vi "ControlProgram5.6 (DON'T USE ME YET!).vi"() -> ()   [LabVIEW 2016]
uses:
  <vilib>/Utility/error.llb/DialogType.ctl
  <vilib>/Utility/miscctls.llb/LVPoint32TypeDef.ctl
  <vilib>/DAQmx/write.llb/DAQmx Write (Digital Bool 1Line 1Point).vi
  <vilib>/DAQmx/create/channels.llb/DAQmx Create Channel (DO-Digital Output).vi
  <vilib>/platform/TimedLoop/XDataNode/XDataNode.xnode
  <vilib>/Platform/TimedLoop/XDataNode/nitl_modes.ctl
  <vilib>/Platform/TimedLoop/XDataNode/XDNodeRunTimeDep.lvlib
  <vilib>/Platform/TimedLoop/XDataNode/wakeup.ctl
  <vilib>/Platform/TimedLoop/XDataNode/timing_clust.ctl
  <vilib>/DAQmx/create/channels.llb/DAQmx Create Channel (AI-Voltage-Basic).vi
  <vilib>/DAQmx/create/channels.llb/DAQmx Create Channel (AO-Voltage-Basic).vi
  <vilib>/DAQmx/write.llb/DAQmx Write (Analog 1D DBL NChan 1Samp).vi
  <resource>/objmgr/daqmx.rc
  <vilib>/Analysis/NI_AALBase.lvlib
  <vilib>/Analysis/baseanly.llb/Mean (DBL).vi
  <vilib>/Instr/_visa.llb/VISA Configure Serial Port (Instr).vi
  <vilib>/Utility/inputDevices.llb/closeMouse.vi
  <vilib>/Utility/inputDevices.llb/mouseAcquire.vi
  <vilib>/DAQmx/read.llb/DAQmx Read (Analog 2D DBL NChan NSamp).vi
  <vilib>/DAQmx/configure/timing.llb/DAQmx Timing (Sample Clock).vi
  <vilib>/addons/control/pid/NI_PID_pid.lvlib
  <vilib>/addons/control/pid/pid.llb/PID (DBL).vi
panel:
  in  "Save file index":dbl=15.0
  out "Flush Sample Start Time":u32=2285218960
  out "Sample flush time (s)":dbl=48.0
  in  "Inject Sample":bool=TRUE
  out "Chart Freq (Hz)":dbl=500.0
  out "Cal values":T1={"AX alpha"=667.4214819429142, "BX alpha"=606.5152707209702, "AX kappa"=0.3417228871032801, "BX kappa"=0.33057762801553825, "AX offset"=-0.04779405741665418, "BX offset"=-0.14093899580105926, "AY alpha"=584.7548506445179, "BY alpha"=581.5659074854012, "AY kappa"=0.3795559926341009, "BY kappa"=0.3493562572212465, "AY offset"=-0.01291651645056598, "BY offset"=-0.10407020663314887}
  in  "Inject Pump 1":bool
  in  "Inject Pump 2":bool
  in  "Tab Control 2":T2(tab)=enum."Fish"
  in  "Force FB script":bool
  in  "Got ADig bead":bool
  in  "Move Cap. 2 (ADig Top)":bool
  in  "Dump beads":bool
  in  "Got DNA bead":bool
  in  "Flow on\ncap 2?":bool=TRUE
  in  "Flow on\ncap 1?":bool=TRUE
  in  "Flow on\ndump?":bool=TRUE
  in  "Fish After TA?":bool=TRUE
  in  "Delta after tether":dbl=1650.0
  in  "TA Cancel Save?":bool=TRUE
  in  "Min fish\ndelta (nm)":dbl=1200.0 min=0.0 max=5000.0 step=25.0
  in  "Max fish\ndelta (nm)":dbl=1900.0 min=0.0 max=5000.0 step=25.0
  in  "Fish Speed (ms)":i32=5000
  in  "Wait (ms)":i32=1500
  in  "# attempts":dbl=10.0
  in  "Cutoff force (pN)":dbl=4.5
  in  "Raster after\n tether?":bool=TRUE
  out "Tether":bool
  out "Attempt #":i32=9
  in  "Flow on\nwhile fish?":bool=TRUE
  in  "Flow on\nafter raster?":bool=TRUE
  in  "Offset @ Delta (nm)":dbl=1600.0
  in  "Cal @ Delta (nm)":dbl=2500.0
  in  "Cal stage position":i32=3
  out "Cal Final Sampling Rate":dbl=125000.0
  in  "Cal Averaging":i32=1
  in  "Wait before dip (s)":dbl=3.0
  in  "Start dipping after?":bool
  in  "Start trap delta (nm)":dbl=1700.0
  in  "Cancel dwell":bool
  in  "Pause dwell":bool
  in  "Return position":dbl=3.0
  in  "Dip duration":dbl=15.0
  in  "Dip position":dbl=4.0
  in  "Dip":bool
  out "Dip time":i32
  in  "Stop":bool=TRUE
  in  "?":T3(tab)
  in  "Save N sets":bool
  in  "N sets":i32=200
  in  "Cal sets to save":i32=500
  in  "Reset data stream":bool
  out "Buffer Overflow":bool
  out "Stage moving":bool
  in  "Comment":string
  in  "Raster scan":bool
  out "Saving":bool
  in  "Save cal":bool
  in  "Save Data":bool
  in  "Stop saving":bool
  out "Calibrating":bool
  out "Progress":dbl(slide) scale=0.0..100.0
  in  "Read Cal":bool
  in  "Fish":bool
  in  "Averaging Number":i32=1250
  out "Final Sampling Rate":dbl=100.0
  in  "Trap position (V)":cluster{"X":dbl, "Y":dbl}={"X"=3.2129837352776223, "Y"=1.95}
  in  "Trap delta (nm)":dbl=1750.0 min=0.0 max=5000.0 step=50.0
  in  "Fixed X":dbl=1.25
  in  "Fixed Y":dbl=1.95
  in  "Shutter 1 (B)":bool
  in  "Shutter 2 (A)":bool
  in  "Pulling direction":bool
  out "Raster scanning...":bool
  out "Current file name":path=path "D:/data/160307/160307_015.dat"
  in  "AX alpha":dbl=667.4214819429142 format="%#_3p"
  in  "BX alpha":dbl=606.5152707209702 format="%#_3g"
  in  "AX kappa":dbl=0.3417228871032801 format="%#_3g"
  in  "BX kappa":dbl=0.33057762801553825 format="%#_3g"
  in  "AX offset":dbl=-0.04779405741665418 format="%#_3g"
  in  "BX offset":dbl=-0.14093899580105926 format="%#_3g"
  in  "AY alpha":dbl=584.7548506445179 format="%#_3g"
  in  "BY alpha":dbl=581.5659074854012 format="%#_3g"
  in  "AY kappa":dbl=0.3795559926341009 format="%#_3g"
  in  "BY kappa":dbl=0.3493562572212465 format="%#_3g"
  in  "AY offset":dbl=-0.01291651645056598 format="%#_3g"
  in  "BY offset":dbl=-0.10407020663314887 format="%#_3g"
  out "Buffer status":u8(slide) scale=0.0..100.0
  in  "dump spot":string="Dump beads spot"
  in  "up flow spot":string="Upper flow spot"
  in  "low flow spot":string="Lower flow spot"
  in  "up cap":string="Upper capillary (ADig beads)"
  in  "bottom cap":string="Lower capillary (DNA beads)"
  in  "Move to Position 5":bool
  in  "Set Position 5":bool
  in  "Saved stage positions":dbl[][](array[numeric])=[[1.0, 0.0, 0.0, 0.0], [2.0, -0.1188, -3.20907, 0.00068], [3.0, 0.45, -0.73974, 0.0], [4.0, 0.45, -2.1978, 0.0], [5.0, 0.45, -2.63158, -0.02256]]
  in  "Set Position 2":bool
  in  "Move to Position 2":bool
  in  "Set Position 1":bool
  in  "Move to Position 1":bool
  in  "Set Position 4":bool
  in  "Move to Position 4":bool
  in  "Set Position 3":bool
  in  "Move to Position 3":bool
  out "Stage error":errorcluster
  in  "Clear Volume":bool
  out "Sample Flush Meter":u8(slide) scale=0.0..100.0
  out "Flushing Sample":bool
  in  "Flush Sample":bool
  in  "Normal \nRate (ul/hr)  3":dbl=100.0
  in  "Normal \nVolume (ul) 3":dbl=300.0
  in  "Normal \nVolume (ul) 2":dbl
  in  "Normal \nRate (ul/hr)":dbl
  in  "Normal \nVolume (ul)":dbl
  in  "Flush\nRate (ul/min)":dbl
  in  "Flush\nVolume (ul)":dbl
  in  "Flush \nRate (ul/min)  2":dbl
  in  "Flush Pump 2":bool
  in  "Flush\nVolume (ul)  2":dbl
  in  "Flush Pump 1":bool
  in  "Normal \nRate (ul/hr)  2":dbl
  in  "Write Wait":i32=1000
  in  "Flush \nRate (ul/min)  3":dbl=100.0
  in  "Flush\nVolume (ul)  3":dbl=80.0
  out "error out":errorcluster
  in  "Use Mouse to Move Trap?":bool
  in  "Pause Mouse/Mirror Connection":bool
  out "Reference Voltage":cluster{dbl, dbl}={0.0, -0.0}
  out "Saved voltage":cluster{dbl, dbl}={5.766666666666665, 1.45}
  out "Real Coordinates":cluster{"Horizontal":i32, "Vertical":i32}={"Horizontal"=897, "Vertical"=-1271}
  out "CoordinatesMousePressed":T4
  in  "Initial Delta (nm)":dbl=1600.0
  in  "Desired Force (pN)":dbl
  out "Sum error":dbl(knob)=1.0 scale=-10.0..10.0
  out "Trap sep":waveform(dbl)[](graph)=[{"t0"=timestamp(168.60999999999163 s since 1904-01-01), "dt"=0.002, "Y"=[1750.8033268895808, 1750.6596979359072, 1750.70221210613, 1750.6907217899675, 1750.7631107826903], "attributes"=variant("NI_ChannelName"=variant(string "T2 X"))}, {"t0"=timestamp(168.60999999999163 s since 1904-01-01), "dt"=0.002, "Y"=[1.7020764070611287, 1.7327099986985621, 1.667532144120588, 1.7268439918257026, 1.6936032859078953], "attributes"=variant("NI_ChannelName"=variant(string "T2 Y"))}]
  in  "Set Initial Delta":bool
  in  "Offset Y (nm)":dbl format="%0.2f"
  in  "Offset X (nm)":dbl format="%0.2f"
  in  "Remove offsets":bool
  in  "Force Feedback":bool
  in  "Max value X":dbl=10.0 format="%.1f"
  in  "Min value X":dbl format="%0.1f"
  in  "Max value Y":dbl=10.0 format="%.1f"
  in  "Min value Y":dbl format="%.1g"
  in  "PID gains":cluster{"Kprop":dbl, "Kint":dbl}={"Kprop"=1.0, "Kint"=0.5}
  out "Mean Trap Pos X 2 (nm)":dbl=1750.7238139008552 format="%0.2f"
  out "Mean Trp Pos Y 2 (nm)":dbl=1.7045531655227752 format="%0.2f"
  out "T2 X RMS (A)":dbl=0.5203679966642587 format="%0.2f"
  out "T2 Y RMS (A)":dbl=0.2360626363266869 format="%0.2f"
  in  "reinitialize error":bool
  in  "Scan range (nm)":dbl=450.0
  in  "Scan speed (nm/s)":dbl=100.0 min=0.0 max=100.0
  in  "Step size (nm)":dbl=1.0
  in  "Save scans":bool=TRUE
  in  "# scans":i32=1
  in  "Load param":bool
  in  "Scan Parameters":T5(array[cluster])=[{"Label"="Offset", "Max delta 2"=3.8, "Start delta 2"=2.4, "Speed (ms) 2"=10000, "# scans 2"=1}]
  in  "Trap delta\nafter (nm)":dbl=1750.0
  in  "Stop raster":bool
  out "Scan range (V)":dbl=0.5047672462142456
  out "Scan steps (mirror)":u64=450
  out "Scan increment (V)":dbl=0.0011217049915872126
  out "Time per step (ms)":dbl=10.0
  out "Total raster time (s)":dbl=9.0
  out "N sets to be saved":dbl=900.0
  out "Continue to display?":bool
  out "Video Error":errorcluster
  in  "# Samples/channel (in)":i32=40000 format="%.2f"
  out "Buffer size\n(Samples/channel)":u32=511
  out "DAQ rate\n(Samples/s)":dbl=125000.0 format="%#_6p"
  out "# Samples/channel":i32=1250
  out "# Samples/channel/s":dbl=100.0
  out "AvailSampPerChan":u32=9
  out "Data update period (s/set)":dbl=0.01 format="%#_6p"
  out "AvailSampPerChan 2":u32=110
  in  "PC samp per channel":i32=1000
  in  "Sampling Rate":dbl=125000.0 format="%0.0p"
  in  "DAQ Rate2":dbl=1000000.0 format="%#_6p"
  out "Data period (s)":dbl=8e-06 format="%#_6p"
  in  "Tether break\nforce (pN)":dbl=1.0
  in  "Path":path=path "D:/data"
  out "Mirror task":refnum<k21>
  in  "Conv X (nm/V)":dbl=891.5
  in  "Conv Y (nm/V)":dbl=505.7
  in  "HWP1":string="Half waveplate 1: differential trap power"
  in  "HWP0":string="Half waveplate 0: total trap power"
  in  "Move 1":bool
  in  "\"Degrees\" 1":dbl
  in  "Move 0":bool
  in  "\"Degrees\" 0":dbl
  out "Chamber":T6(plugin-control)
  out "Deflection":T4
  in  "Sampling Rate":dbl=125000.0 format="%0.2f"
  in  "Averaging Number":i32=12500
  in  "DAQ Rate":dbl=1000000.0
  out "Final Sampling Rate":dbl
  in  "Tab Control":T7(tab)
  in  "Downsamp\nfact":dbl=250.0
  out "Bead sep":waveform(dbl)[](graph)=[{"t0"=timestamp(168.60999999999163 s since 1904-01-01), "dt"=0.002, "Y"=[4727.160732188745, 4710.814328126384, 4662.047898916555, 4830.411717025629, 4760.584350916598], "attributes"=variant("NI_ChannelName"=variant(string "T2"))}, {"t0"=timestamp(168.60999999999163 s since 1904-01-01), "dt"=0.002, "Y"=[1461.5383672767387, 1524.4661096393045, 1544.3945198290342, 1457.2660645927294, 1236.1675333616608], "attributes"=variant("NI_ChannelName"=variant(string "T1"))}]
  out "Force (pN)":waveform(dbl)[](graph)=[{"t0"=timestamp(168.60999999999163 s since 1904-01-01), "dt"=0.002, "Y"=[1615.882480725656, 1610.392258295866, 1593.6702564391426, 1651.2708223052214, 1627.3736257823707], "attributes"=variant("NI_ChannelName"=variant(string "T2"))}, {"t0"=timestamp(168.60999999999163 s since 1904-01-01), "dt"=0.002, "Y"=[510.5070285449429, 532.3366054605332, 539.4905656260677, 508.8600257300396, 431.67642791906815], "attributes"=variant("NI_ChannelName"=variant(string "T1"))}]
  out "Mean force (pN)":dbl=1062.1460096828907 format="%0.2f"
  out "Force noise (pN)":dbl=17.268335299694712 format="%0.2f"
  out "Mean Bead Sep\n(nm)":dbl=3091.4851621873377 format="%0.2f"
  out "Bead Sep Noise\n(A)":dbl=494.77805668581857 format="%0.2f"
  out "PSD 2":cluster{dbl[], dbl[]}(graph)
  out "PSD 1":cluster{dbl[], dbl[]}(graph)
  out "PSD 1 Sum":dbl(slide) scale=0.0..10.0
  out "PSD 2 Sum":dbl(slide) scale=0.0..10.0
  in  "Start":bool
  out "All signals":waveform(dbl)[](graph)=[{"t0"=timestamp(168.60999999999163 s since 1904-01-01), "dt"=0.002, "Y"=[0.0011821860798437312, 0.001312633777410628, 0.001242511697769595, 0.0012914940322799955, 0.0012690652725783874], "attributes"=variant("NI_ChannelName"=variant(string "A y"))}, {"t0"=timestamp(168.60999999999163 s since 1904-01-01), "dt"=0.002, "Y"=[0.019556422473767078, 0.01991399362970228, 0.019693830876328172, 0.01969460427040848, 0.019782772493313613], "attributes"=variant("NI_ChannelName"=variant(string "A x"))}, {"t0"=timestamp(168.60999999999163 s since 1904-01-01), "dt"=0.002, "Y"=[-0.0013630908745525172, -0.0015559266057216816, -0.001497405596047725, -0.0014656959822427578, -0.0013483961720842275], "attributes"=variant("NI_ChannelName"=variant(string "B y"))}, {"t0"=timestamp(168.60999999999163 s since 1904-01-01), "dt"=0.002, "Y"=[0.00015941436024671937, 0.0002339190787486881, 0.00014781328468225978, 0.00022773183412498586, 0.000218450970001253], "attributes"=variant("NI_ChannelName"=variant(string "B x"))}, {"t0"=timestamp(168.60999999999163 s since 1904-01-01), "dt"=0.002, "Y"=[-0.002746279049062249, -0.002806855193752219, -0.0028042774852306703, -0.002707613423611985, -0.0027591675907931747], "attributes"=variant("NI_ChannelName"=variant(string "A sum"))}, {"t0"=timestamp(168.60999999999163 s since 1904-01-01), "dt"=0.002, "Y"=[-0.0005668266999084266, -0.000620958572545292, -0.0005874483653747573, -0.000613225446732485, -0.0006699350304745015], "attributes"=variant("NI_ChannelName"=variant(string "B sum"))}, {"t0"=timestamp(168.60999999999163 s since 1904-01-01), "dt"=0.002, "Y"=[3.213884831059541, 3.2137237217452688, 3.213771410102221, 3.2137585213572266, 3.2138397204516997], "attributes"=variant("NI_ChannelName"=variant(string "Trap x"))}, {"t0"=timestamp(168.60999999999163 s since 1904-01-01), "dt"=0.002, "Y"=[1.9533657828891855, 1.9534263594991073, 1.9532974730949586, 1.9534147597228113, 1.9533490276565313], "attributes"=variant("NI_ChannelName"=variant(string "Trap y"))}]
  # "Bead Calibration"
  # "Y"
  # "X"
  # "Pump #1 Controls"
  # "Pump #2 Controls"
  # "Sample Pump Controls"
  # "Retract the pumps manually. Change it back to INFUSE when you're done. Suck it up, don't whine."
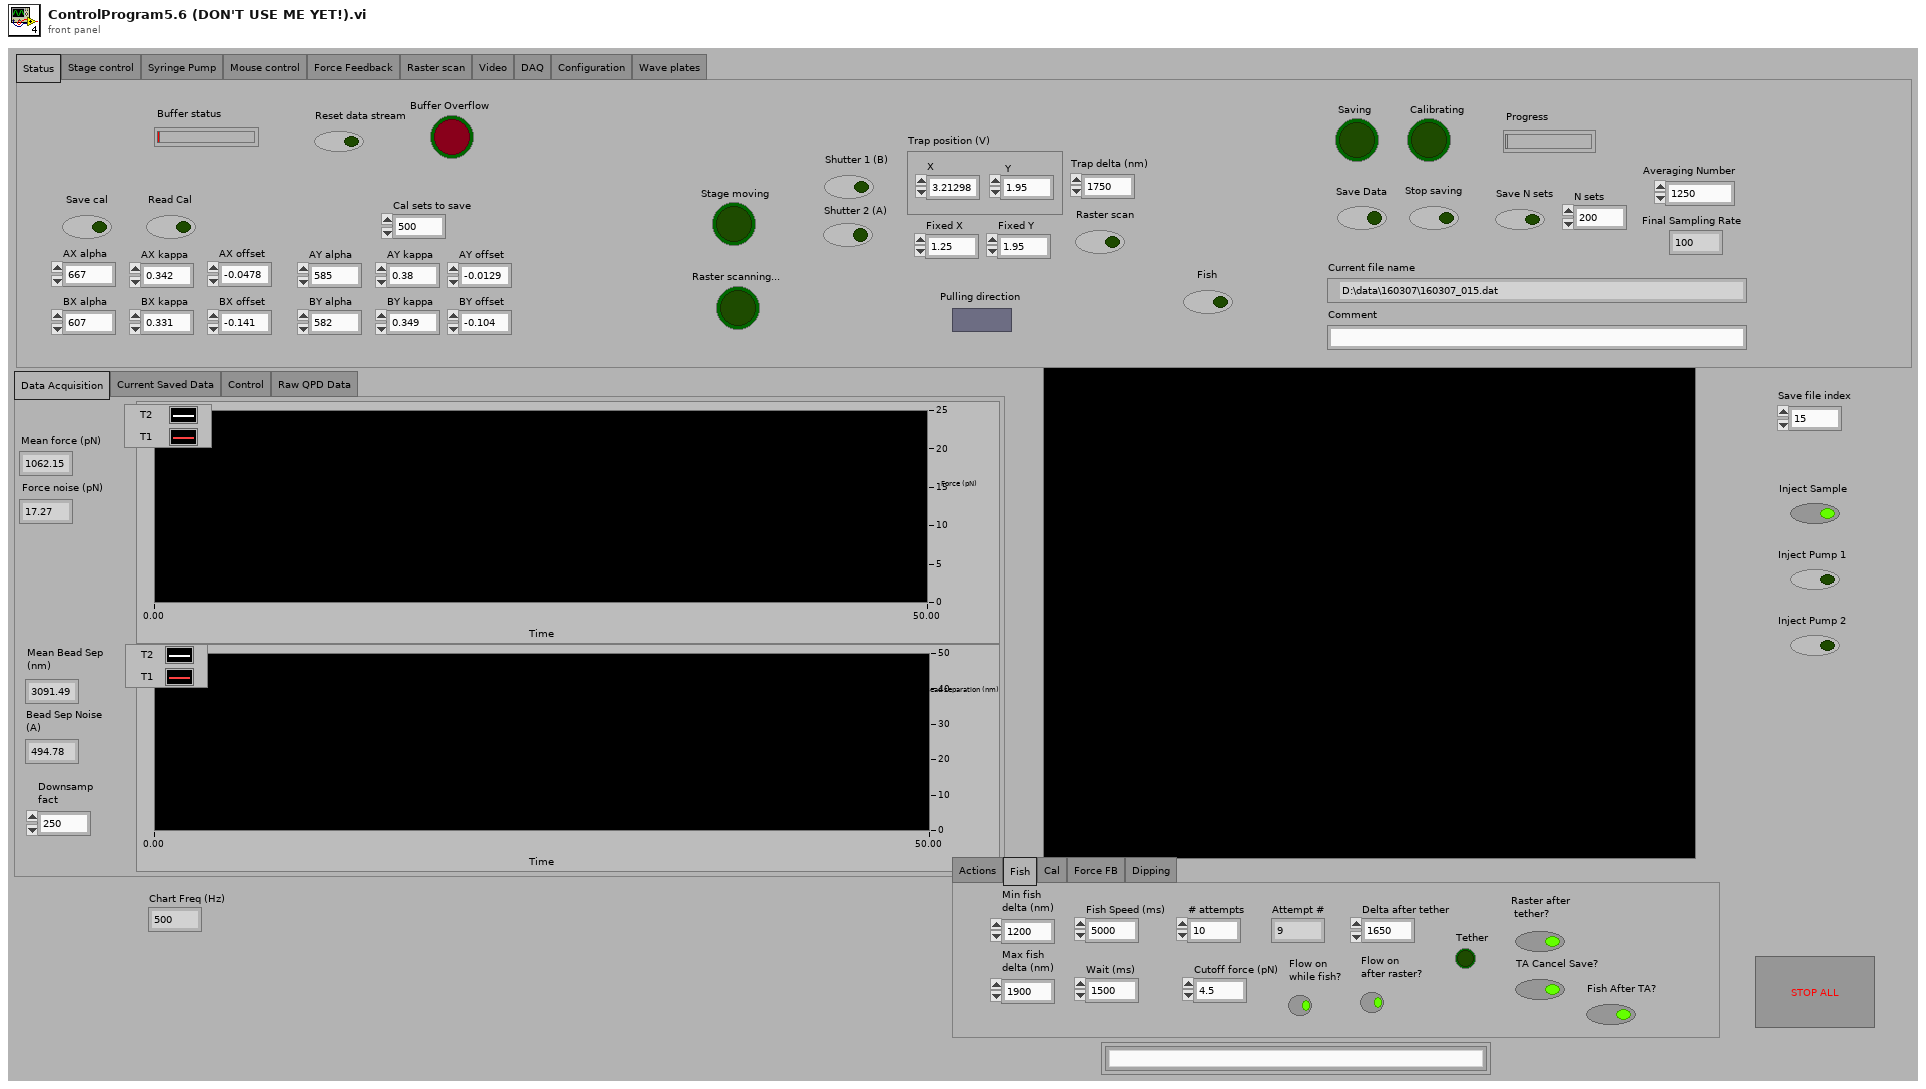
[diagram p1: front panel]
types:
  T1 = cluster{"AX alpha":dbl, "BX alpha":dbl, "AX kappa":dbl, "BX kappa":dbl, "AX offset":dbl, "BX offset":dbl, "AY alpha":dbl, "BY alpha":dbl, "AY kappa":dbl, "BY kappa":dbl, "AY offset":dbl, "BY offset":dbl}
  T2 = enum32{"Actions", "Fish", "Cal", "Force FB", "Dipping"}
  T3 = enum32{"Status", "Stage control", "Syringe Pump", "Mouse control", "Force Feedback", "Raster scan", "Video", "DAQ", "Configuration", "Wave plates"}
  T4 = typedef "LVPoint32TypeDef.ctl" = cluster{"Horizontal":i32, "Vertical":i32}
  T5 = cluster{"Label":string, "Max delta 2":dbl, "Start delta 2":dbl, "Speed (ms) 2":i32, "# scans 2":i32}[]
  T6 = typedef "IMAQ Image.ctl" = refnum<image>
  T7 = enum32{"Data Acquisition", "Current Saved Data", "Control", "Raw QPD Data"}
  T8 = enum16{"open", "replace", "create", "open or create", "replace or create", "replace or create with confirmation"}
  T9 = enum16{"big-endian, network order", "native, host order", "little-endian"}
  T10 = cluster{string, string, string, string, string, string, string, string}
  T11 = typedef "XDNodeRunTimeDep.lvlib/timing_clust.ctl" = cluster{"Expected End [f-1]":u64, "Actual End [f-1]":u64, "Finished Late? [f-1]":bool, "Expected End [i-1]":u64, "Actual End [i-1]":u64, "Finished Late? [i-1]":bool, "Expected Start [i]":u64, "Actual Start [i]":u64, "Expected Start [f]":u64, "Actual Start [f]":u64, "Source Name":string, "Structure Name":string, "Period":i64, "Deadline":i64, "Offset":i64, "Start":i64, "Priority":i32, "Timeout":i32, "Mode":T12, "Wakeup Reason":T13, "Error":errorcluster, "Source Type":string, "Secondary Source Type":string, "Global End Time":u64, "Global Start Time":u64, "Frame Duration":u64, "Iteration Duration":u64, "Assigned CPU":i32, "I/O Scan Engine Mode":u32}
  T12 = typedef "XDNodeRunTimeDep.lvlib/nitl_modes.ctl" = enum32{"No Change", "Process missed periods, maintain original phase", "Discard missed periods, maintain original phase", "Process missed periods, ignore original phase", "Discard missed periods, ignore original phase"}
  T13 = typedef "XDNodeRunTimeDep.lvlib/wakeup.ctl" = enum32{"Normal", "Aborted", "Asynchronous wakeup", "Timing source error", "Timed loop error", "Timeout"}
  T14 = typedef "DialogType.ctl" = u16
  T15 = cluster{"button 1":bool, "button 2":bool, "button 3":bool, "button 4":bool}
  T16 = cluster{"[0]":dbl, "[1]":dbl, "[2]":dbl, "[3]":dbl, "[4]":dbl, "[5]":dbl, "[6]":dbl, "[7]":dbl, "[8]":dbl, "[9]":dbl, "[10]":dbl, "[11]":dbl}
  T17 = cluster{"Label":string, "Max delta 2":dbl, "Start delta 2":dbl, "Speed (ms) 2":i32, "# scans 2":i32}
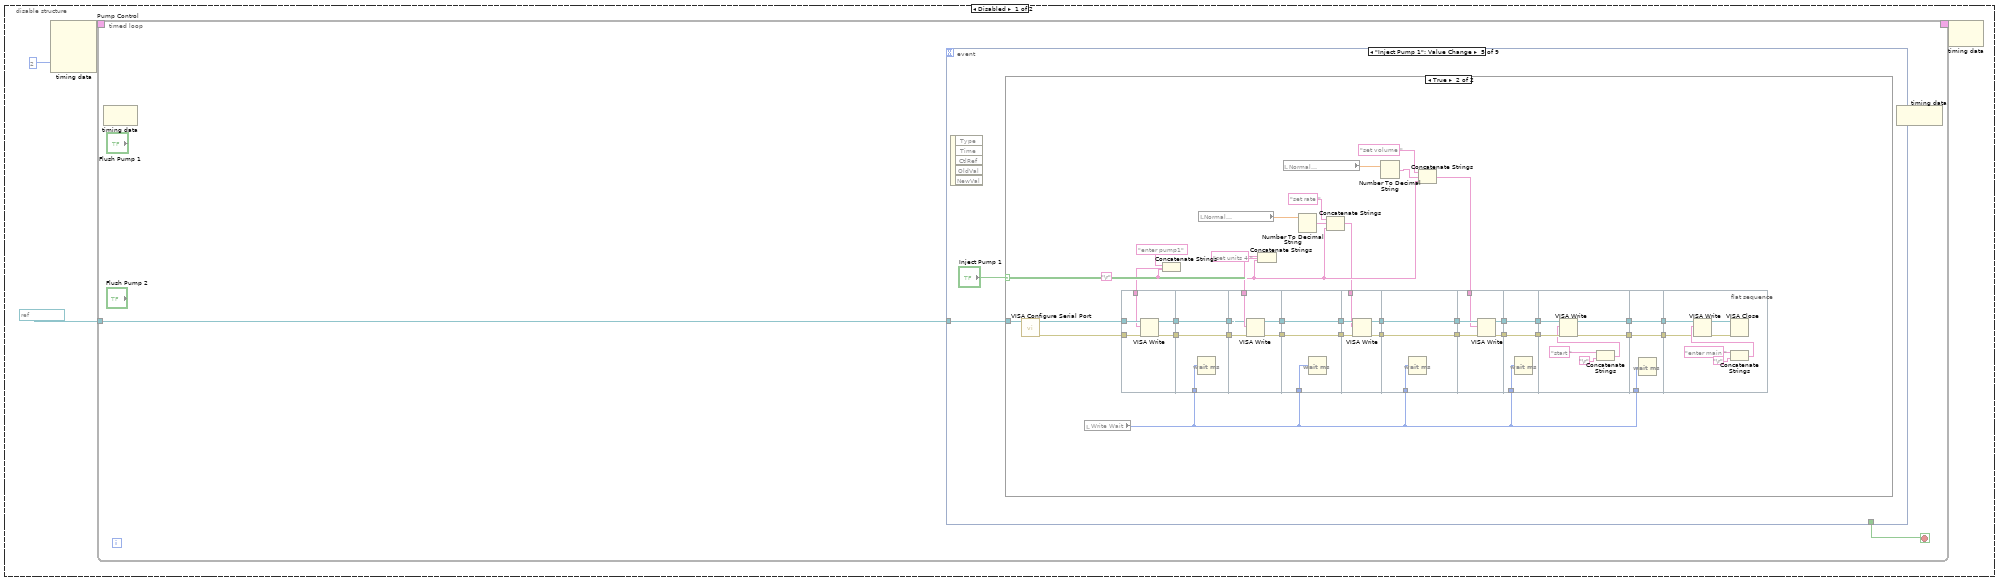
[diagram p2: hidden frame]
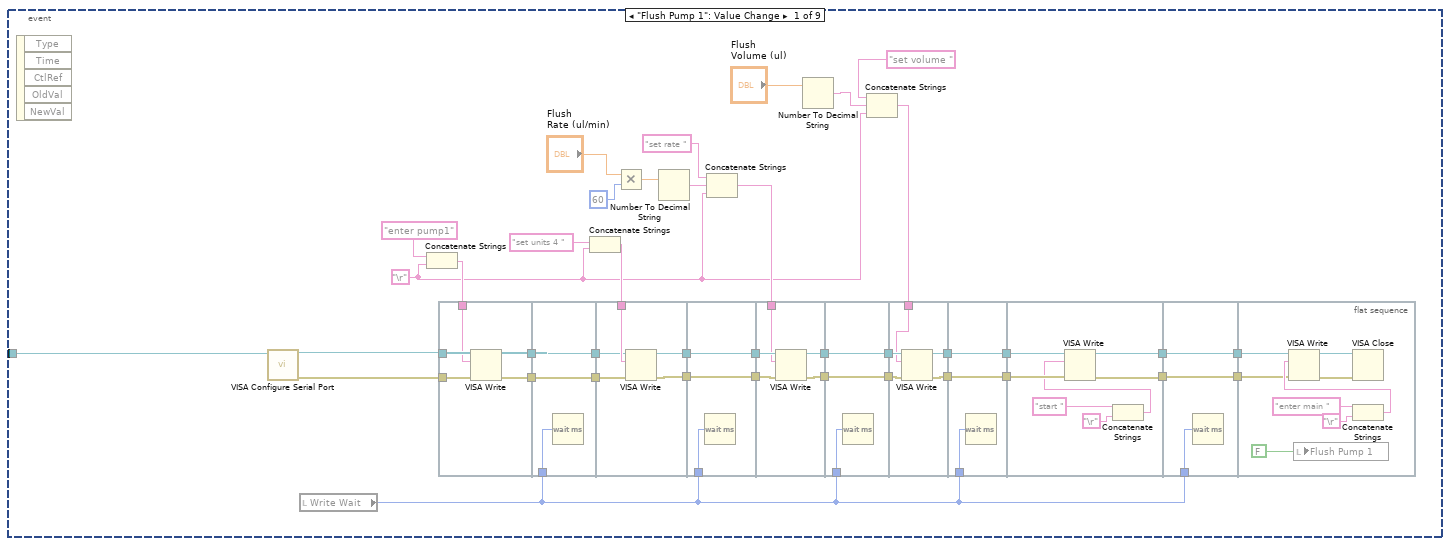
[diagram p3: hidden frame]
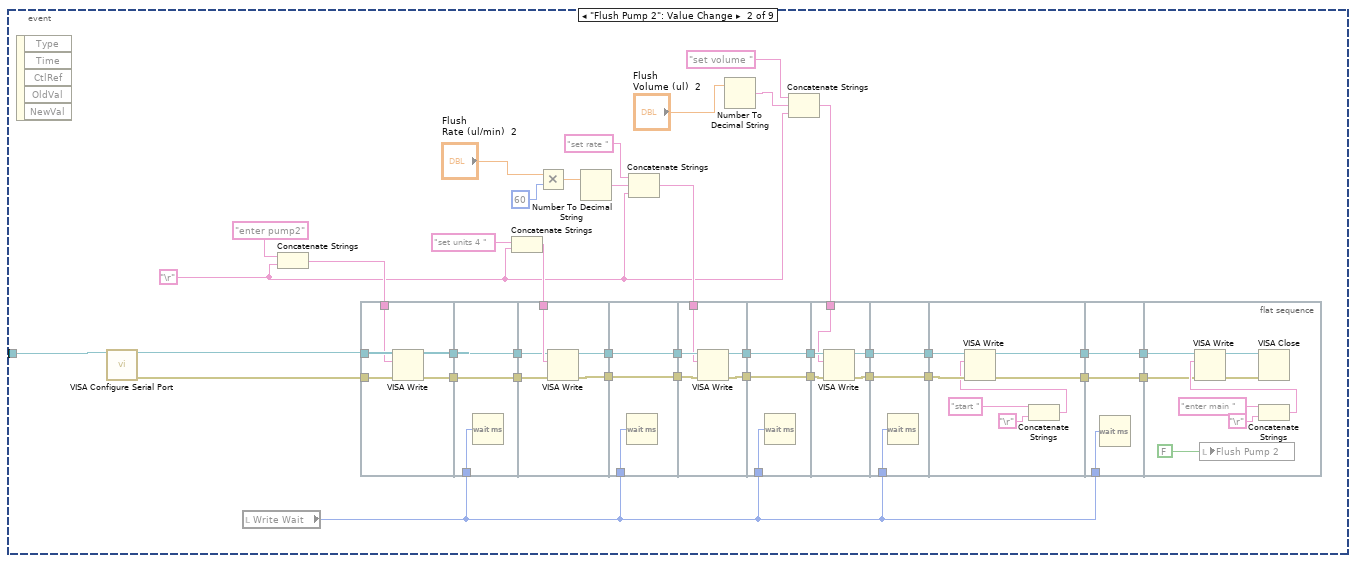
[diagram p4: hidden frame]
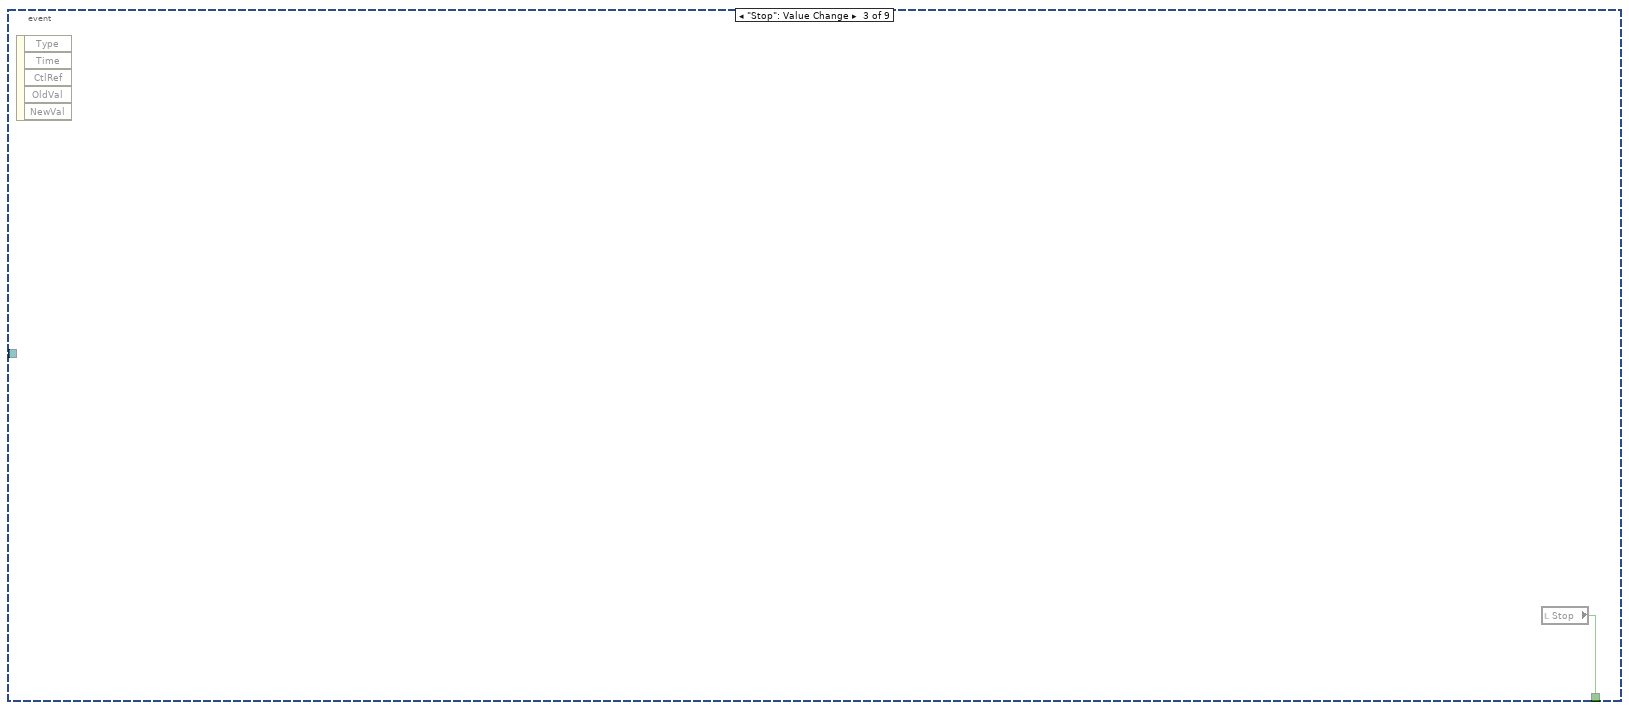
[diagram p5: hidden frame]
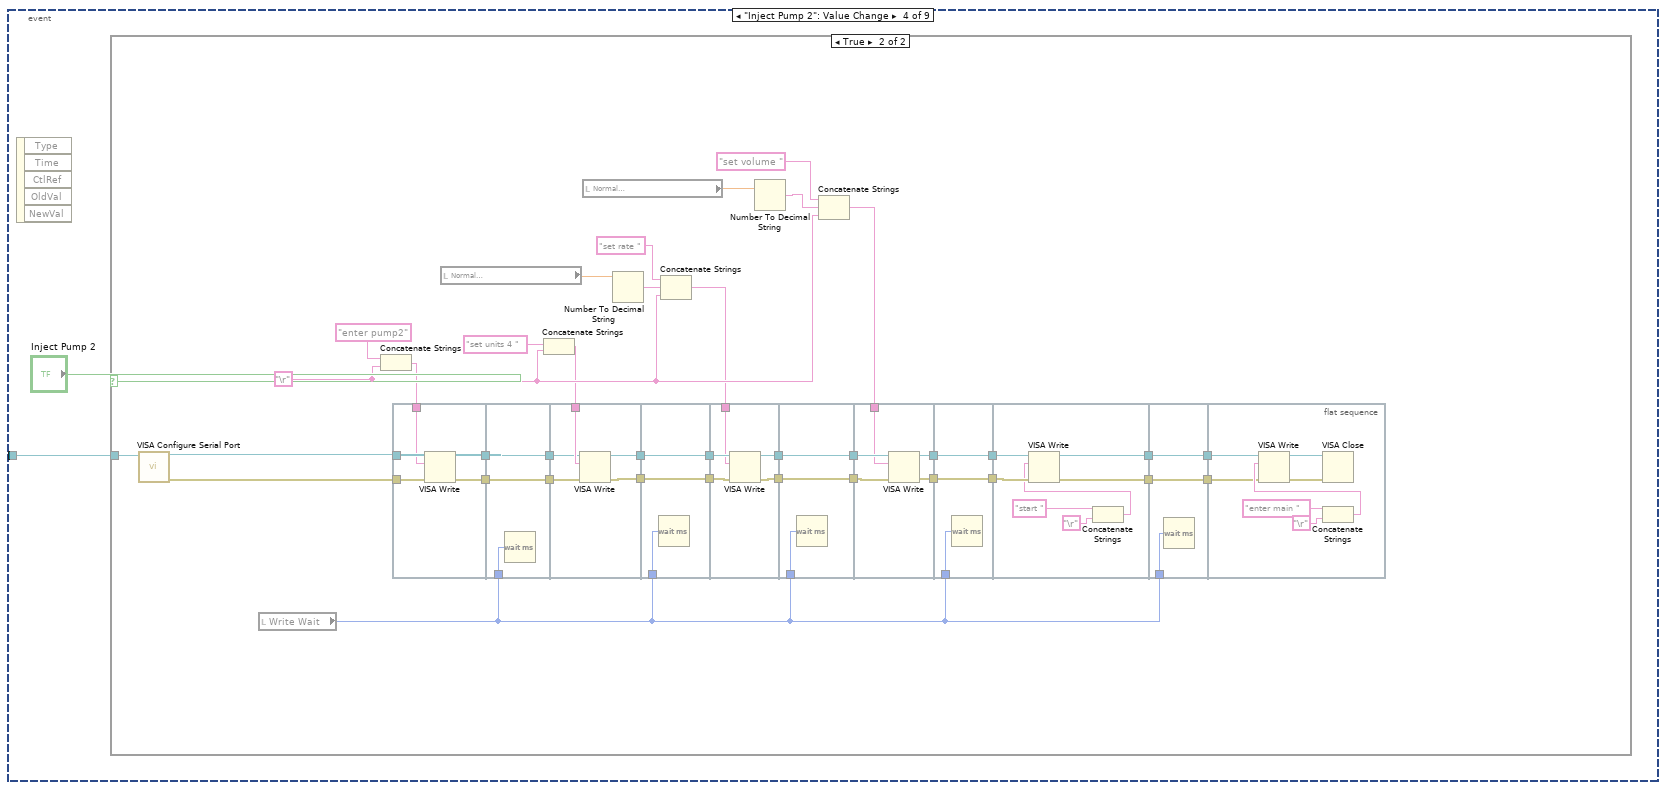
[diagram p6: hidden frame]
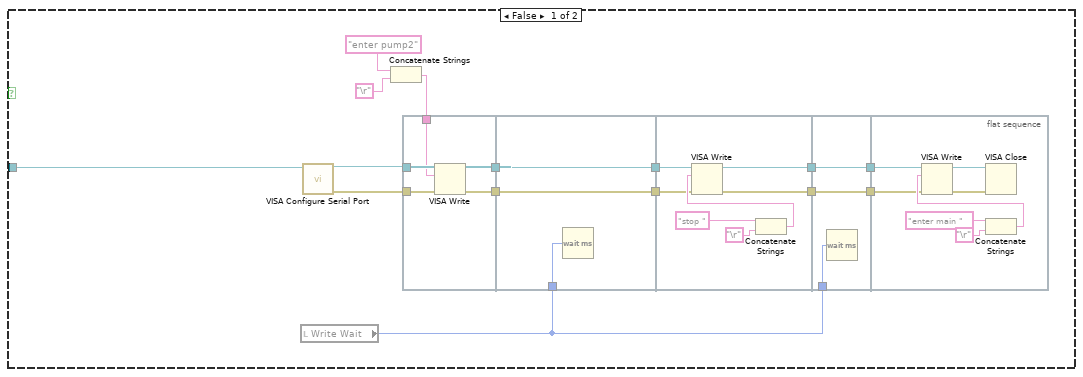
[diagram p7: hidden frame]
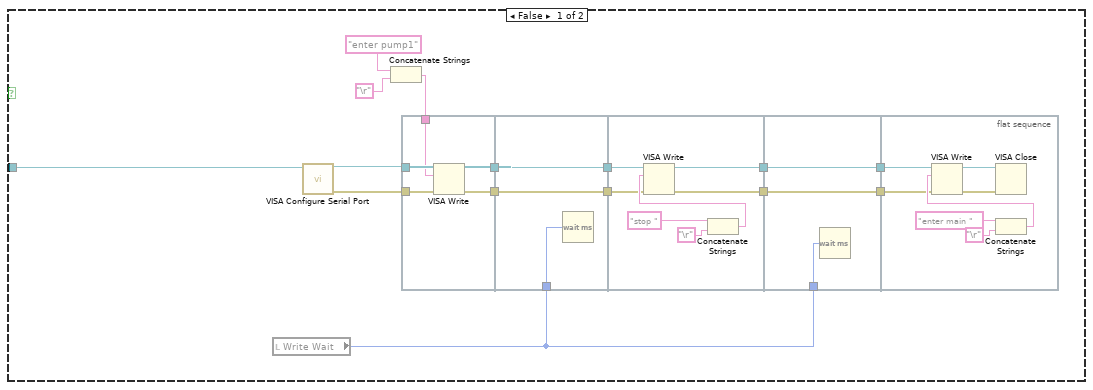
[diagram p8: hidden frame]
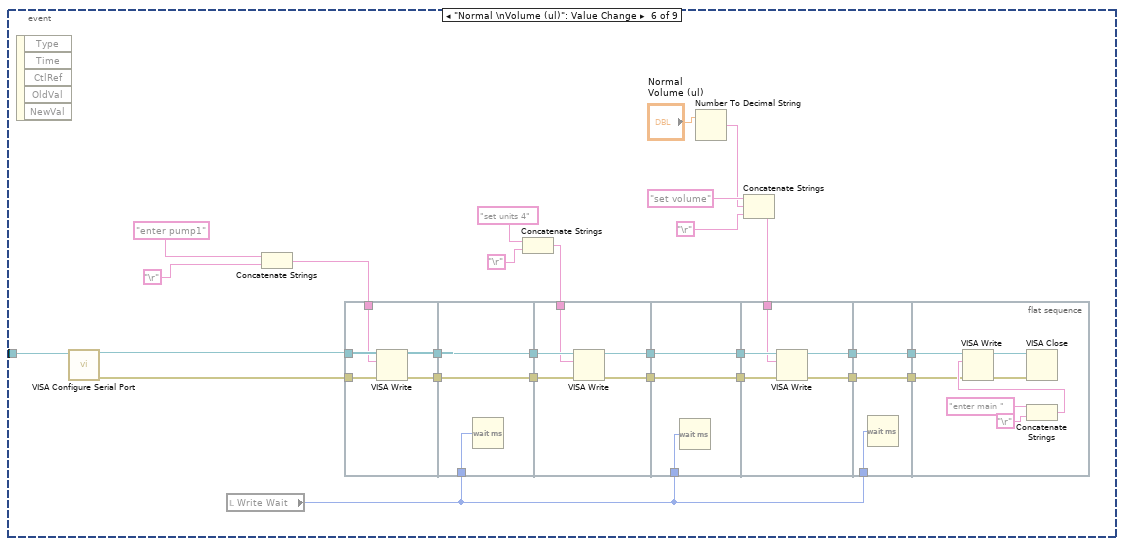
[diagram p9: hidden frame]
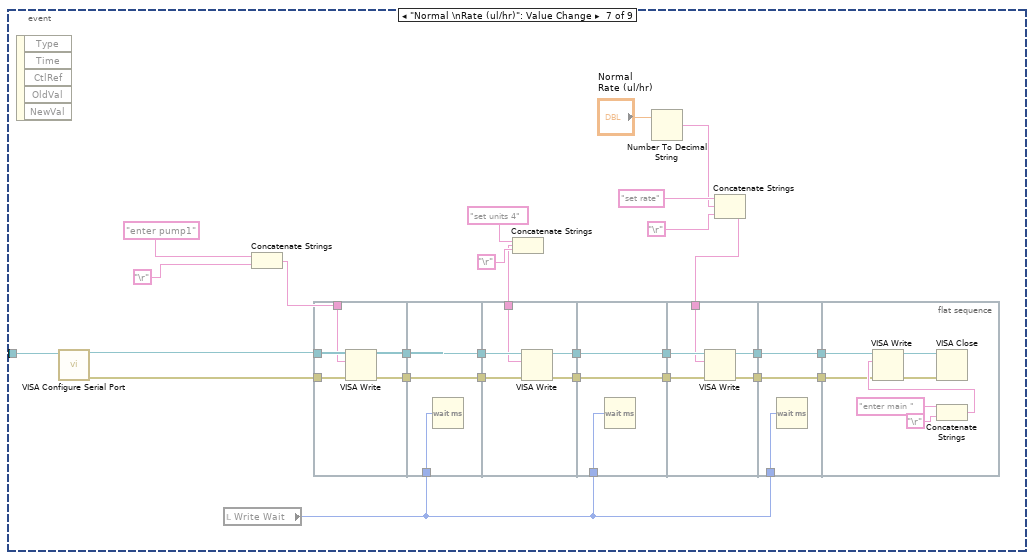
[diagram p10: hidden frame]
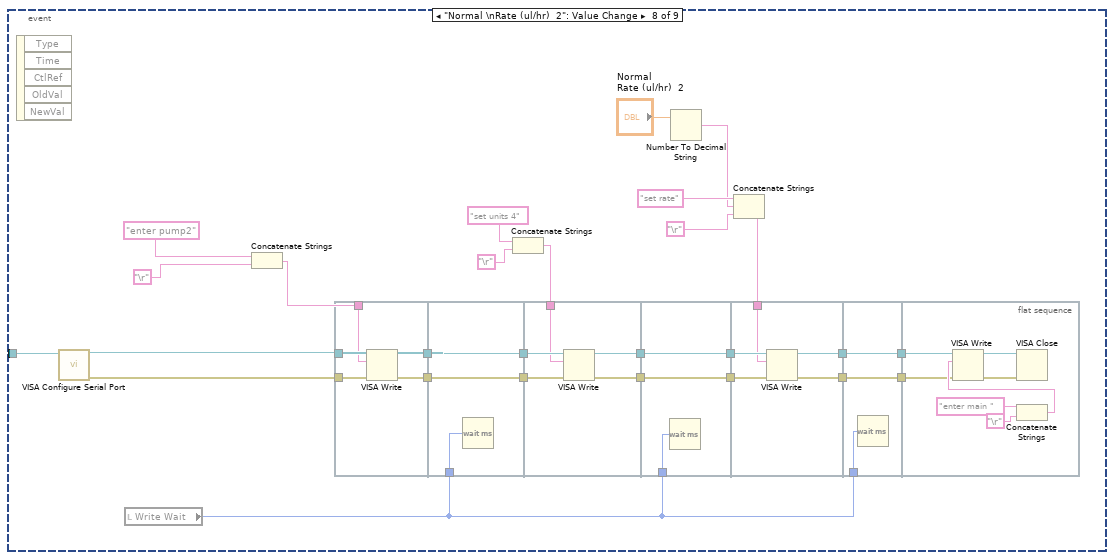
[diagram p11: hidden frame]
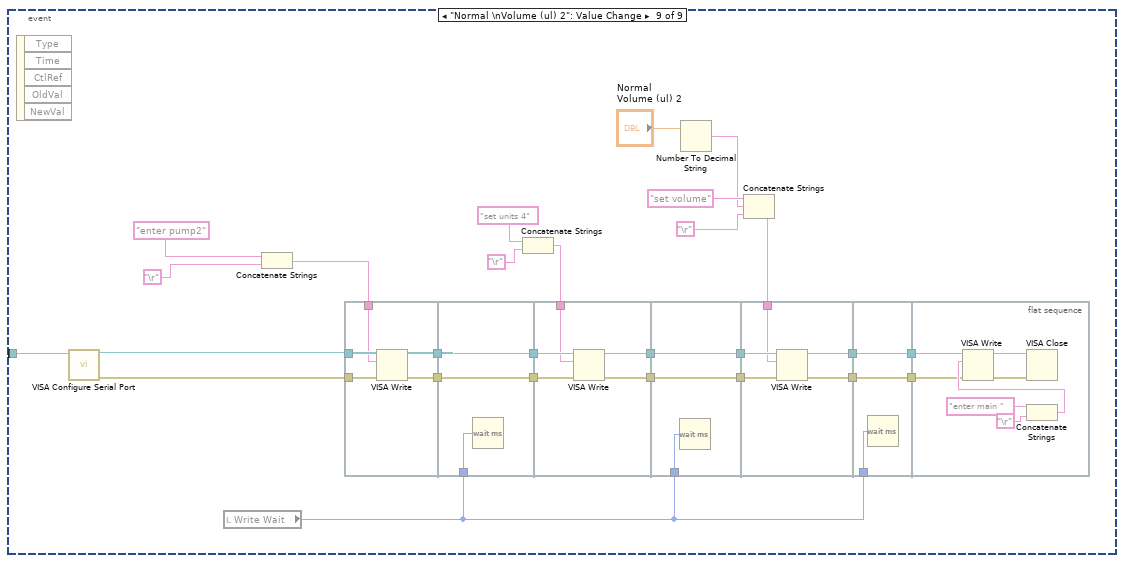
[diagram p12: hidden frame]
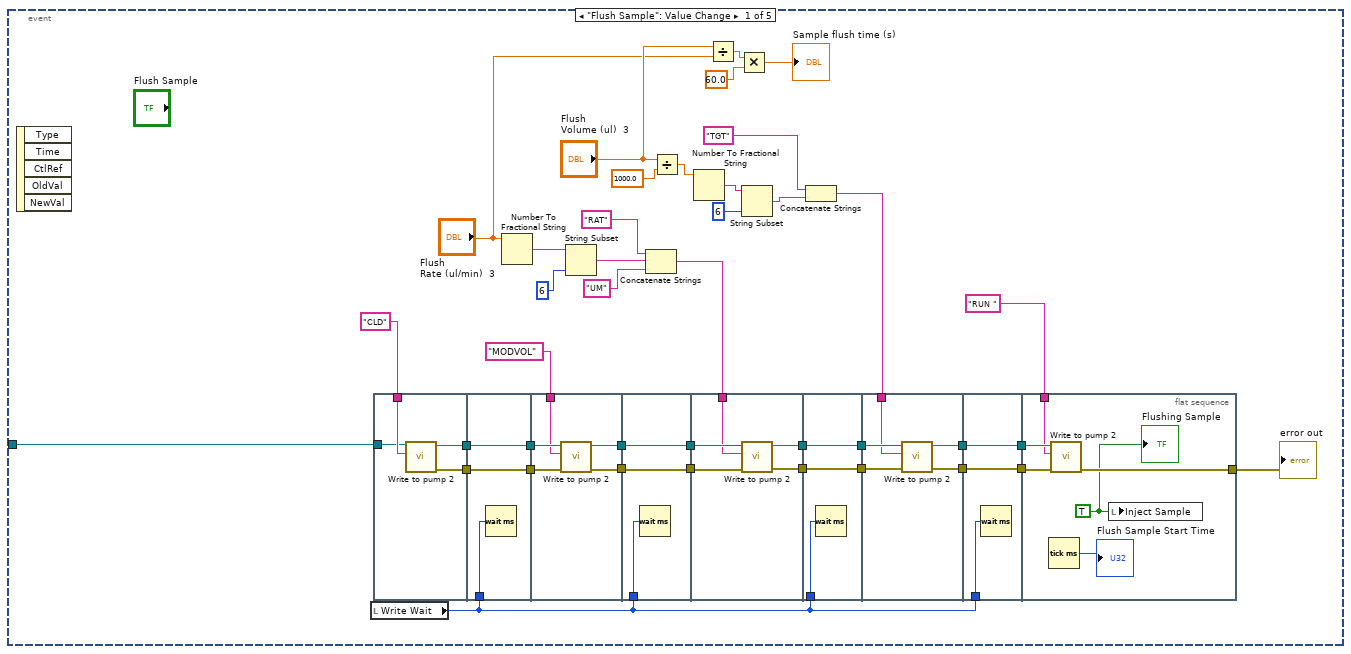
[diagram p13: hidden frame]
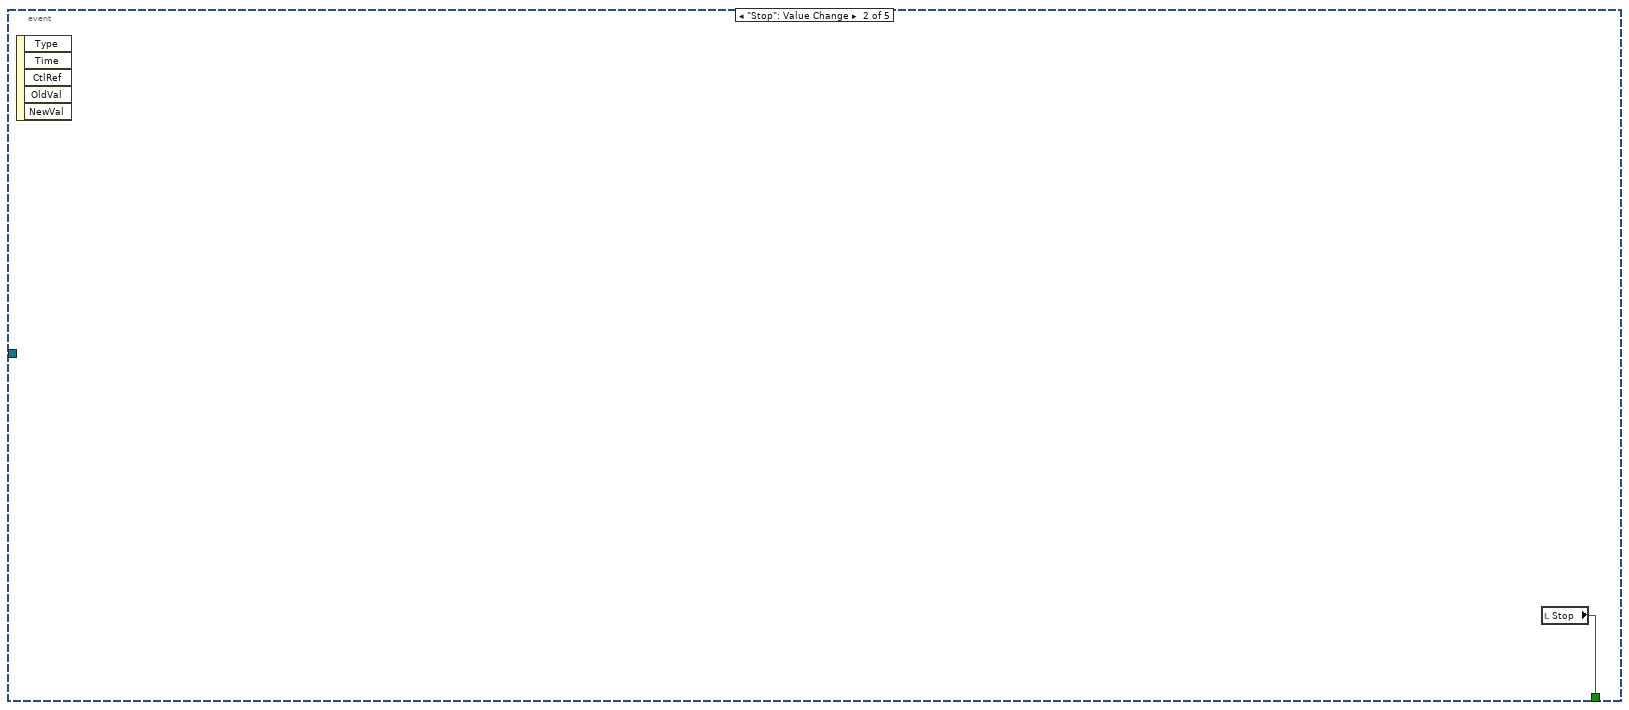
[diagram p14: hidden frame]
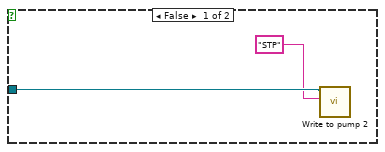
[diagram p15: hidden frame]
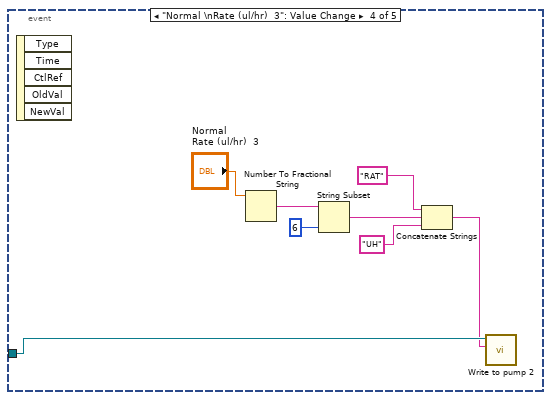
[diagram p16: hidden frame]
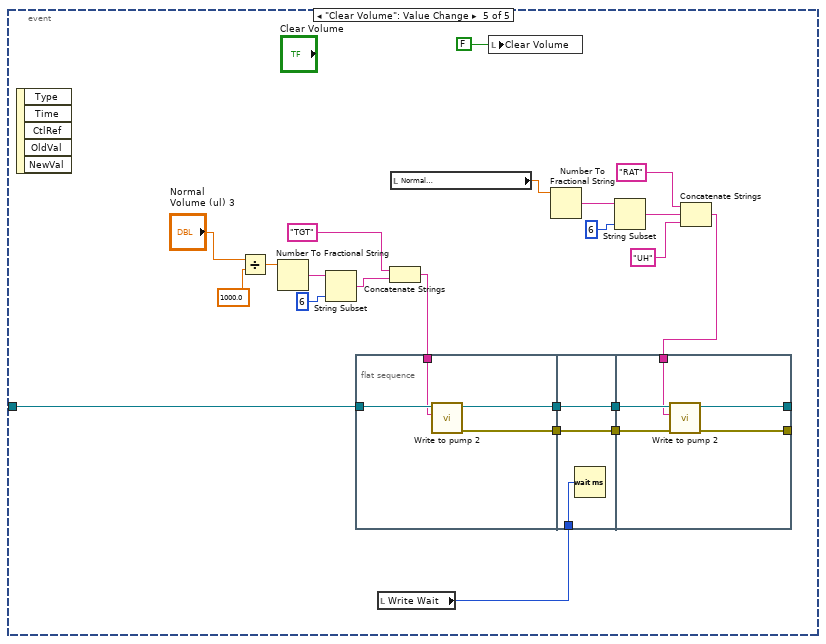
[diagram p17: hidden frame]
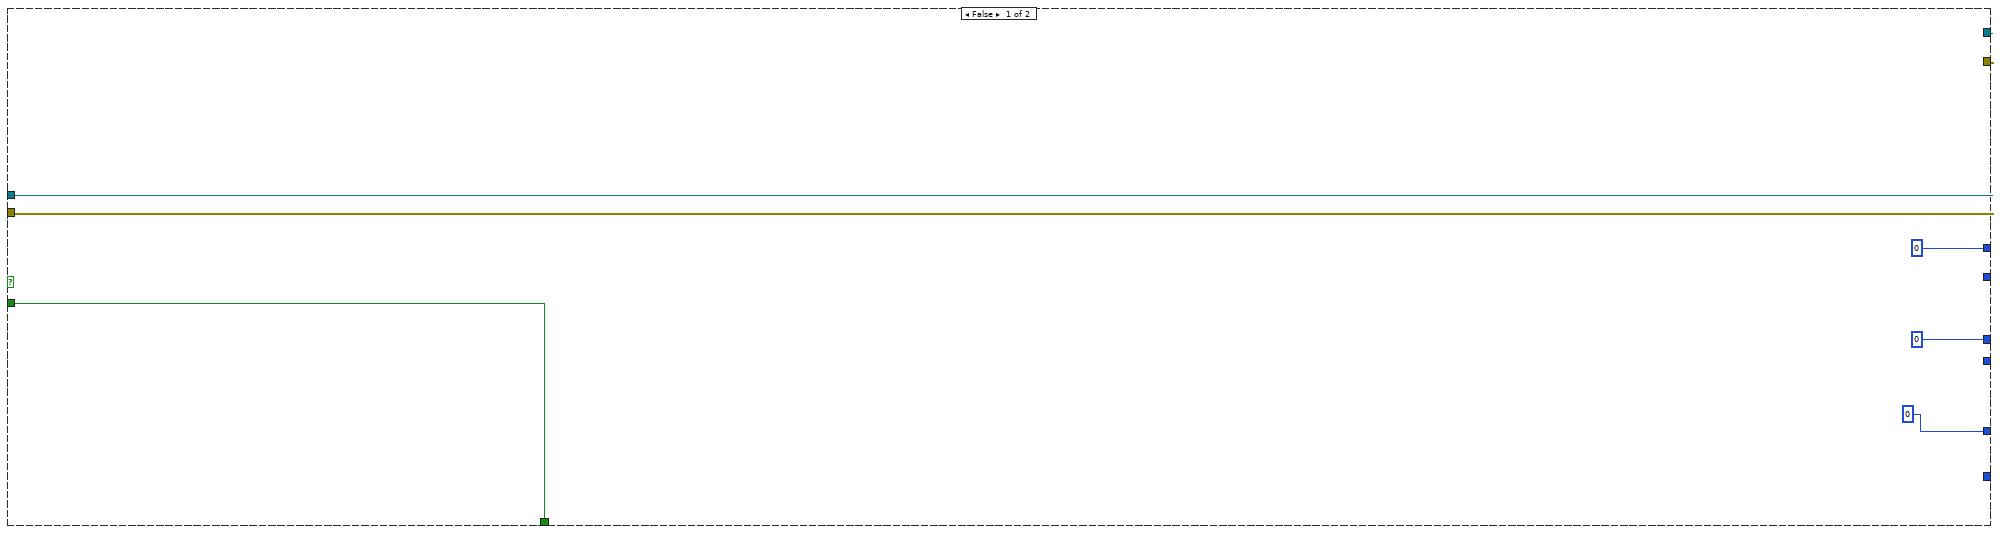
[diagram p20: hidden frame]
diagram:
  w42 = 10.0 ("Minimum Value")
  w43 = -10.0 ("Minimum Value")
  w45 = -2.0 ("Minimum Value")
  w46 = 2.0 ("Maximum Value")
  w71 = 10123 items=["Finite Samples"=10178, "Continuous Samples"=10123] ("sample mode")
  w92 = tag "Dev1/port2/line1"  # Shutter 2
  w95 = tag "Dev1/port1/line4"  # Shutter 1
  # "Create channels for movable mirror"
  # "Create channels for detectors"
  n1 = call-poly <vilib>:"DAQmx Create Virtual Channel.vi"("maximum value"=w46, "minimum value"=w45, "physical channels"=tag "Dev1/ai0" ("Physical Channel")) -> ("task out"=w47:refnum<k21>, "error out"=w70:errorcluster)  [unwired: 11 in]
  n2 = call-poly <vilib>:"DAQmx Create Virtual Channel.vi"("task in"=w47, "maximum value"=w46, "minimum value"=w45, "physical channels"=tag "Dev1/ai1", "error in"=w70) -> ("task out"=w68:refnum<k21>, "error out"=w67:errorcluster)  [unwired: 9 in]
  n3 = call-poly <vilib>:"DAQmx Create Virtual Channel.vi"("task in"=w68, "maximum value"=w46, "minimum value"=w45, "physical channels"=tag "Dev1/ai2", "error in"=w67) -> ("task out"=w59:refnum<k21>, "error out"=w58:errorcluster)  [unwired: 9 in]
  n4 = call-poly <vilib>:"DAQmx Create Virtual Channel.vi"("task in"=w59, "maximum value"=w46, "minimum value"=w45, "physical channels"=tag "Dev1/ai3" ("Physical Channel"), "error in"=w58) -> ("task out"=w44:refnum<k21>, "error out"=w64:errorcluster)  [unwired: 9 in]
  n5 = call-poly <vilib>:"DAQmx Create Virtual Channel.vi"("task in"=w44, "maximum value"=w42, "minimum value"=w43, "physical channels"=tag "Dev1/ai4", "error in"=w64) -> ("task out"=w62:refnum<k21>, "error out"=w61:errorcluster)  [unwired: 9 in]
  n6 = call-poly <vilib>:"DAQmx Create Virtual Channel.vi"("task in"=w62, "maximum value"=w42, "minimum value"=w43, "physical channels"=tag "Dev1/ai5", "error in"=w61) -> ("task out"=w57:refnum<k21>, "error out"=w56:errorcluster)  [unwired: 9 in]
  n7 = call-poly <vilib>:"DAQmx Create Virtual Channel.vi"("task in"=w57, "maximum value"=w42, "minimum value"=w43, "physical channels"=tag "Dev1/ai6", "error in"=w56) -> ("task out"=w51:refnum<k21>, "error out"=w49:errorcluster)  [unwired: 9 in]
  n8 = call-poly <vilib>:"DAQmx Create Virtual Channel.vi"("task in"=w51, "maximum value"=w42, "minimum value"=w43, "physical channels"=tag "Dev1/ai7", "error in"=w49) -> ("task out"=w50:refnum<k21>, "error out"=w48:errorcluster)  [unwired: 9 in]
  n9 = call-poly <vilib>:"DAQmx Timing.vi"("task/channels in"=w50, "sample mode"=w71, "samples per channel"="PC samp per channel", "rate"="Sampling Rate", "error in"=w48) -> ("task out"=w54:refnum<k21>, "error out"=w53:errorcluster)  [unwired: 9 in]
  n10 = call-poly <vilib>:"DAQmx Create Virtual Channel.vi"("maximum value"="Max value Y", "minimum value"="Min value Y", "physical channels"=tag "Dev1/ao1" ("Trap X Axis")) -> ("task out"=w39:refnum<k21>, "error out"=w41:errorcluster)  [unwired: 11 in]
  n11 = property class="DAQmx Timing"(reference=w54, error in=w53, "More:AI Convert:Rate"="DAQ Rate2") -> (reference out=w6:refnum<k21>, error out=w5:errorcluster, "SampClk.Rate"=→"DAQ rate\n(Samples/s)":dbl)
  n12 = call-poly <vilib>:"DAQmx Create Virtual Channel.vi"("task in"=w39, "maximum value"="Max value X", "minimum value"="Min value X", "physical channels"=tag "Dev1/ao0" ("Trap Y Axis"), "error in"=w41) -> ("task out"=w30:refnum<k21>, "error out"=w29:errorcluster)  [unwired: 9 in]
  "Mirror task" <- w30
  n13 = property class="DAQmx Buffer"(reference=w6, error in=w5) -> (reference out=w3:refnum<k21>, error out=w2:errorcluster, "Input.OnbrdBufSize"=→"Buffer size\n(Samples/channel)":u32)
  n14 = call <vilib>:"DAQmx Start Task.vi"("task/channels in"=w3, "error in"=w2) -> ("task out"=w31:refnum<k21>)  [unwired: 12 in, 1 out]
  n15 = while {
    tunnel: [w129] -> w77
    tunnel: [w320] -> w78
    tunnel: [w128] -> w76
    tunnel: [w429] -> w73
    tunnel: w31 -> [w114]
    tunnel: w30 -> [w112]
    tunnel: w29 -> [w111]
    stop <- w429 stop-if-true
    w169 = "NI_ChannelName" ("name")
    w245 = -1
    # "Scan # counter"
    # "DAQ loop iteration\ncounter (for timing)"
    # "Step counter"
    # "Force feedback"
    # "Raster scan"
    # "Rewire everything"
    # "Invert these because changed\nfrom PSD to QPD"
    # "Trap Y"
    # "Trap X"
    # "Convert to\npN"
    # "Convert to\nnm"
    # "Subtract\noffset"
    # "Normalize by\nsum"
    # "B sum"
    # "BX"
    # "BY"
    # "AX"
    # "AY"
    # "A sum"
    # "Close files when done saving"
    n16 = disable-structure shown="Disabled" {
      frame Disabled {
        n17 = property class="DAQmx Read"() -> ("AvailSampPerChan"=→"AvailSampPerChan 2":u32)  [unwired: 2 in, 2 out]
      }
      frame Enabled {
      }
    }
    n18 = local read "Averaging Number"() -> (w136:i32)
    n19 = local read "Averaging Number"() -> (w139:i32)
    "# Samples/channel" <- w139
    n20 = local read "Sampling Rate"() -> (w428:dbl)
    n21 = call-poly <vilib>:"DAQmx Read.vi"("task/channels in"=w114, "number of samples per channel"=w136, "timeout"=10.0) -> ("task out"=w113:refnum<k21>, "data"=w137:dbl[][], "error out"=w248:errorcluster)  [unwired: 10 in]
    n22 = Unbundle By Name(w248) -> ("status"=w368:bool)
    n23 = Divide(x=w428, y="Cal Averaging") -> (x/y=→"Cal Final Sampling Rate":dbl)
    n24 = Divide(x=w428, y=w139) -> (x/y=→"Final Sampling Rate" →"# Samples/channel/s":dbl)
    n25 = disable-structure shown="Disabled" {
      frame Disabled {
        n26 = local read "Buffer size\n(Samples/channel)"() -> (w431:u32)
        n27 = property class="DAQmx Read"() -> ("AvailSampPerChan"=w432:u32)  [unwired: 2 in, 2 out]
        "AvailSampPerChan" <- w432
        n28 = Divide(x=w432, y=w431) -> (x/y=→"Buffer status":dbl)
      }
      frame Enabled {
      }
    }
    n29 = case shown="True" w368 {
      frame False {
      }
      frame True {
        n30 = call <vilib>:"Beep.vi"() -> ()  [unwired: 12 in]
        "Buffer Overflow" <- TRUE
      }
    }
    n31 = local read "Cal values"() -> (w360:T1)
    n32 = Index Array(array=w137, index (row)=4) -> (element=w237:dbl[])  [unwired: 1 in]
    n33 = Index Array(array=w137, index (row)=0) -> (element=w247:dbl[])  [unwired: 1 in]
    n34 = Index Array(array=w137, index (row)=2) -> (element=w242:dbl[])  [unwired: 1 in]
    n35 = Index Array(array=w137, index (row)=1) -> (element=w246:dbl[])  [unwired: 1 in]
    n36 = Index Array(array=w137, index (row)=3) -> (element=w240:dbl[])  [unwired: 1 in]
    n37 = Index Array(array=w137, index (row)=6) -> (element=w239:dbl[])  [unwired: 1 in]
    n38 = Index Array(array=w137, index (row)=7) -> (element=w238:dbl[])  [unwired: 1 in]
    n39 = Index Array(array=w137, index (row)=5) -> (element=w236:dbl[])  [unwired: 1 in]
    n40 = Unbundle(w360) -> ("AX alpha"=w348:dbl, "BX alpha"=w344:dbl, "AX kappa"=w340:dbl, "BX kappa"=w336:dbl, "AX offset"=w354:dbl, "BX offset"=w352:dbl, "AY alpha"=w351:dbl, "BY alpha"=w346:dbl, "AY kappa"=w342:dbl, "BY kappa"=w338:dbl, "AY offset"=w358:dbl, "BY offset"=w356:dbl)
    n41 = Multiply(x=w246, y=w245) -> (x*y=w241:dbl[])
    n42 = Multiply(x=w247, y=w245) -> (x*y=w243:dbl[])
    n43 = local write "AX alpha"(w348) -> ()
    n44 = local write "BY offset"(w356) -> ()
    n45 = Build Array(w243, w242, w241, w240, w239, w238, w237, w236) -> (w166:dbl[][])
    n46 = local write "BX alpha"(w344) -> ()
    n47 = case shown="True" "Reset data stream" {
      selector: "Reset data stream" -> [_ w567]
      tunnel: w113 -> [w559 w565]
      tunnel: [w559 w563] -> w320
      tunnel: w248 -> [w558 w562]
      tunnel: [w558 w560] -> _
      frame False {
      }
      frame True {
        n48 = Not(x=w567) -> (.not. x?=w566:bool)
        n49 = call <vilib>:"DAQmx Stop Task.vi"("task/channels in"=w565, "error in"=w562) -> ("task out"=w564:refnum<k21>, "error out"=w561:errorcluster)  [unwired: 12 in]
        n50 = local write "Reset data stream"(w566) -> ()
        n51 = local write "Buffer Overflow"(w566) -> ()
        n52 = call <vilib>:"DAQmx Start Task.vi"("task/channels in"=w564, "error in"=w561) -> ("task out"=w563:refnum<k21>, "error out"=w560:errorcluster)  [unwired: 12 in]
      }
    }
    n53 = call-poly <vilib>:"Mean.vi"("X"=w236) -> ("mean"=w372:dbl)  [unwired: 1 out]
    n54 = local write "AY offset"(w358) -> ()
    n55 = call-poly <vilib>:"Mean.vi"("X"=w237) -> ("mean"=w373:dbl)  [unwired: 1 out]
    n56 = call-poly <vilib>:"Mean.vi"("X"=w242) -> ("mean"=w379:dbl)  [unwired: 1 out]
    n57 = call-poly <vilib>:"Mean.vi"("X"=w240) -> ("mean"=w377:dbl)  [unwired: 1 out]
    n58 = call-poly <vilib>:"Mean.vi"("X"=w239) -> ("mean"=w376:dbl)  [unwired: 1 out]
    n59 = call-poly <vilib>:"Mean.vi"("X"=w238) -> ("mean"=w375:dbl)  [unwired: 1 out]
    n60 = local read "Averaging Number"() -> (w135:i32)
    n61 = local write "BY kappa"(w338) -> ()
    n62 = local write "AX kappa"(w340) -> ()
    n63 = call-poly <vilib>:"Mean.vi"("X"=w241) -> ("mean"=w378:dbl)  [unwired: 1 out]
    n64 = local write "AY kappa"(w342) -> ()
    n65 = call-poly <vilib>:"Mean.vi"("X"=w243) -> ("mean"=w380:dbl)  [unwired: 1 out]
    n66 = local read "DAQ rate\n(Samples/s)"() -> (w144:dbl)
    n67 = Build Array(w373, w372) -> (w371:dbl[])
    n68 = local write "BX kappa"(w336) -> ()
    n69 = local write "BY alpha"(w346) -> ()
    n70 = local write "AX offset"(w354) -> ()
    n71 = local write "BX offset"(w352) -> ()
    n72 = local write "AY alpha"(w351) -> ()
    n73 = Build Array(w380, w379, w378, w377, w376, w375) -> (w369:dbl[])
    n74 = Divide(x=w135, y=w144) -> (x/y=w141:dbl)
    "Data update period (s/set)" <- w141
    n75 = Reciprocal(x=w144) -> (1/x=w145:dbl)
    "Data period (s)" <- w145
    n76 = Divide(x=w380, y=w376) -> (x/y=w410:dbl)
    n77 = Divide(x=w379, y=w376) -> (x/y=w411:dbl)
    n78 = Divide(x=w378, y=w375) -> (x/y=w418:dbl)
    n79 = Divide(x=w377, y=w375) -> (x/y=w419:dbl)
    n80 = Subtract(x=w410, y="AY offset") -> (x-y=w392:dbl)
    n81 = Subtract(x=w411, y="AX offset") -> (x-y=w393:dbl)
    n82 = Subtract(x=w418, y="BY offset") -> (x-y=w391:dbl)
    n83 = Subtract(x=w419, y="BX offset") -> (x-y=w394:dbl)
    n84 = Subtract(x=w418, y=w410) -> (x-y=w408:dbl)
    n85 = Subtract(x=w419, y=w411) -> (x-y=w409:dbl)
    n86 = feedback #1(0.0) -> (w319:dbl)
    n87 = Multiply(x="Downsamp\nfact", y=w145) -> (x*y=w146:dbl)
    n88 = Multiply(x=w392, y="AY alpha") -> (x*y=w328:dbl)
    n89 = Multiply(x=w393, y="AX alpha") -> (x*y=w326:dbl)
    n90 = Multiply(x=w394, y="BX alpha") -> (x*y=w327:dbl)
    n91 = Multiply(x=w391, y="BY alpha") -> (x*y=w329:dbl)
    n92 = Add(x=w141, y=w319) -> (x+y=w317:dbl)
    n93 = feedback-in #1(w317) -> ()
    n94 = Square(x=w328) -> (x^2=w402:dbl)
    n95 = Square(x=w326) -> (x^2=w403:dbl)
    n96 = Square(x=w329) -> (x^2=w404:dbl)
    n97 = Square(x=w327) -> (x^2=w405:dbl)
    n98 = Bundle(w408, w409) -> (w138:cluster{dbl, dbl})  [unwired: 1 in]
    n99 = case shown="True" "Set Initial Delta" {
      tunnel: w138 -> [_ _]
      frame False {
      }
      frame True {
        n100 = local read "Trap delta (nm)"() -> (w556:dbl)
        n101 = local write "Set Initial Delta"(FALSE ("Set reading to\nsetpoint")) -> ()
        n102 = local write "Initial Delta (nm)"(w556) -> ()
      }
    }
    n103 = Reciprocal(x=w146) -> (1/x=→"Chart Freq (Hz)":dbl)
    n104 = To Time Stamp(1:w317) -> (0:w316:timestamp)
    n105 = Add(x=w402, y=w403) -> (x+y=w406:dbl)
    n106 = Add(x=w404, y=w405) -> (x+y=w417:dbl)
    n107 = Multiply(x=w326, y="AX kappa") -> (x*y=w322:dbl)
    n108 = Bundle("A y", "A x", "B y", "B x", "A sum", "B sum", "Trap x", "Trap y") -> (w307:T10)  [unwired: 1 in]
    n109 = Multiply(x=w327, y="BX kappa") -> (x*y=w323:dbl)
    n110 = Square Root(x=w406) -> (sqrt(x)=w422:dbl)
    n111 = Square Root(x=w417) -> (sqrt(x)=w421:dbl)
    n112 = Multiply(x=w328, y="AY kappa") -> (x*y=w324:dbl)
    n113 = Multiply(x=w329, y="BY kappa") -> (x*y=w325:dbl)
    n114 = Subtract(x=w372, y="Fixed Y") -> (x-y=w407:dbl)
    n115 = Subtract(x=w373, y="Fixed X") -> (x-y=w412:dbl)
    n116 = Cluster To Array(cluster=w307) -> (array=w306:string[])
    n117 = for {
      tunnel: w166 -> [w548] mode=indexing
      tunnel: w146 -> [w547]
      tunnel: "Downsamp\nfact" -> [w553]
      tunnel: [w551] -> w222 mode=indexing
      tunnel: w316 -> [w555]
      tunnel: w306 -> [w550] mode=indexing
      tunnel: "NI_ChannelName" ("name") -> [w549]
      n118 = call "Downsample 1D array.vi"("Ave N"=w553, "Arrray In"=w548) -> ("Array Out"=w554:dbl[])  [unwired: 9 in]
      n119 = Bundle By Name("Y"=w554, "dt"=w547, "t0"=w555) -> (w552:waveform(dbl))  [unwired: 1 in]
      n120 = Set Waveform Attribute(5:w550, 6:w549, 7:w552) -> (3:w551:waveform(dbl))  [unwired: 1 in, 2 out]
    }
    "All signals" <- w222
    n121 = Square(x=w324) -> (x^2=w395:dbl)
    n122 = Square(x=w322) -> (x^2=w396:dbl)
    n123 = Square(x=w325) -> (x^2=w397:dbl)
    n124 = Square(x=w323) -> (x^2=w398:dbl)
    n125 = Add(x=w395, y=w396) -> (x+y=w399:dbl)
    n126 = Add(x=w397, y=w398) -> (x+y=w400:dbl)
    n127 = Multiply(x=w407, y="Conv Y (nm/V)") -> (x*y=w331:dbl)
    n128 = Multiply(x=w412, y="Conv X (nm/V)") -> (x*y=w332:dbl)
    n129 = Square Root(x=w399) -> (sqrt(x)=w330:dbl)
    n130 = Square Root(x=w400) -> (sqrt(x)=w423:dbl)
    n131 = Add(x=w330, y=w423) -> (x+y=w401:dbl)
    n132 = Build Array(w410, w411, w418, w419, w376, w375, w330, w423, w422, w421, w332, w331) -> ()  [unwired: 1 out]
    n133 = Divide(x=w401, y=2.0) -> (x/y=w367:dbl)
    n134 = Index Array(array=w222, index=6) -> (element=w171:waveform(dbl))
    n135 = Index Array(array=w222, index=7) -> (element=w173:waveform(dbl))
    n136 = feedback #2(0.0) -> (w109:dbl)
    n137 = case shown="True" "Force Feedback" {
      tunnel: [0.0 w846] -> w110
      tunnel: w109 -> [_ w844]
      frame False {
        # "Force feedback"
      }
      frame True {
        w852 = 0.0  # Kdiff
        n138 = Unbundle("PID gains") -> ("Kprop"=w854:dbl, "Kint"=w853:dbl)
        n139 = local read "Mean force (pN)"() -> (w847:dbl)
        n140 = Bundle("Kprop"=w854, "Kint"=w853, "Kdiff"=w852) -> (w851:cluster{"Kprop":dbl, "Kint":dbl, "Kdiff":dbl})  [unwired: 1 in]
        n141 = local read "Pulling direction"() -> (w841:bool)
        n142 = local read "AY kappa"() -> (w850:dbl)
        n143 = local read "AX kappa"() -> (w849:dbl)
        n144 = Select(t=w850, s=w841, f=w849) -> (s? t:f=w843:dbl)
        n145 = Subtract(x="Desired Force (pN)", y=w847) -> (x-y=w845:dbl)
        n146 = call-poly <vilib>:"PID.vi"("reinitialize? (F)"="reinitialize error", "PID gains"=w851, "process variable"=w847, "setpoint"="Desired Force (pN)") -> ("output"=w842:dbl)  [unwired: 6 in, 1 out]
        n147 = Add(x=w845, y=w844) -> (x+y=w846:dbl)
        "Sum error" <- w846
        n148 = Multiply(x=w843, y=w842) -> (x*y=w840:dbl)
        n149 = Add(x="Initial Delta (nm)", y=w840) -> (x+y=w839:dbl)
        n150 = property on="Trap delta (nm)" class="DigNum (strict)"("Val(Sgnl)"=w839) -> ()  [unwired: 2 in, 2 out]
      }
    }
    n151 = feedback-in #2(w110) -> ()
    n152 = local read "Fixed X"() -> (w226:dbl)
    n153 = local read "Fixed Y"() -> (w228:dbl)
    n154 = Unbundle By Name(w171) -> ("Y"=w230:dbl[])
    n155 = Unbundle By Name(w173) -> ("Y"=w229:dbl[])
    n156 = Index Array(array=w222, index=0) -> (element=w179:waveform(dbl))
    n157 = Index Array(array=w222, index=1) -> (element=w303:waveform(dbl))
    n158 = Index Array(array=w222, index=4) -> (element=w297:waveform(dbl))
    n159 = Subtract(x=w230, y=w226) -> (x-y=w227:dbl[])
    n160 = Subtract(x=w229, y=w228) -> (x-y=w224:dbl[])
    n161 = Unbundle By Name(w179) -> ("Y"=w295:dbl[])
    n162 = Unbundle By Name(w303) -> ("Y"=w294:dbl[])
    n163 = Unbundle By Name(w297) -> ("Y"=w293:dbl[])
    n164 = Index Array(array=w222, index=5) -> (element=w296:waveform(dbl))
    n165 = local read "Conv X (nm/V)"() -> (w225:dbl)
    n166 = local read "Conv Y (nm/V)"() -> (w223:dbl)
    n167 = Index Array(array=w222, index=2) -> (element=w176:waveform(dbl))
    n168 = Index Array(array=w222, index=3) -> (element=w300:waveform(dbl))
    n169 = Set Waveform Attribute(5:"T2 X", 6:w169, 7:w171) -> (3:w170:waveform(dbl))  [unwired: 1 in, 2 out]
    n170 = Set Waveform Attribute(5:"T2 Y", 6:w169, 7:w173) -> (3:w172:waveform(dbl))  [unwired: 1 in, 2 out]
    n171 = Unbundle By Name(w296) -> ("Y"=w290:dbl[])
    n172 = Unbundle By Name(w176) -> ("Y"=w292:dbl[])
    n173 = Unbundle By Name(w300) -> ("Y"=w291:dbl[])
    n174 = local read "Saving"() -> (w333:bool)
    n175 = local read "Tether"() -> (w334:bool)
    n176 = Divide(x=w295, y=w293) -> (x/y=w194:dbl[])
    n177 = Divide(x=w294, y=w293) -> (x/y=w192:dbl[])
    n178 = local read "AY offset"() -> (w281:dbl)
    n179 = local read "AX offset"() -> (w279:dbl)
    n180 = Multiply(x=w227, y=w225) -> (x*y=w163:dbl[])
    n181 = Multiply(x=w224, y=w223) -> (x*y=w165:dbl[])
    n182 = Less?(x=w367, y="Tether break\nforce (pN)") -> (x < y?=w365:bool)
    n183 = Divide(x=w291, y=w290) -> (x/y=w193:dbl[])
    n184 = Subtract(x=w192, y=w279) -> (x-y=w282:dbl[])
    n185 = local read "BY offset"() -> (w286:dbl)
    n186 = local read "BX offset"() -> (w289:dbl)
    n187 = Subtract(x=w194, y=w281) -> (x-y=w283:dbl[])
    n188 = Divide(x=w292, y=w290) -> (x/y=w195:dbl[])
    n189 = local read "AY alpha"() -> (w280:dbl)
    n190 = local read "AX alpha"() -> (w278:dbl)
    n191 = Compound Arithmetic op=AND(w333, w334, w365) -> (w364:bool)
    n192 = call-poly <vilib>:"Mean.vi"("X"=w165) -> ("mean"=w205:dbl)  [unwired: 1 out]
    "Mean Trp Pos Y 2 (nm)" <- w205
    n193 = Subtract(x=w195, y=w194) -> (x-y=w191:dbl[])
    n194 = Subtract(x=w193, y=w192) -> (x-y=w190:dbl[])
    n195 = Subtract(x=w163, y="Offset X (nm)") -> (x-y=w162:dbl[])
    n196 = Subtract(x=w165, y="Offset Y (nm)") -> (x-y=w164:dbl[])
    n197 = Subtract(x=w195, y=w286) -> (x-y=w288:dbl[])
    n198 = Subtract(x=w193, y=w289) -> (x-y=w287:dbl[])
    n199 = Subtract(x=w205, y=w165) -> (x-y=w204:dbl[])
    n200 = call-poly <vilib>:"Mean.vi"("X"=w163) -> ("mean"=w209:dbl)  [unwired: 1 out]
    "Mean Trap Pos X 2 (nm)" <- w209
    n201 = Build Array(w191, w190) -> (w188:dbl[][])
    n202 = Index Array(array=w188, index (row)=0) -> (element=w186:dbl[])  [unwired: 1 in]
    n203 = Index Array(array=w188, index (row)=1) -> (element=w185:dbl[])  [unwired: 1 in]
    n204 = call-poly <vilib>:"Mean.vi"("X"=w186) -> ("mean"=w184:dbl)  [unwired: 1 out]
    n205 = call-poly <vilib>:"Mean.vi"("X"=w185) -> ("mean"=w183:dbl)  [unwired: 1 out]
    n206 = Bundle("mean"=w184, "mean"=w183) -> ()  [unwired: 1 in, 1 out]
    n207 = local read "BY alpha"() -> (w285:dbl)
    n208 = local read "BX alpha"() -> (w284:dbl)
    n209 = Multiply(x=w283, y=w280) -> (x*y=w271:dbl[])
    n210 = Multiply(x=w282, y=w278) -> (x*y=w270:dbl[])
    n211 = Square(x=w204) -> (x^2=w203:dbl[])
    n212 = Subtract(x=w209, y=w163) -> (x-y=w208:dbl[])
    n213 = Bundle By Name(cluster=w172, "Y"=w164) -> (w220:waveform(dbl))
    n214 = Bundle By Name(cluster=w170, "Y"=w162) -> (w221:waveform(dbl))
    n215 = case shown="True" w364 {
      selector: w364 -> [_ w571]
      frame False {
      }
      frame True {
        n216 = call <vilib>:"Beep.vi"() -> ()  [unwired: 12 in]
        n217 = Not(x=w571) -> (.not. x?=w569:bool)
        n218 = local write "Tether"(w569) -> ()
        n219 = local write "Force Feedback"(w569) -> ()
        n220 = property on="Stop saving" class="Bool (strict)"("Val(Sgnl)"="TA Cancel Save?") -> ()  [unwired: 2 in, 2 out]
        n221 = property on="Fish" class="Bool (strict)"("Val(Sgnl)"="Fish After TA?") -> ()  [unwired: 2 in, 2 out]
      }
    }
    n222 = Square(x=w208) -> (x^2=w207:dbl[])
    n223 = call-poly <vilib>:"Mean.vi"("X"=w203) -> ("mean"=w202:dbl)  [unwired: 1 out]
    n224 = Square(x=w271) -> (x^2=w277:dbl[])
    n225 = Multiply(x=w288, y=w285) -> (x*y=w269:dbl[])
    n226 = Square(x=w270) -> (x^2=w276:dbl[])
    n227 = Multiply(x=w287, y=w284) -> (x*y=w268:dbl[])
    n228 = call-poly <vilib>:"Mean.vi"("X"=w207) -> ("mean"=w206:dbl)  [unwired: 1 out]
    n229 = Build Array(w221, w220) -> (w130:waveform(dbl)[])
    "Trap sep" <- w130
    n230 = Square Root(x=w202) -> (sqrt(x)=w201:dbl)
    n231 = Square(x=w269) -> (x^2=w275:dbl[])
    n232 = Square(x=w268) -> (x^2=w274:dbl[])
    n233 = Add(x=w277, y=w276) -> (x+y=w273:dbl[])
    n234 = Square Root(x=w206) -> (sqrt(x)=w199:dbl)
    n235 = Multiply(x=w201, y=10) -> (x*y=→"T2 Y RMS (A)":dbl)
    n236 = Square Root(x=w273) -> (sqrt(x)=w158:dbl[])
    n237 = Add(x=w275, y=w274) -> (x+y=w272:dbl[])
    n238 = Set Waveform Attribute(5:"T2", 6:"NI_ChannelName" ("name"), 7:w179) -> (3:w178:waveform(dbl))  [unwired: 1 in, 2 out]
    n239 = Set Waveform Attribute(5:"T1", 6:"NI_ChannelName" ("name"), 7:w176) -> (3:w175:waveform(dbl))  [unwired: 1 in, 2 out]
    n240 = Square Root(x=w272) -> (sqrt(x)=w157:dbl[])
    n241 = Multiply(x=w199, y=10) -> (x*y=→"T2 X RMS (A)":dbl)
    n242 = Bundle By Name(cluster=w178, "Y"=w158) -> (w182:waveform(dbl))
    n243 = Bundle By Name(cluster=w175, "Y"=w157) -> (w250:waveform(dbl))
    n244 = Add(x=w158, y=w157) -> (x+y=w156:dbl[])
    n245 = case shown="True" "Remove offsets" {
      selector: "Remove offsets" -> [_ w545]
      frame False {
      }
      frame True {
        n246 = local read "Mean Trp Pos Y 2 (nm)"() -> (w543:dbl)
        n247 = Not(x=w545) -> (.not. x?=w546:bool)
        n248 = local read "Mean Trap Pos X 2 (nm)"() -> (w544:dbl)
        n249 = local write "Remove offsets"(w546) -> ()
        n250 = local write "Offset Y (nm)"(w543) -> ()
        n251 = local write "Offset X (nm)"(w544) -> ()
      }
    }
    n252 = Build Array(w182, w250) -> (→"Bead sep":waveform(dbl)[])
    n253 = local read "AY kappa"() -> (w267:dbl)
    n254 = local read "AX kappa"() -> (w266:dbl)
    n255 = Divide(x=w156, y=2) -> (x/y=w154:dbl[])
    n256 = local read "Raster scanning..."() -> (w127:bool)
    n257 = local read "BX kappa"() -> (w264:dbl)
    n258 = local read "BY kappa"() -> (w265:dbl)
    n259 = call-poly <vilib>:"Mean.vi"("X"=w154) -> ("mean"=w153:dbl)  [unwired: 1 out]
    "Mean Bead Sep\n(nm)" <- w153
    n260 = local read "Calibrating"() -> (w424:bool)
    n261 = Multiply(x=w271, y=w267) -> (x*y=w260:dbl[])
    n262 = Multiply(x=w270, y=w266) -> (x*y=w261:dbl[])
    n263 = Square(x=w260) -> (x^2=w259:dbl[])
    n264 = Square(x=w261) -> (x^2=w258:dbl[])
    n265 = Subtract(x=w154, y=w153) -> (x-y=w152:dbl[])
    n266 = Multiply(x=w269, y=w265) -> (x*y=w262:dbl[])
    n267 = Multiply(x=w268, y=w264) -> (x*y=w263:dbl[])
    n268 = Add(x=w259, y=w258) -> (x+y=w255:dbl[])
    n269 = Square(x=w152) -> (x^2=w151:dbl[])
    n270 = Or(x=w127, y="Raster scan") -> (x .or. y?=w126:bool)
    n271 = Square Root(x=w255) -> (sqrt(x)=w219:dbl[])
    n272 = Square(x=w262) -> (x^2=w257:dbl[])
    n273 = Square(x=w263) -> (x^2=w256:dbl[])
    n274 = call-poly <vilib>:"Mean.vi"("X"=w151) -> ("mean"=w150:dbl)  [unwired: 1 out]
    n275 = Add(x=w257, y=w256) -> (x+y=w254:dbl[])
    n276 = Bundle By Name(cluster=w178, "Y"=w219) -> (w253:waveform(dbl))
    n277 = local read "Saving"() -> (w363:bool)
    n278 = Or(x=w424, y=w363) -> ()  [unwired: 1 out]
    n279 = Square Root(x=w150) -> (sqrt(x)=w149:dbl)
    n280 = Square Root(x=w254) -> (sqrt(x)=w218:dbl[])
    n281 = Multiply(x=10, y=w149) -> (x*y=→"Bead Sep Noise\n(A)":dbl)
    n282 = Bundle By Name(cluster=w175, "Y"=w218) -> (w252:waveform(dbl))
    n283 = Add(x=w219, y=w218) -> (x+y=w217:dbl[])
    n284 = Build Array(w253, w252) -> (→"Force (pN)":waveform(dbl)[])
    n285 = Divide(x=w217, y=2) -> (x/y=w214:dbl[])
    n286 = call-poly <vilib>:"Mean.vi"("X"=w214) -> ("mean"=w215:dbl)  [unwired: 1 out]
    "Mean force (pN)" <- w215
    n287 = Subtract(x=w215, y=w214) -> (x-y=w213:dbl[])
    n288 = Square(x=w213) -> (x^2=w212:dbl[])
    n289 = call-poly <vilib>:"Mean.vi"("X"=w212) -> ("mean"=w211:dbl)  [unwired: 1 out]
    n290 = Square Root(x=w211) -> (sqrt(x)=→"Force noise (pN)":dbl)
    n291 = flat-sequence {
      tunnel: w424 -> [w611]
      tunnel: w363 -> [_]
      tunnel: w424 -> [_]
      tunnel: w363 -> [_]
      tunnel: w166 -> [w598]
      tunnel: [w598] -> w382
      tunnel: w248 -> [w597]
      tunnel: [w597] -> w381
      tunnel: w369 -> [w596]
      tunnel: [w596] -> w374
      tunnel: w371 -> [w595]
      tunnel: [w595] -> w370
      tunnel: [w592] -> w362
      tunnel: [w589] -> w361
      tunnel: [w586] -> w235
      tunnel: [w585] -> w234
      tunnel: [w582] -> w233
      tunnel: w132 -> [w579]
      tunnel: ["Save Data"] -> w131
      tunnel: w382 -> [w759]
      tunnel: w381 -> [w758]
      tunnel: w374 -> [_]
      tunnel: w370 -> [_]
      tunnel: w362 -> [w757]
      tunnel: w361 -> [w756]
      tunnel: w235 -> [w755]
      tunnel: w234 -> [w754]
      tunnel: w233 -> [w753]
      tunnel: w131 -> [w751]
      tunnel: w130 -> [w750]
      frame #0 {
        w577 = 0.0
        # "1: old trap\n0: fleezers"
        # "Create files if saving data"
        n292 = local read "Save N sets"() -> (w581:bool)
        n293 = local read "Sampling Rate"() -> (w609:dbl)
        n294 = Or(x=w581, y="Save Data") -> (x .or. y?=w580:bool)
        n295 = Build Array(w580, "Save cal", w579) -> (w600:bool[])
        n296 = Compound Arithmetic op=OR("Save Data", "Save cal", w579) -> (w602:bool)
        n297 = Boolean Array To Number(Boolean array=w600) -> (number=w599:u32)
        n298 = local read "Trap position (V)"() -> (w606:cluster{"X":dbl, "Y":dbl})
        n299 = local read "Fixed X"() -> (w576:dbl)
        n300 = local read "Fixed Y"() -> (w575:dbl)
        n301 = Unbundle(w606) -> ("X"=w574:dbl, "Y"=w573:dbl)
        n302 = Build Array(w574, w573, w576, w575, w577, w577) -> (w605:dbl[])
        n303 = feedback #3(refnum<k0> refnum) -> (w590:refnum<file>)
        n304 = feedback #4() -> (w587:dbl)  [unwired: 1 in]
        n305 = feedback #5(FALSE) -> (w583:bool)
        n306 = feedback #6(0) -> (w603:i32)
        n307 = feedback #7(refnum<k0> refnum) -> (w593:refnum<file>)
        n308 = case shown="True" w602 {
          tunnel: w611 -> [_ _]
          tunnel: 9 -> [_ w654]
          tunnel: w609 -> [_ w653]
          tunnel: 6 -> [_ w652]
          tunnel: 5 -> [_ w651]
          tunnel: w605 -> [_ w650]
          tunnel: [w616 1] -> w586
          tunnel: w603 -> [w617 _]
          tunnel: w599 -> [_ w625]
          tunnel: [w615 w623] -> w592
          tunnel: w593 -> [w615 _]
          tunnel: [w614 w622] -> w589
          tunnel: w590 -> [w614 _]
          tunnel: 1.0 -> [_ w621]
          tunnel: [w613 w620] -> w585
          tunnel: w587 -> [w613 _]
          tunnel: [w612 w619] -> w582
          tunnel: w583 -> [w612 _]
          frame False {
            n309 = Increment(x=w617) -> (x+1=w616:i32)
          }
          frame True {
            w626 = FALSE ("Save Data")
            w632 = FALSE
            w633 = T9."big-endian, network order" ("byte order (0:big-endian, network order)")
            n310 = local write "Save cal"(w626) -> ()
            n311 = local write "Save Data"(w626) -> ()
            n312 = case shown="4" w625 {
              tunnel: w654 -> [w701 w719 w749]
              tunnel: w653 -> [w679 w718 w724]
              tunnel: w652 -> [w700 w716 w745]
              tunnel: w651 -> [w699 w715 w744]
              tunnel: w650 -> [w697 w712 w741]
              tunnel: [w696 w711 w730] -> w647
              tunnel: [w698 w708 w729] -> w619
              tunnel: ["Averaging Number" 200 w727] -> _
              tunnel: w621 -> [w684 w703 w726]
              tunnel: [w680 "Cal sets to save" w720] -> w620
              frame 1, Default {
                w698 = TRUE
                w685 = 0.0
                # "Time trace"
                n313 = local read "Averaging Number"() -> (w695:i32)
                n314 = Boolean To (0,1)(Boolean=w698) -> (0, 1=w690:i16)
                n315 = Increment(x=w690) -> (x+1=w689:i16)
                n316 = Divide(x=w679, y=w695) -> (x/y=w694:dbl)
                n317 = To Double Precision Float(number=w689) -> (double precision float=w688:dbl)
                n318 = Reciprocal(x=w694) -> (1/x=w693:dbl)
                n319 = Reciprocal(x=w679) -> (1/x=w678:dbl)
                n320 = Build Array(w701, w678, w693, w700, w699, 0 ("f")) -> (w692:dbl[])
                n321 = Build Array(w688, w684, w685, w685, w685) -> (w691:dbl[])
                n322 = Build Array (concatenate)(w692, w697, w691) -> (w696:dbl[])
                n323 = Select(t="N sets", s="Save N sets", f=2147483647) -> (s? t:f=w680:i32)
              }
              frame 2 {
                w708 = FALSE
                w706 = 0.0
                # "Calibration file"
                n324 = Reciprocal(x=w718) -> (1/x=w717:dbl)
                n325 = Boolean To (0,1)(Boolean=w708) -> (0, 1=w710:i16)
                n326 = To Double Precision Float(number=w710) -> (double precision float=w709:dbl)
                n327 = Build Array(w719, w717, w717, w716, w715, 1) -> (w713:dbl[])
                n328 = Build Array(w709, w703, w706, w706, w706) -> (w707:dbl[])
                n329 = Build Array (concatenate)(w713, w712, w707) -> (w711:dbl[])
                "Calibrating" <- TRUE ("Calibrating")
              }
              frame 4 {
                w737 = 0.0
                w729 = TRUE
                # "Not using ncycles"
                # "FX curve"
                n330 = local read "Averaging Number"() -> (w748:i32)
                n331 = Boolean To (0,1)(Boolean=w729) -> (0, 1=w740:i16)
                n332 = Increment(x=w740) -> (x+1=w739:i16)
                n333 = local write "Raster scan"(FALSE ("Raster scan")) -> ()
                n334 = To Double Precision Float(number=w739) -> (double precision float=w738:dbl)
                n335 = Divide(x=w724, y=w748) -> (x/y=w747:dbl)
                n336 = Reciprocal(x=w747) -> (1/x=w746:dbl)
                n337 = Build Array(w738, w726, w737, w737, w737) -> (w736:dbl[])
                n338 = Reciprocal(x=w724) -> (1/x=w723:dbl)
                n339 = Build Array(w749, w723, w746, w745, w744, 2) -> (w742:dbl[])
                n340 = local read "Pulling direction"() -> (w734:bool)
                n341 = local read "Scan range (V)"() -> (w721:dbl)
                n342 = local read "N sets to be saved"() -> (w720:dbl)
                n343 = local read "Scan steps (mirror)"() -> (w722:u64)
                n344 = local read "# scans"() -> (w732:i32)
                n345 = Not(x=w734) -> (.not. x?=w733:bool)
                n346 = local read "Averaging Number"() -> (w727:i32)
                n347 = Boolean To (0,1)(Boolean=w733) -> (0, 1=w735:i16)
                n348 = Build Array(w735, w721, w722, 0, w732) -> (w731:dbl[])
                n349 = Build Array (concatenate)(w742, w741, w736, w731) -> (w730:dbl[])
              }
            }
            n350 = call "CreateSaveFile.vi"("Index In"="Save file index", "Ext"=".dat", "Insert"="", "Directory"="Path") -> ("Index Out"=w618:i32, "Path Out"=w631:path)  [unwired: 6 in]
            "Current file name" <- w631
            n351 = Open/Create/Replace File(file path (use dialog)=w631, operation (0:open)=T8."create", access (0:read/write)=enum16{"read/write", "read-only", "write-only"}."write-only") -> (refnum out=w640:refnum<file>, error out=w641:errorcluster)  [unwired: 3 in, 1 out]
            n352 = local write "Save file index"(w618) -> ()
            n353 = Array Size(array=w647) -> (size(s)=w649:i32)
            n354 = case shown="True" w619 {
              tunnel: w631 -> [_ w677]
              tunnel: [refnum<k0> refnum w656] -> w622
              frame False {
              }
              frame True {
                w663 = 0.0
                n355 = Path To String(path=w677) -> (string=w673:string)
                n356 = Build Array(w663, w663, w663, w663, w663, w663, w663, w663) -> (w660:dbl[])
                n357 = String Length(string=w673) -> (length=w676:i32)
                n358 = Array Size(array=w660) -> (size(s)=w662:i32)
                n359 = Subtract(x=w676, y=4) -> (x-y=w674:i32)
                n360 = To Double Precision Float(number=w662) -> (double precision float=w661:dbl)
                n361 = String Subset(string=w673, length (rest)=w674) -> (substring=w672:string)  [unwired: 1 in]
                n362 = Build Array (concatenate)(w661, w660) -> (w659:dbl[])
                n363 = Concatenate Strings(w672, "_pos.dat" ("string")) -> (w670:string)
                n364 = String To Path(string=w670) -> (path=w669:path)
                n365 = Open/Create/Replace File(file path (use dialog)=w669, operation (0:open)=T8."create", access (0:read/write)=enum16{"read/write", "read-only", "write-only"}."write-only") -> (refnum out=w665:refnum<file>, error out=w666:errorcluster)  [unwired: 3 in, 1 out]
                n366 = Deny Access(4:w666, 7:w665) -> (3:w664:refnum<file>)  [unwired: 1 in, 1 out]
                n367 = Write to Binary File(file (use dialog)=w664, data=w659, 5:FALSE ("prepend array or string size? (T)"), 9:T9."big-endian, network order" ("byte order (0:big-endian, network order)")) -> (refnum out=w656:refnum<file>)  [unwired: 2 in, 2 out]
              }
            }
            n368 = Deny Access(4:w641, 7:w640) -> (0:w630:errorcluster, 3:w639:refnum<file>)  [unwired: 1 in]
            n369 = String Length(string="Comment") -> (length=w646:i32)
            n370 = To Double Precision Float(number=w649) -> (double precision float=w648:dbl)
            n371 = To Double Precision Float(number=w646) -> (double precision float=w645:dbl)
            n372 = Build Array (concatenate)(w648, w647, w645) -> (w636:dbl[])
            n373 = Write to Binary File(file (use dialog)=w639, data=w636, error in=w630, 5:w632, 9:w633) -> (refnum out=w635:refnum<file>, error out=w629:errorcluster)  [unwired: 1 in, 1 out]
            n374 = Write to Binary File(file (use dialog)=w635, data="Comment", error in=w629, 5:w632, 9:w633) -> (refnum out=w623:refnum<file>)  [unwired: 1 in, 2 out]
            "Saving" <- TRUE
          }
        }
        n375 = feedback-in #3(w589) -> ()
        n376 = feedback-in #4(w585) -> ()
        n377 = feedback-in #5(w582) -> ()
        n378 = feedback-in #6(w586) -> ()
        n379 = feedback-in #7(w592) -> ()
      }
      frame #1 {
        n380 = local read "Saving"() -> (w752:bool)
        n381 = case shown="True" w752 {
          tunnel: w759 -> [_ w778]
          tunnel: w758 -> [_ w777]
          tunnel: w757 -> [_ w776]
          tunnel: w756 -> [_ w775]
          tunnel: w755 -> [_ w765]
          tunnel: w754 -> [_ w766]
          tunnel: w753 -> [_ w769]
          tunnel: w751 -> [_ w761]
          tunnel: w750 -> [_ w760]
          frame False {
            (unwired) FALSE ("Calibrating")
          }
          frame True {
            n382 = local read "Stop"() -> (w773:bool)
            n383 = Less Or Equal?(x=w765, y=w766) -> (x <= y?=w774:bool)
            n384 = Divide(x=w765, y=w766) -> (x/y=w764:dbl)
            n385 = Or(x=w773, y="Stop saving") -> (x .or. y?=w772:bool)
            n386 = Not(x=w772) -> (.not. x?=w771:bool)
            n387 = Multiply(x=100.0, y=w764) -> (x*y=w763:dbl)
            n388 = And(x=w774, y=w771) -> (x .and. y?=w770:bool)
            n389 = case shown="True" w770 {
              tunnel: w776 -> [w783 w792]
              tunnel: w777 -> [_ w791]
              tunnel: w778 -> [_ w790]
              tunnel: w775 -> [w782 w789]
              tunnel: w769 -> [w780 _]
              tunnel: [0.0 ("Progress") w788] -> w768
              tunnel: w763 -> [_ w788]
              tunnel: w761 -> [_ w785]
              tunnel: w760 -> [_ w786]
              frame False {
                w781 = FALSE
                n390 = Close File(refnum=w783) -> ()  [unwired: 1 in, 2 out]
                n391 = case shown="True" w780 {
                  tunnel: w782 -> [_ w784]
                  frame False {
                  }
                  frame True {
                    n392 = Close File(refnum=w784) -> ()  [unwired: 1 in, 2 out]
                  }
                }
                n393 = call <vilib>:"Beep.vi"() -> ()  [unwired: 12 in]
                n394 = local write "Saving"(w781) -> ()
                n395 = local write "Stop saving"(w781) -> ()
                n396 = local write "Calibrating"(w781) -> ()
              }
              frame True {
                n397 = local read "Calibrating"() -> (w787:bool)
                n398 = case shown="True" w787 {
                  tunnel: w792 -> [w819 w835]
                  tunnel: w791 -> [_ w834]
                  tunnel: w790 -> [w806 w828]
                  tunnel: w789 -> [w805 _]
                  tunnel: w786 -> [w797 _]
                  tunnel: w785 -> [_ _]
                  frame False {
                    n399 = local read "Averaging Number"() -> (w813:i32)
                    n400 = Array Subset(array=w806, index (row)=0 ("index"), length (row)=6 ("length")) -> (w802:dbl[][])  [unwired: 2 in]
                    n401 = Array Subset(array=w806, index (row)=6 ("index"), length (row)=2 ("length")) -> (w801:dbl[][])  [unwired: 2 in]
                    n402 = Array Size(array=w801) -> (size(s)=w812:i32[])
                    n403 = Array Size(array=w802) -> (size(s)=w809:i32[])
                    n404 = Index Array(array=w797, index=0) -> (element=w794:waveform(dbl))
                    n405 = Index Array(array=w797, index=1) -> (element=w793:waveform(dbl))
                    n406 = for {
                      tunnel: w802 -> [w823] mode=indexing
                      tunnel: w813 -> [w825]
                      tunnel: [w824] -> w800 mode=indexing
                      n407 = call "Downsample 1D array.vi"("Ave N"=w825, "Arrray In"=w823) -> ("Array Out"=w824:dbl[])  [unwired: 9 in]
                    }
                    n408 = Unbundle By Name(w794) -> ()  [unwired: 1 out]
                    n409 = Unbundle By Name(w793) -> ()  [unwired: 1 out]
                    n410 = Multiply Array Elements(1:w809) -> (0:w808:i32)
                    n411 = for {
                      tunnel: w801 -> [w822] mode=indexing
                      tunnel: w813 -> [w821]
                      tunnel: [w820] -> w804 mode=indexing
                      n412 = call "Downsample 1D array.vi"("Ave N"=w821, "Arrray In"=w822) -> ("Array Out"=w820:dbl[])  [unwired: 9 in]
                    }
                    n413 = Multiply Array Elements(1:w812) -> (0:w811:i32)
                    n414 = Divide(x=w808, y=w813) -> (x/y=w814:dbl)
                    n415 = Divide(x=w811, y=w813) -> (x/y=w810:dbl)
                    n416 = Transpose 2D Array(2D array=w800) -> (transposed array=w799:dbl[][])
                    n417 = Transpose 2D Array(2D array=w804) -> (transposed array=w798:dbl[][])
                    n418 = Reshape Array(w799, w814) -> (w803:dbl[])
                    n419 = Reshape Array(w798, w810) -> (w807:dbl[])
                    n420 = call <vilib>:"Write File+ [SGL].vi"("1D array"=w807, "refnum"=w805) -> ()  [unwired: 7 in, 3 out]
                    n421 = call <vilib>:"Write File+ [SGL].vi"("1D array"=w803, "refnum"=w819) -> ()  [unwired: 7 in, 3 out]
                  }
                  frame True {
                    n422 = Array Subset(array=w828, index (row)=0 ("index"), length (row)=6 ("length")) -> (w826:dbl[][])  [unwired: 2 in]
                    n423 = Transpose 2D Array(2D array=w826) -> (transposed array=w832:dbl[][])
                    n424 = Array Size(array=w826) -> (size(s)=w827:i32[])
                    n425 = Multiply Array Elements(1:w827) -> (0:w833:i32)
                    n426 = Reshape Array(w832, w833) -> (w831:dbl[])
                    n427 = call <vilib>:"Write File+ [SGL].vi"("1D array"=w831, "error in (no error)"=w834, "refnum"=w835) -> ()  [unwired: 6 in, 3 out]
                  }
                }
              }
            }
            "Progress" <- w768
          }
        }
      }
    }
    n428 = local read "Flushing Sample"() -> (w134:bool)
    n429 = case shown="True" w134 {
      frame False {
      }
      frame True {
        n430 = local read "Flush Sample Start Time"() -> (w539:u32)
        n431 = local read "Sample flush time (s)"() -> (w532:dbl)
        n432 = Tick Count (ms)() -> (millisecond timer value=w540:u32)
        n433 = Subtract(x=w540, y=w539) -> (x-y=w530:u32)
        n434 = Multiply(x=u32 1000, y=w532) -> (x*y=w531:dbl)
        n435 = Divide(x=w530, y=w531) -> (x/y=w535:dbl)
        n436 = Greater?(x=w530, y=w531) -> (0:w538:bool)
        n437 = Not(x=w538) -> (.not. x?=w537:bool)
        n438 = Boolean To (0,1)(Boolean=w537) -> (0, 1=w536:i16)
        n439 = Compound Arithmetic op=MULTIPLY(w536, w535, 100.0 ("value")) -> (→"Sample Flush Meter":dbl)
        n440 = case shown="True" w538 {
          frame False {
          }
          frame True {
            w542 = FALSE ("Inject Sample")
            n441 = property on="Clear Volume" class="Bool (strict)"("Val(Sgnl)"=TRUE ("Value (Signaling)")) -> ()  [unwired: 2 in, 2 out]
            n442 = local write "Inject Sample"(w542) -> ()
            n443 = local write "Flushing Sample"(w542) -> ()
          }
        }
      }
    }
    n444 = feedback #8(0) -> (w119:i32)
    n445 = feedback #9(0) -> (w116:i32)
    n446 = feedback #10(0) -> (w121:i32)
    n447 = case shown="True" w126 {
      tunnel: w112 -> [w440 w488]
      tunnel: [w440 w472] -> w129
      tunnel: w111 -> [w439 w487]
      tunnel: [w439 w471] -> w128
      tunnel: "Raster scan" -> [w438 w464]
      tunnel: [w438 w463] -> w124
      tunnel: [0 w462] -> w122
      tunnel: w121 -> [_ w456]
      tunnel: w119 -> [_ w444]
      tunnel: [0 w447] -> w118
      tunnel: w116 -> [_ w453]
      tunnel: [0 w452] -> w115
      frame False {
      }
      frame True {
        # "Reset step counter"
        # "Current position"
        # "Initial values"
        n448 = disable-structure shown="Disabled" {
          frame Disabled {
            n449 = local write "Raster scan"(FALSE ("Raster scan")) -> ()
            n450 = property on="Reset data stream" class="Bool (strict)"("Val(Sgnl)"=TRUE) -> ()  [unwired: 2 in, 2 out]
          }
          frame Enabled {
          }
        }
        n451 = local read "Data update period (s/set)"() -> (w461:dbl)
        n452 = local read "Time per step (ms)"() -> (w458:dbl)
        n453 = local read "Trap position (V)"() -> (w443:cluster{"X":dbl, "Y":dbl})
        n454 = local read "Fixed X"() -> (w481:dbl)
        n455 = local read "Fixed Y"() -> (w482:dbl)
        n456 = Unbundle(w443) -> ("X"=w441:dbl, "Y"=w442:dbl)
        n457 = local read "Scan steps (mirror)"() -> (w470:u64)
        n458 = Multiply(x=w461, y=1000.0) -> (x*y=w459:dbl)
        n459 = local read "Stop raster"() -> (w477:bool)
        n460 = local read "Stop saving"() -> (w478:bool)
        n461 = Select(t=w481, s="Pulling direction", f=w482) -> (s? t:f=w489:dbl)
        n462 = Divide(x=w458, y=w459) -> (x/y=w457:dbl)
        n463 = Quotient & Remainder(x=w456, y=w457) -> (x-y*floor(x/y)=w455:dbl)  [unwired: 1 out]
        n464 = Not(x=w477) -> (.not. x?=w476:bool)
        n465 = Not(x=w478) -> (.not. x?=w475:bool)
        n466 = Multiply(x=u64 2, y=w470) -> (x*y=w466:u64)
        n467 = Select(t=w442, s="Pulling direction", f=w441) -> (s? t:f=w465:dbl)
        n468 = Equal To 0?(x=w455) -> (x = 0?=w454:bool)
        n469 = Less?(x=w444, y=w466) -> (x < y?=w467:bool)
        n470 = Compound Arithmetic op=AND(w467, w476, w475, w454) -> (w468:bool)
        n471 = Not(x=w467) -> (.not. x?=w450:bool)
        n472 = feedback #11() -> (w473:dbl)  [unwired: 1 in]
        n473 = case shown="True" w468 {
          tunnel: w489 -> [_ w525]
          tunnel: w465 -> [_ w507]
          tunnel: w488 -> [w502 w524]
          tunnel: w487 -> [w501 w523]
          tunnel: [w502 w522] -> w472
          tunnel: [w501 w521] -> w471
          tunnel: [w498 w510] -> w474
          tunnel: w444 -> [w499 w505]
          tunnel: w473 -> [w498 w504]
          tunnel: w464 -> [w500 w509]
          tunnel: [w500 w509] -> w463
          tunnel: [w499 w508] -> w448
          frame False {
          }
          frame True {
            # "Go forward or backward?"
            n474 = local read "Scan increment (V)"() -> (w503:dbl)
            n475 = local read "Scan steps (mirror)"() -> (w514:u64)
            n476 = Multiply(x=w503, y=w505) -> (x*y=w506:dbl)
            n477 = Less?(x=w505, y=w514) -> (x < y?=w513:bool)
            n478 = Add(x=w507, y=w506) -> (x+y=w516:dbl)
            n479 = Subtract(x=w504, y=w503) -> (x-y=w515:dbl)
            n480 = Select(t=w516, s=w513, f=w515) -> (s? t:f=w510:dbl)
            n481 = local read "Pulling direction"() -> (w512:bool)
            n482 = Build Array(w510, w525) -> (w519:dbl[])
            n483 = Build Array(w525, w510) -> (w518:dbl[])
            n484 = Select(t=w519, s=w512, f=w518) -> (s? t:f=w517:dbl[])
            n485 = call-poly <vilib>:"DAQmx Write.vi"("task/channels in"=w524, "auto start"=TRUE, "data"=w517, "error in"=w523) -> ("task out"=w522:refnum<k21>, "error out"=w521:errorcluster)  [unwired: 9 in, 1 out]
            n486 = Increment(x=w505) -> (x+1=w508:i32)
            "Raster scanning..." <- TRUE ("Raster scanning...")
          }
        }
        n487 = feedback-in #11(w474) -> ()
        n488 = case shown="True" w450 {
          tunnel: w453 -> [w495 w497]
          tunnel: [w495 w496] -> w452
          frame False {
          }
          frame True {
            n489 = Increment(x=w497) -> (x+1=w496:i32)
          }
        }
        n490 = local read "# scans"() -> (w451:i32)
        n491 = local read "Stop saving"() -> (w480:bool)
        n492 = Greater Or Equal?(x=w452, y=w451) -> (x >= y?=w445:bool)
        n493 = Not(x=w445) -> (.not. x?=w446:bool)
        n494 = And(x=w450, y=w446) -> (x .and. y?=w449:bool)
        n495 = Compound Arithmetic op=OR(w445, "Stop raster", w480) -> (w483:bool)
        n496 = case shown="True" w483 {
          frame False {
          }
          frame True {
            n497 = flat-sequence {
              frame #0 {
                n498 = Wait (ms)(milliseconds to wait=u32 300) -> ()  [unwired: 1 out]
              }
              frame #1 {
                n499 = property on="Trap delta (nm)" class="DigNum (strict)"("Val(Sgnl)"="Trap delta\nafter (nm)") -> ()  [unwired: 2 in, 2 out]
              }
            }
          }
        }
        n500 = And(x="Flow on\nafter raster?", y=w483) -> (x .and. y?=w484:bool)
        n501 = case shown="True" w484 {
          frame False {
          }
          frame True {
            n502 = property on="Inject Sample" class="Bool (strict)"("Val(Sgnl)"=TRUE ("Value (Signaling)")) -> ()  [unwired: 2 in, 2 out]
          }
        }
        n503 = case shown="True" w449 {
          tunnel: w448 -> [w493 _]
          tunnel: [w493 0] -> w447
          frame False {
          }
          frame True {
          }
        }
        n504 = Not(x=w483) -> (.not. x?=w486:bool)
        n505 = local write "Raster scanning..."(w486) -> ()
        n506 = Increment(x=w456) -> (x+1=w462:i32)
      }
    }
    n507 = And(x="Save scans", y=w124) -> (x .and. y?=w132:bool)
    n508 = feedback-in #8(w118) -> ()
    n509 = feedback-in #9(w115) -> ()
    n510 = feedback-in #10(w122) -> ()
    n511 = local read "Stop"() -> (w429:bool)
  }
  n512 = local write "Progress"(u8 0 ("Progress")) -> ()
  n513 = local write "Calibrating"(FALSE ("Calibrating")) -> ()
  n514 = call "InitializeChamberImage.vi"() -> ("error out"=w101:errorcluster, "IMAQ Session Out"=w102:refnum<k11>, "Display Out"=w103:T6, "Acquired Image"=w9:T6)  [unwired: 8 in]
  n515 = node-c288(i64 10 ("Period"), 2 ("Processor")) -> (w15:T11)  [unwired: 2 in]
  n516 = timed-loop {
    tunnel: w103 -> [w865]
    tunnel: w102 -> [w864]
    tunnel: w101 -> [w863]
    tunnel: [w861] -> w100
    tunnel: [w860] -> w99
    timing: w15 -> [_]
    timing-out: [_] -> w14
    i -> [w862]
    stop <- w856 continue-if-true
    n517 = node-c288() -> ()  [unwired: 1 in, 1 out]
    n518 = call <vilib>:"IMAQ Copy Acquired Buffer.vi"("IMAQ Session In"=w864, "Image In"=w865, "Buffer Number"=w862, "error in (no error)"=w863) -> ("IMAQ Session Out"=w861:refnum<k11>, "Image Out"=→"Chamber":T6, "error out"=w860:errorcluster)  [unwired: 7 in, 2 out]
    "Video Error" <- w860
    n519 = local read "Stop"() -> (w858:bool)
    n520 = Unbundle By Name(w860) -> ("status"=w859:bool)
    n521 = Not Or(1:w858, 2:w859) -> (0:w856:bool)
    "Continue to display?" <- w856
    n522 = node-c288() -> ()  [unwired: 1 in, 1 out]
  }
  n523 = node-c288(w14) -> ()  [unwired: 1 out]
  n524 = call <vilib>:"IMAQ Close.vi"("error in (no error)"=w99, "IMAQ Session In"=w100) -> ("error out"=w107:errorcluster)  [unwired: 9 in]
  n525 = call "IMAQ Dispose"("error in (no error)"=w107) -> ("error out"=w106:errorcluster)  [unwired: 5 in]
  n526 = call-poly "VISA Configure Serial Port"("VISA resource name"=refnum<visa-resource-name> "COM3") -> ("VISA resource name out"=w21:refnum<visa-resource-name>, "error out"=w20:errorcluster)  [unwired: 13 in]
  n527 = call "IMAQ Dispose"("Image"=w9, "error in (no error)"=w106) -> ("error out"=w105:errorcluster)  [unwired: 4 in]
  n528 = node-c288(i64 100 ("Period"), 2 ("Processor")) -> (w23:T11)  [unwired: 2 in]
  n529 = call <vilib>:"Simple Error Handler.vi"("error in (no error)"=w105) -> ()  [unwired: 4 in, 5 out]
  n530 = timed-loop {
    timing: w23 -> [_]
    timing-out: [_] -> w22
    tunnel: w21 -> [w868]
    tunnel: w20 -> [w870]
    tunnel: [w868] -> w19
    stop <- w869 stop-if-true
    n531 = node-c288() -> ()  [unwired: 1 in, 1 out]
    n532 = event shown="[0] \"Got DNA bead\": Value Change" {
      selector: _ -> [_ _ _ _ _ _ _ _ _ _ _]
      dyn-events: _ -> [_ _ _ _ _ _ _ _ _ _ _]
      timeout: _ -> [_ _ _ _ _ _ _ _ _ _ _]
      tunnel: w868 -> [w877 w916 w936 w953 w970 w989 w1009 _ _ _ _]
      tunnel: w870 -> [w876 w915 w935 w952 w969 w988 w1008 _ _ _ _]
      tunnel: [_ _ _ _ _ _ _ _ _ _ w1062] -> w869
      event "Got DNA bead": Value Change {
        n533 = event-data() -> ()  [unwired: 1 in, 5 out]
        n534 = flat-sequence {
          tunnel: w877 -> [w881]
          tunnel: w876 -> [w879]
          tunnel: [w896] -> w875
          tunnel: w875 -> [w899]
          tunnel: [w899] -> w874
          tunnel: w874 -> [w901]
          tunnel: [w901] -> w873
          tunnel: w873 -> [w905]
          tunnel: [w905] -> w872
          tunnel: w872 -> [w907]
          tunnel: [w907] -> w871
          tunnel: w871 -> [w909]
          frame #0 {
            n535 = local read "Saved stage positions"() -> (w882:dbl[][])
            n536 = disable-structure shown="Disabled" {
              frame Disabled {
                n537 = property on="Inject Pump 2" class="Bool (strict)"("Val(Sgnl)"=FALSE ("Inject Pump 2")) -> ()  [unwired: 2 in, 2 out]
              }
              frame Enabled {
              }
            }
            n538 = property on="Inject Sample" class="Bool (strict)"("Val(Sgnl)"=TRUE ("Value (Signaling)")) -> ()  [unwired: 2 in, 2 out]
            n539 = local write "Stage moving"(TRUE ("Stage moving")) -> ()
            n540 = property on="Trap delta (nm)" class="DigNum (strict)"("Val(Sgnl)"="Cal @ Delta (nm)") -> ()  [unwired: 2 in, 2 out]
            n541 = call "move to saved stage position.vi"("error in"=w879, "Stage VISA resource name in"=w881, "Position"="Cal stage position", "Saved Stage Positions"=w882) -> ()  [unwired: 2 out]
          }
          frame #1 {
            n542 = local write "Stage moving"(FALSE ("Stage moving")) -> ()
            n543 = property on="Inject Sample" class="Bool (strict)"("Val(Sgnl)"=FALSE ("Value (Signaling)")) -> ()  [unwired: 2 in, 2 out]
            n544 = call <vilib>:"Beep.vi"() -> ()  [unwired: 12 in]
          }
          frame #2 {
            n545 = Wait (ms)(milliseconds to wait=u32 1000) -> ()  [unwired: 1 out]
          }
          frame #3 {
            n546 = property on="Save cal" class="Bool (strict)"("Val(Sgnl)"=TRUE ("Value (Signaling)")) -> ()  [unwired: 2 in, 2 out]
          }
          frame #4 {
            n547 = Wait (ms)(milliseconds to wait=u32 2000) -> ()  [unwired: 1 out]
          }
          frame #5 {
            n548 = while {
              stop <- w892 stop-if-true
              n549 = local read "Saving"() -> (w893:bool)
              n550 = Not(x=w893) -> (.not. x?=w892:bool)
              n551 = Wait (ms)(milliseconds to wait=u32 100) -> ()  [unwired: 1 out]
            }
          }
          frame #6 {
            n552 = Wait (ms)(milliseconds to wait=u32 2000) -> ()  [unwired: 1 out]
            n553 = property on="Trap delta (nm)" class="DigNum (strict)"("Val(Sgnl)"="Offset @ Delta (nm)") -> ()  [unwired: 2 in, 2 out]
          }
          frame #7 {
            # "Only continue if there is no buffer\noverflow error"
            n554 = local read "Buffer Overflow"() -> (w897:bool)
            n555 = Not(x=w897) -> (.not. x?=w896:bool)
            n556 = case shown="True" w896 {
              frame False {
              }
              frame True {
                n557 = property on="Raster scan" class="Bool (strict)"("Val(Sgnl)"=TRUE ("Value (Signaling)")) -> ()  [unwired: 2 in, 2 out]
              }
            }
          }
          frame #8 {
            n558 = case shown="True" w899 {
              frame False {
              }
              frame True {
                n559 = Wait (ms)(milliseconds to wait=u32 2000) -> ()  [unwired: 1 out]
              }
            }
          }
          frame #9 {
            n560 = case shown="True" w901 {
              frame False {
              }
              frame True {
                n561 = while {
                  stop <- w903 stop-if-true
                  n562 = local read "Saving"() -> (w904:bool)
                  n563 = Not(x=w904) -> (.not. x?=w903:bool)
                  n564 = Wait (ms)(milliseconds to wait=u32 100) -> ()  [unwired: 1 out]
                }
              }
            }
          }
          frame #10 {
            n565 = case shown="True" w905 {
              frame False {
              }
              frame True {
                n566 = property on="Read Cal" class="Bool (strict)"("Val(Sgnl)"=TRUE ("Value (Signaling)")) -> ()  [unwired: 2 in, 2 out]
              }
            }
          }
          frame #11 {
            n567 = case shown="True" w907 {
              frame False {
              }
              frame True {
                n568 = Wait (ms)(milliseconds to wait=u32 1000) -> ()  [unwired: 1 out]
              }
            }
          }
          frame #12 {
            n569 = case shown="True" w909 {
              frame False {
              }
              frame True {
                n570 = property on="Fish" class="Bool (strict)"("Val(Sgnl)"=TRUE ("Value (Signaling)")) -> ()  [unwired: 2 in, 2 out]
                n571 = case shown="True" "Flow on\nwhile fish?" {
                  frame False {
                  }
                  frame True {
                    n572 = property on="Inject Sample" class="Bool (strict)"("Val(Sgnl)"=TRUE ("Value (Signaling)")) -> ()  [unwired: 2 in, 2 out]
                  }
                }
              }
            }
          }
        }
      }
      event "Dump beads": Value Change {
        n573 = event-data() -> ()  [unwired: 1 in, 5 out]
        n574 = flat-sequence {
          tunnel: w915 -> [w919]
          tunnel: w916 -> [w920]
          tunnel: [w920] -> w914
          tunnel: [w919] -> w913
          tunnel: w914 -> [w923]
          tunnel: w913 -> [w922]
          frame #0 {
            w917 = FALSE ("Fish")
            n575 = local read "Saving"() -> (w918:bool)
            n576 = local write "Pause dwell"(w917) -> ()
            n577 = local write "Force Feedback"(w917) -> ()
            n578 = local write "Dump beads"(w917) -> ()
            n579 = property on="Stop saving" class="Bool (strict)"("Val(Sgnl)"=w918) -> ()  [unwired: 2 in, 2 out]
            n580 = local write "Fish"(w917) -> ()
          }
          frame #1 {
            n581 = local read "Saved stage positions"() -> (w925:dbl[][])
            n582 = case shown="True" "Flow on\ndump?" {
              frame False {
              }
              frame True {
                n583 = property on="Inject Sample" class="Bool (strict)"("Val(Sgnl)"=TRUE ("Value (Signaling)")) -> ()  [unwired: 2 in, 2 out]
              }
            }
            n584 = local write "Stage moving"(TRUE ("Stage moving")) -> ()
            n585 = call "move to saved stage position.vi"("error in"=w922, "Stage VISA resource name in"=w923, "Position"=5, "Saved Stage Positions"=w925) -> ()  [unwired: 2 out]
          }
          frame #2 {
            n586 = local read "Shutter 1 (B)"() -> (w930:bool)
            n587 = local read "Shutter 2 (A)"() -> (w929:bool)
            n588 = call <vilib>:"Beep.vi"() -> ()  [unwired: 12 in]
            n589 = case shown="True" w930 {
              frame False {
              }
              frame True {
                n590 = property on="Shutter 1 (B)" class="Bool (strict)"("Val(Sgnl)"=FALSE ("Value (Signaling)")) -> ()  [unwired: 2 in, 2 out]
              }
            }
            n591 = case shown="True" w929 {
              frame False {
              }
              frame True {
                n592 = property on="Shutter 2 (A)" class="Bool (strict)"("Val(Sgnl)"=FALSE) -> ()  [unwired: 2 in, 2 out]
              }
            }
            n593 = local write "Stage moving"(FALSE ("Stage moving")) -> ()
            n594 = local write "Tether"(FALSE ("Tether")) -> ()
          }
          frame #3 {
            n595 = property on="Move Cap. 2 (ADig Top)" class="Bool (strict)"("Val(Sgnl)"=TRUE ("Value (Signaling)")) -> ()  [unwired: 2 in, 2 out]
          }
        }
      }
      event "Move Cap. 2 (ADig Top)": Value Change {
        n596 = event-data() -> ()  [unwired: 1 in, 5 out]
        n597 = flat-sequence {
          tunnel: w936 -> [w940]
          tunnel: w935 -> [w939]
          frame #0 {
            n598 = local read "Saved stage positions"() -> (w938:dbl[][])
            n599 = case shown="True" "Flow on\ncap 2?" {
              frame False {
              }
              frame True {
                n600 = property on="Inject Sample" class="Bool (strict)"("Val(Sgnl)"=TRUE ("Value (Signaling)")) -> ()  [unwired: 2 in, 2 out]
              }
            }
            n601 = local write "Move Cap. 2 (ADig Top)"(FALSE ("Move Cap. 2 (ADig Top)")) -> ()
            n602 = local write "Stage moving"(TRUE ("Stage moving")) -> ()
            n603 = call "move to saved stage position.vi"("error in"=w939, "Stage VISA resource name in"=w940, "Position"=2, "Saved Stage Positions"=w938) -> ()  [unwired: 2 out]
          }
          frame #1 {
            # "Make sure you don't reverse\nwhich is ON and OFF"
            n604 = local read "Cal @ Delta (nm)"() -> (w947:dbl)
            n605 = local write "Stage moving"(FALSE ("Stage moving")) -> ()
            n606 = call <vilib>:"Beep.vi"() -> ()  [unwired: 12 in]
            n607 = property on="Trap delta (nm)" class="DigNum (strict)"("Val(Sgnl)"=w947) -> ()  [unwired: 2 in, 2 out]
            n608 = disable-structure shown="Disabled" {
              frame Disabled {
                n609 = property on="Inject Pump 1" class="Bool (strict)"("Val(Sgnl)"=TRUE ("Inject Pump 2")) -> ()  [unwired: 2 in, 2 out]
              }
              frame Enabled {
              }
            }
            n610 = local read "Shutter 2 (A)"() -> (w946:bool)
            n611 = case shown="False" w946 {
              frame False {
                n612 = property on="Shutter 2 (A)" class="Bool (strict)"("Val(Sgnl)"=TRUE ("Value (Signaling)")) -> ()  [unwired: 2 in, 2 out]
              }
              frame True {
              }
            }
            n613 = property on="Inject Sample" class="Bool (strict)"("Val(Sgnl)"=FALSE ("Value (Signaling)")) -> ()  [unwired: 2 in, 2 out]
          }
        }
      }
      event "Got ADig bead": Value Change {
        n614 = event-data() -> ()  [unwired: 1 in, 5 out]
        n615 = flat-sequence {
          tunnel: w953 -> [w957]
          tunnel: w952 -> [w956]
          frame #0 {
            n616 = local read "Saved stage positions"() -> (w959:dbl[][])
            n617 = property on="Inject Pump 1" class="Bool (strict)"("Val(Sgnl)"=FALSE ("Inject Pump 2")) -> ()  [unwired: 2 in, 2 out]
            n618 = case shown="True" "Flow on\ncap 1?" {
              frame False {
              }
              frame True {
                n619 = property on="Inject Sample" class="Bool (strict)"("Val(Sgnl)"=TRUE ("Value (Signaling)")) -> ()  [unwired: 2 in, 2 out]
              }
            }
            n620 = local write "Stage moving"(TRUE ("Stage moving")) -> ()
            n621 = call "move to saved stage position.vi"("error in"=w956, "Stage VISA resource name in"=w957, "Position"=1, "Saved Stage Positions"=w959) -> ()  [unwired: 2 out]
          }
          frame #1 {
            n622 = local read "Shutter 1 (B)"() -> (w963:bool)
            n623 = disable-structure shown="Disabled" {
              frame Disabled {
                n624 = property on="Inject Pump 2" class="Bool (strict)"("Val(Sgnl)"=TRUE ("Inject Pump 2")) -> ()  [unwired: 2 in, 2 out]
              }
              frame Enabled {
              }
            }
            n625 = local write "Stage moving"(FALSE ("Stage moving")) -> ()
            n626 = case shown="False" w963 {
              frame False {
                n627 = property on="Shutter 1 (B)" class="Bool (strict)"("Val(Sgnl)"=TRUE ("Value (Signaling)")) -> ()  [unwired: 2 in, 2 out]
              }
              frame True {
              }
            }
            n628 = property on="Inject Sample" class="Bool (strict)"("Val(Sgnl)"=FALSE ("Value (Signaling)")) -> ()  [unwired: 2 in, 2 out]
            n629 = call <vilib>:"Beep.vi"() -> ()  [unwired: 12 in]
          }
        }
        n630 = local write "Got ADig bead"(FALSE ("Got ADig bead")) -> ()
      }
      event "Set Position 1", "Set Position 2", "Set Position 3", "Set Position 4", "Set Position 5": Value Change {
        n631 = event-data() -> ()  [unwired: 1 in, 5 out]
        n632 = Build Array("Set Position 1", "Set Position 2", "Set Position 3", "Set Position 4", "Set Position 5") -> (w982:bool[])
        n633 = Boolean Array To Number(Boolean array=w982) -> (number=w981:u32)
        n634 = call "Read Stage Position.vi"("error in"=w969, "VISA resource name in"=w970) -> ("Current Position"=w967:cluster{dbl, dbl, dbl}, "error out"=→"Stage error":errorcluster)  [unwired: 1 in, 1 out]
        n635 = Logarithm Base 2(1:w981) -> (0:w975:dbl)
        n636 = Cluster To Array(cluster=w967) -> (array=w977:dbl[])
        n637 = Increment(x=w975) -> (x+1=w978:dbl)
        n638 = Build Array (concatenate)(w978, w977) -> (w976:dbl[])
        n639 = Replace Array Subset(array="Saved stage positions", new element=w976, index (row)=w975) -> (w979:dbl[][])  [unwired: 1 in]
        n640 = local write "Saved stage positions"(w979) -> ()
      }
      event "Move to Position 2", "Move to Position 4", "Move to Position 3", "Move to Position 5", "Move to Position 1": Value Change {
        n641 = event-data() -> ()  [unwired: 1 in, 5 out]
        n642 = Build Array("Move to Position 1", "Move to Position 2", "Move to Position 3", "Move to Position 4", "Move to Position 5") -> (w992:bool[])
        n643 = Boolean Array To Number(Boolean array=w992) -> (number=w991:u32)
        n644 = Logarithm Base 2(1:w991) -> (0:w990:dbl)
        n645 = flat-sequence {
          tunnel: w990 -> [w997]
          tunnel: w989 -> [w996]
          tunnel: w988 -> [w995]
          frame #0 {
            n646 = local read "Saved stage positions"() -> (w998:dbl[][])
            n647 = Increment(x=w997) -> (x+1=w994:dbl)
            n648 = call "move to saved stage position.vi"("error in"=w995, "Stage VISA resource name in"=w996, "Position"=w994, "Saved Stage Positions"=w998) -> ()  [unwired: 2 out]
            "Stage moving" <- TRUE ("Stage moving")
          }
          frame #1 {
            n649 = call <vilib>:"Beep.vi"() -> ()  [unwired: 12 in]
            n650 = local write "Stage moving"(FALSE ("Stage moving")) -> ()
          }
        }
      }
      event "Dip": Value Change {
        n651 = event-data() -> ()  [unwired: 1 in, 5 out]
        n652 = local write "Dip"(FALSE ("Dip")) -> ()
        n653 = flat-sequence {
          tunnel: w1009 -> [w1011]
          tunnel: w1008 -> [w1010]
          tunnel: [w1012] -> w1006
          tunnel: [w1011] -> w1004
          tunnel: [w1010] -> w1002
          tunnel: [w1020] -> w1007
          tunnel: w1006 -> [w1020]
          tunnel: [w1019] -> w1005
          tunnel: w1004 -> [w1019]
          tunnel: [w1018] -> w1003
          tunnel: w1002 -> [w1018]
          tunnel: w1007 -> [w1039]
          tunnel: w1005 -> [w1038]
          tunnel: w1003 -> [w1037]
          frame #0 {
            n654 = local read "Saved stage positions"() -> (w1012:dbl[][])
            n655 = local write "Stage moving"(TRUE) -> ()
            n656 = call "move to saved stage position.vi"("error in"=w1010, "Stage VISA resource name in"=w1011, "Position"="Dip position", "Saved Stage Positions"=w1012) -> ()  [unwired: 2 out]
          }
          frame #1 {
            n657 = node-c288() -> (w1017:T11)  [unwired: 4 in]
            n658 = timed-loop {
              timing: w1017 -> [_]
              timing-out: [_] -> w1016
              i -> [w1030]
              stop <- w1021 stop-if-true
              n659 = node-c288() -> ()  [unwired: 1 in, 1 out]
              n660 = Greater Or Equal?(x=w1030, y="Dip duration") -> (x >= y?=w1026:bool)
              n661 = local read "Dump beads"() -> (w1023:bool)
              n662 = Or(x=w1026, y="Cancel dwell") -> (x .or. y?=w1024:bool)
              n663 = Not(x="Pause dwell") -> (.not. x?=w1027:bool)
              n664 = node-c288() -> ()  [unwired: 1 in, 1 out]
              n665 = And(x=w1027, y=w1024) -> (x .and. y?=w1022:bool)
              n666 = Or(x=w1022, y=w1023) -> (x .or. y?=w1021:bool)
              "Dip time" <- w1030
            }
            n667 = local write "Stage moving"(FALSE ("Stage moving")) -> ()
            n668 = node-c288(w1016) -> ()  [unwired: 1 out]
          }
          frame #2 {
            n669 = local write "Cancel dwell"(FALSE ("Cancel dwell")) -> ()
            n670 = call "move to saved stage position.vi"("error in"=w1037, "Stage VISA resource name in"=w1038, "Position"="Return position", "Saved Stage Positions"=w1039) -> ()  [unwired: 2 out]
          }
          frame #3 {
            n671 = local write "Stage moving"(FALSE ("Stage moving")) -> ()
          }
        }
      }
      event "Force FB script": Value Change {
        n672 = event-data() -> ()  [unwired: 1 in, 5 out]
        n673 = flat-sequence {
          frame #0 {
            n674 = disable-structure shown="Disabled" {
              frame Disabled {
                n675 = local read "# Samples/channel"() -> (w1043:i32)
                n676 = local write "# Samples/channel (in)"(w1043) -> ()
              }
              frame Enabled {
              }
            }
            n677 = local write "Force FB script"(FALSE ("Force FB script")) -> ()
            n678 = property on="Trap delta (nm)" class="DigNum (strict)"("Val(Sgnl)"="Start trap delta (nm)") -> ()  [unwired: 2 in, 2 out]
          }
          frame #1 {
            n679 = Wait (ms)(milliseconds to wait=u32 500) -> ()  [unwired: 1 out]
          }
          frame #2 {
            n680 = property on="Set Initial Delta" class="Bool (strict)"("Val(Sgnl)"=TRUE ("Value (Signaling)")) -> ()  [unwired: 2 in, 2 out]
          }
          frame #3 {
            n681 = Wait (ms)(milliseconds to wait=u32 300) -> ()  [unwired: 1 out]
          }
          frame #4 {
            n682 = local write "Force Feedback"(TRUE ("Force Feedback")) -> ()
            n683 = property on="Tabs" class="TabCtl (strict)"("Val(Sgnl)"=T3."Force Feedback" ("Value (Signaling)")) -> ()  [unwired: 2 in, 2 out]
          }
          frame #5 {
            n684 = property on="Save Data" class="Bool (strict)"("Val(Sgnl)"=TRUE ("Value (Signaling)")) -> ()  [unwired: 2 in, 2 out]
          }
          frame #6 {
            n685 = Multiply(x="Wait before dip (s)", y=1000) -> (x*y=w1050:dbl)
            n686 = Wait (ms)(milliseconds to wait=w1050) -> ()  [unwired: 1 out]
          }
          frame #7 {
            n687 = case shown="True" "Start dipping after?" {
              selector: "Start dipping after?" -> [_ w1055]
              frame False {
              }
              frame True {
                n688 = property on="Dip" class="Bool (strict)"("Val(Sgnl)"=w1055) -> ()  [unwired: 2 in, 2 out]
              }
            }
            n689 = property on="Remove offsets" class="Bool (strict)"("Val(Sgnl)"=TRUE ("Value (Signaling)")) -> ()  [unwired: 2 in, 2 out]
          }
        }
      }
      event "Move 0": Value Change {
        n690 = event-data() -> ()  [unwired: 1 in, 5 out]
        n691 = local write "Move 0"(FALSE) -> ()
        n692 = call "HalfWavePlate.vi"("Degrees"="\"Degrees\" 0", "Motor"=0) -> ()  [unwired: 1 in]
      }
      event "Move 1": Value Change {
        n693 = event-data() -> ()  [unwired: 1 in, 5 out]
        n694 = local write "Move 1"(FALSE) -> ()
        n695 = call "HalfWavePlate.vi"("Degrees"="\"Degrees\" 1", "Motor"=1) -> ()  [unwired: 1 in]
      }
      event "Stop": Value Change {
        n696 = event-data() -> ()  [unwired: 1 in, 5 out]
        n697 = local read "Stop"() -> (w1062:bool)
      }
    }
    n698 = node-c288() -> ()  [unwired: 1 in, 1 out]
  }
  n699 = node-c288(2 ("Processor")) -> (w75:T11)  [unwired: 3 in]
  n700 = node-c288(2 ("Processor")) -> (w27:T11)  [unwired: 3 in]
  n701 = timed-loop {
    timing: w75 -> [_]
    timing-out: [_] -> w74
    stop <- w1065 stop-if-true
    n702 = node-c288() -> ()  [unwired: 1 in, 1 out]
    n703 = case shown="\"Current Saved Data\"" "Tab Control" {
      frame "Control" {
        n704 = case shown="True" "Start" {
          frame False {
          }
          frame True {
            w1078 = T14 3 items=["no dialog", "OK message", "continue or stop message", "OK message + warnings", "continue/stop + warnings"] ("type of dialog (OK msg:1)")
            n705 = call "InitializeAcquireFF.vi"("DAQ Rate"="DAQ Rate", "Averaging Number"="Averaging Number", "Sampling Rate"="Sampling Rate") -> ("error out"=w1072:errorcluster, "task out"=w1071:refnum<k21>, "Final Sampling Rate"=→"Final Sampling Rate":dbl)  [unwired: 4 in, 2 out]
            n706 = while {
              tunnel: [w1090] -> w1077
              tunnel: [w1089] -> w1070
              tunnel: "Averaging Number" -> [w1088]
              tunnel: w1072 -> [w1087]
              tunnel: w1071 -> [w1085]
              stop <- w1086 continue-if-true
              n707 = call "Acquire2_QPD.vi"("task/channels in"=w1085, "Save Data?"=FALSE ("Take Data?"), "Averaging Number"=w1088, "error in"=w1087) -> ("PSD 1"=→"PSD 1":cluster{dbl[], dbl[]}, "PSD 1 Sum"=→"PSD 1 Sum":dbl, "PSD 2"=→"PSD 2":cluster{dbl[], dbl[]}, "PSD 2 Sum"=→"PSD 2 Sum":dbl, "task out"=w1090:refnum<k21>, "error out"=w1089:errorcluster)  [unwired: 14 in, 4 out]
              n708 = local read "Start"() -> (w1086:bool)
            }
            n709 = call <vilib>:"DAQmx Clear Task.vi"("task in"=w1077, "error in"=w1070) -> ("error out"=w1079:errorcluster)  [unwired: 13 in]
            n710 = call <vilib>:"Simple Error Handler.vi"("type of dialog (OK msg:1)"=w1078, "error in (no error)"=w1079) -> ()  [unwired: 3 in, 5 out]
          }
        }
      }
      frame "Current Saved Data" {
      }
      frame "Data Acquisition" {
      }
      frame "Raw QPD Data" {
      }
    }
    n711 = local read "Stop"() -> (w1065:bool)
    n712 = node-c288() -> ()  [unwired: 1 in, 1 out]
  }
  n713 = call-poly <vilib>:"DAQmx Create Virtual Channel.vi"("lines"=w92) -> ("task out"=w91:refnum<k21>)  [unwired: 13 in, 1 out]
  n714 = call-poly <vilib>:"DAQmx Create Virtual Channel.vi"("lines"=w95) -> ("task out"=w94:refnum<k21>)  [unwired: 13 in, 1 out]
  n715 = timed-loop {
    timing: w27 -> [_]
    timing-out: [_] -> w26
    stop <- w1091 stop-if-true
    n716 = node-c288() -> ()  [unwired: 1 in, 1 out]
    n717 = event shown="[0] \"Pause Mouse/Mirror Connection\": Value Change" {
      selector: _ -> [_ _]
      dyn-events: _ -> [_ _]
      timeout: _ -> [_ _]
      tunnel: [w1184 _] -> w1092
      tunnel: [_ w1185] -> w1091
      event "Pause Mouse/Mirror Connection": Value Change {
        n718 = event-data() -> ("NewVal"=w1184:bool)  [unwired: 1 in]
      }
      event "Stop": Value Change {
        n719 = event-data() -> ("NewVal"=w1185:bool)  [unwired: 1 in]
      }
    }
    n720 = case shown="True" w1092 {
      frame False {
      }
      frame True {
        n721 = call "InitializeMouseControl.vi"() -> ("error out 2"=w1101:errorcluster, "task out"=w1102:refnum<k21>, "error out"=w1104:errorcluster, "device ID"=w1103:refnum<k1>)  [unwired: 8 in]
        n722 = while {
          tunnel: w1104 -> [w1116]
          tunnel: w1103 -> [w1115]
          tunnel: w1102 -> [w1114]
          tunnel: w1101 -> [w1113]
          tunnel: [w1112] -> w1099
          tunnel: [w1111] -> w1098
          tunnel: [w1110] -> w1095
          tunnel: [w1109] -> w1096
          stop <- w1108 stop-if-true
          n723 = case shown="True" "Use Mouse to Move Trap?" {
            tunnel: w1115 -> [w1123 w1146]
            tunnel: w1116 -> [w1122 w1145]
            tunnel: w1114 -> [w1121 w1144]
            tunnel: w1113 -> [w1120 w1143]
            tunnel: [w1123 w1142] -> w1110
            tunnel: [w1122 w1141] -> w1109
            tunnel: [w1121 w1140] -> w1112
            tunnel: [w1120 w1139] -> w1111
            frame False {
              (unwired) FALSE ("button 1")
            }
            frame True {
              w1134 = 0.0 ("y")
              w1136 = 10
              n724 = local read "Deflection"() -> (w1147:T4)
              n725 = call-poly <vilib>:"Acquire Input Data.vi"("device ID"=w1146, "error in (no error)"=w1145) -> ("device ID"=w1142:refnum<k1>, "button info"=w1160:T15, "error out"=w1141:errorcluster)  [unwired: 14 in, 1 out]
              n726 = Unbundle By Name(w1147) -> ("Horizontal"=w1149:i32, "Vertical"=w1148:i32)
              n727 = local read "Saved voltage"() -> (w1125:cluster{dbl, dbl})
              n728 = Divide(x=w1149, y=30) -> (x/y=w1152:dbl)
              n729 = Divide(x=w1148, y=-20) -> (x/y=w1153:dbl)
              n730 = Unbundle By Name(w1160) -> ("button 1"=w1138:bool, "button 2"=w1154:bool)
              n731 = Bundle(w1152, w1153) -> (w1130:cluster{dbl, dbl})  [unwired: 1 in]
              n732 = local write "Reference Voltage"(w1130) -> ()
              n733 = Add(x=w1130, y=w1125) -> (x+y=w1158:cluster{dbl, dbl})
              n734 = case shown="True" w1138 {
                frame False {
                  n735 = stacked-sequence {
                    frame #0 {
                      n736 = local write "CoordinatesMousePressed"(T4 {"Horizontal"=0, "Vertical"=0} ("Coords when pressed")) -> ()
                      n737 = local write "Deflection"(T4 {"Horizontal"=0, "Vertical"=0} ("deflaction")) -> ()
                    }
                  }
                }
                frame True {
                  n738 = local read "CoordinatesMousePressed"() -> (w1183:T4)
                  n739 = local read "Real Coordinates"() -> (w1182:cluster{"Horizontal":i32, "Vertical":i32})
                  n740 = Subtract(x=w1182, y=w1183) -> (x-y=w1181:T4)
                  n741 = local write "Deflection"(w1181) -> ()
                }
              }
              n742 = Unbundle(w1158) -> (w1135:dbl, w1126:dbl)
              n743 = case shown="True" w1154 {
                frame False {
                }
                frame True {
                  n744 = local read "Reference Voltage"() -> (w1164:cluster{dbl, dbl})
                  n745 = local read "Saved voltage"() -> (w1162:cluster{dbl, dbl})
                  n746 = Add(x=w1164, y=w1162) -> (x+y=→"Saved voltage":cluster{dbl, dbl})
                  n747 = local read "Real Coordinates"() -> (w1163:cluster{"Horizontal":i32, "Vertical":i32})
                  n748 = local write "CoordinatesMousePressed"(w1163) -> ()
                }
              }
              n749 = Less?(x=w1135, y=w1136) -> (x < y?=w1133:bool)
              n750 = Greater?(x=w1135, y=w1134) -> (0:w1132:bool)
              n751 = Greater?(x=w1126, y=w1134) -> (0:w1128:bool)
              n752 = Less?(x=w1126, y=w1136) -> (x < y?=w1129:bool)
              n753 = And(x=w1128, y=w1129) -> (x .and. y?=w1127:bool)
              n754 = And(x=w1133, y=w1132) -> (x .and. y?=w1131:bool)
              n755 = case shown="False" w1127 {
                tunnel: [w1174 w1178] -> w1137
                tunnel: w1126 -> [w1172 w1178]
                frame False {
                  n756 = Greater?(x=w1172, y=10.0) -> (0:w1175:bool)
                  n757 = case shown="True" w1175 {
                    tunnel: [0.0 10.0] -> w1174
                    frame False {
                    }
                    frame True {
                    }
                  }
                }
                frame True {
                }
              }
              n758 = case shown="False" w1131 {
                tunnel: w1135 -> [w1166 w1171]
                tunnel: [w1167 w1171] -> w1159
                frame False {
                  n759 = Greater?(x=w1166, y=10.0) -> (0:w1168:bool)
                  n760 = case shown="True" w1168 {
                    tunnel: [0.0 10.0] -> w1167
                    frame False {
                    }
                    frame True {
                    }
                  }
                }
                frame True {
                }
              }
              n761 = Bundle(w1159, w1137) -> (w1124:cluster{dbl, dbl})  [unwired: 1 in]
              n762 = Cluster To Array(cluster=w1124) -> (array=w1155:dbl[])
              n763 = call-poly <vilib>:"DAQmx Write.vi"("task/channels in"=w1144, "data"=w1155, "error in"=w1143) -> ("task out"=w1157:refnum<k21>, "error out"=w1156:errorcluster)  [unwired: 10 in, 1 out]
              n764 = call <vilib>:"DAQmx Is Task Done.vi"("task/channels in"=w1157, "error in"=w1156) -> ("task out"=w1140:refnum<k21>, "error out"=w1139:errorcluster)  [unwired: 11 in, 1 out]
            }
          }
          n765 = event shown="[0] \"Pane\": Mouse Move" {
            selector: _ -> [_ _ _]
            dyn-events: _ -> [_ _ _]
            timeout: _ -> [_ _ _]
            event Mouse Move {
              n766 = event-data() -> ("Coords"=w1118:T4)  [unwired: 1 in]
              n767 = local write "Real Coordinates"(w1118) -> ()
            }
            event Mouse Down {
              n768 = event-data() -> ("Coords"=w1119:T4)  [unwired: 1 in]
              n769 = local write "CoordinatesMousePressed"(w1119) -> ()
            }
            event "Pause Mouse/Mirror Connection": Value Change {
              n770 = event-data() -> ()  [unwired: 1 in, 3 out]
            }
          }
          n771 = local read "Stop"() -> (w1105:bool)
          n772 = Not(x="Pause Mouse/Mirror Connection") -> (.not. x?=w1106:bool)
          n773 = Or(x=w1106, y=w1105) -> (x .or. y?=w1108:bool)
        }
        n774 = call <vilib>:"DAQmx Clear Task.vi"("task in"=w1099, "error in"=w1098) -> ("error out"=w1100:errorcluster)  [unwired: 13 in]
        n775 = call <vilib>:"Simple Error Handler.vi"("error in (no error)"=w1100) -> ()  [unwired: 4 in, 5 out]
        n776 = call-poly <vilib>:"Close Input Device.vi"("error in (no error)"=w1096, "device ID"=w1095) -> ("error out"=w1097:errorcluster)  [unwired: 8 in]
        n777 = call <vilib>:"Simple Error Handler.vi"("error in (no error)"=w1097) -> ()  [unwired: 4 in, 5 out]
      }
    }
    n778 = node-c288() -> ()  [unwired: 1 in, 1 out]
  }
  n779 = node-c288(i64 100 ("Period")) -> (w89:T11)  [unwired: 3 in]
  n780 = timed-loop {
    tunnel: w91 -> [w1188]
    tunnel: [w1187] -> w90
    tunnel: w94 -> [w1190]
    tunnel: [w1189] -> w93
    timing: w89 -> [_]
    timing-out: [_] -> w88
    stop <- w1186 stop-if-true
    n781 = node-c288() -> ()  [unwired: 1 in, 1 out]
    n782 = event shown="[1] \"Shutter 2 (A)\": Value Change" {
      selector: _ -> [_ _ _]
      dyn-events: _ -> [_ _ _]
      timeout: _ -> [_ _ _]
      tunnel: w1190 -> [w1194 _ _]
      tunnel: [w1193 _ _] -> w1189
      tunnel: w1188 -> [_ w1214 _]
      tunnel: [_ w1212 _] -> w1187
      tunnel: [_ _ w1231] -> w1186
      event "Shutter 1 (B)": Value Change {
        n783 = event-data() -> ()  [unwired: 1 in, 1 out]
        n784 = flat-sequence {
          tunnel: [w1200] -> w1197
          tunnel: w1194 -> [w1199]
          tunnel: [w1204] -> w1196
          tunnel: [w1207] -> w1195
          tunnel: w1197 -> [w1202]
          tunnel: w1196 -> [w1211]
          tunnel: w1195 -> [w1209]
          tunnel: [w1208] -> w1193
          frame #0 {
            n785 = call-poly <vilib>:"DAQmx Write.vi"("task/channels in"=w1199, "data"=FALSE) -> ("task out"=w1200:refnum<k21>)  [unwired: 11 in, 2 out]
            n786 = Wait (ms)(milliseconds to wait=100) -> ()  [unwired: 1 out]
          }
          frame #1 {
            n787 = Or(x="Shutter 1 (B)", y=TRUE) -> (x .or. y?=w1204:bool)
            n788 = call-poly <vilib>:"DAQmx Write.vi"("task/channels in"=w1202, "data"=w1204) -> ("task out"=w1207:refnum<k21>)  [unwired: 11 in, 2 out]
            n789 = Wait (ms)(milliseconds to wait=100) -> ()  [unwired: 1 out]
          }
          frame #2 {
            n790 = Not(x=w1211) -> (.not. x?=w1210:bool)
            n791 = call-poly <vilib>:"DAQmx Write.vi"("task/channels in"=w1209, "data"=w1210) -> ("task out"=w1208:refnum<k21>)  [unwired: 11 in, 2 out]
          }
        }
      }
      event "Shutter 2 (A)": Value Change {
        n792 = event-data() -> ()  [unwired: 1 in, 1 out]
        n793 = flat-sequence {
          tunnel: w1214 -> [w1219]
          tunnel: [w1218] -> w1213
          tunnel: [w1223] -> w1216
          tunnel: [w1226] -> w1215
          tunnel: w1213 -> [w1221]
          tunnel: w1216 -> [w1230]
          tunnel: w1215 -> [w1228]
          tunnel: [w1227] -> w1212
          frame #0 {
            n794 = call-poly <vilib>:"DAQmx Write.vi"("task/channels in"=w1219, "data"=FALSE) -> ("task out"=w1218:refnum<k21>)  [unwired: 11 in, 2 out]
            n795 = Wait (ms)(milliseconds to wait=100) -> ()  [unwired: 1 out]
          }
          frame #1 {
            n796 = Or(x="Shutter 2 (A)", y=TRUE) -> (x .or. y?=w1223:bool)
            n797 = call-poly <vilib>:"DAQmx Write.vi"("task/channels in"=w1221, "data"=w1223) -> ("task out"=w1226:refnum<k21>)  [unwired: 11 in, 2 out]
            n798 = Wait (ms)(milliseconds to wait=100) -> ()  [unwired: 1 out]
          }
          frame #2 {
            n799 = Not(x=w1230) -> (.not. x?=w1229:bool)
            n800 = call-poly <vilib>:"DAQmx Write.vi"("task/channels in"=w1228, "data"=w1229) -> ("task out"=w1227:refnum<k21>)  [unwired: 11 in, 2 out]
          }
        }
      }
      event "Stop": Value Change {
        n801 = event-data() -> ("NewVal"=w1231:bool)  [unwired: 1 in, 5 out]
      }
    }
    n802 = node-c288() -> ()  [unwired: 1 in, 1 out]
  }
  n803 = node-c288(w88) -> ()  [unwired: 1 out]
  n804 = node-c288(w74) -> ()  [unwired: 1 out]
  n805 = call <vilib>:"DAQmx Clear Task.vi"("task in"=w90) -> ()  [unwired: 14 in, 1 out]
  n806 = call <vilib>:"DAQmx Clear Task.vi"("task in"=w93) -> ()  [unwired: 14 in, 1 out]
  n807 = node-c288(w26) -> ()  [unwired: 1 out]
  n808 = node-c288(w22) -> ()  [unwired: 1 out]
  n809 = local write "Tether"(FALSE ("Tether")) -> ()
  n810 = local read "Path"() -> (w81:path)
  n811 = node-c288(i64 1 ("Period"), 2 ("Processor")) -> (w87:T11)  [unwired: 2 in]
  n812 = VISA Close(VISA resource name=w19) -> (error out=w104:errorcluster)  [unwired: 1 in]
  n813 = timed-loop {
    timing: w87 -> [_]
    timing-out: [_] -> w86
    tunnel: w81 -> [w1233]
    stop <- w1232 stop-if-true
    n814 = node-c288() -> ()  [unwired: 1 in, 1 out]
    n815 = event shown="[7] \"Step size (nm)\", \"Scan speed (nm/s)\", \"# scans\", \"Pulling direction\", \"Scan range (nm)\": Value Change" {
      selector: _ -> [_ _ _ _ _ _ _ _ _]
      dyn-events: _ -> [_ _ _ _ _ _ _ _ _]
      timeout: _ -> [_ _ _ _ _ _ _ _ _]
      tunnel: w1233 -> [_ w1237 _ _ _ _ _ _ _]
      tunnel: [_ _ w1257 _ _ _ _ _ _] -> w1232
      event Timeout {
        n816 = event-data() -> ()  [unwired: 1 in, 2 out]
      }
      event "Read Cal": Value Change {
        n817 = event-data() -> ()  [unwired: 1 in, 6 out]
        n818 = Path To String(path=w1237) -> (string=w1236:string)
        n819 = Format Date/Time String(time format string (%c)="%y%m%d") -> (date/time string=w1238:string)  [unwired: 2 in]
        n820 = Concatenate Strings(w1236, "\\" ("string"), w1238, "\\" ("string"), "current.cal") -> (w1256:string)
        n821 = String To Path(string=w1256) -> (path=w1255:path)
        n822 = Open/Create/Replace File(file path (use dialog)=w1255, operation (0:open)=T8."open", access (0:read/write)=enum16{"read/write", "read-only", "write-only"}."read-only") -> (refnum out=w1251:refnum<file>, error out=w1252:errorcluster)  [unwired: 3 in, 1 out]
        n823 = Deny Access(4:w1252, 7:w1251) -> (0:w1250:errorcluster, 3:w1249:refnum<file>)  [unwired: 1 in]
        n824 = Read from Binary File(5:0.0, 8:w1250, 9:T9."big-endian, network order" ("byte order (0:big-endian, network order)"), 10:12 ("count"), 11:w1249) -> (0:w1245:errorcluster, 2:w1243:dbl[], 3:w1246:refnum<file>)  [unwired: 1 in, 1 out]
        n825 = Array To Cluster(array=w1243) -> (cluster=→"Cal values":T16)
        n826 = Close File(refnum=w1246, error in=w1245) -> ()  [unwired: 2 out]
        n827 = local write "Read Cal"(FALSE ("Read Cal")) -> ()
      }
      event "Stop": Value Change {
        n828 = event-data() -> ("NewVal"=w1257:bool)  [unwired: 1 in, 5 out]
      }
      event "Trap position (V)": Value Change {
        # "Need to rotate so X and Y don't get mixed up."
        n829 = event-data() -> ()  [unwired: 1 in, 6 out]
        n830 = local read "Mirror task"() -> (w1258:refnum<k21>)
        n831 = Cluster To Array(cluster="Trap position (V)") -> (array=w1261:dbl[])
        n832 = Rotate 1D Array(1:w1261, 2:1 ("n")) -> (0:w1259:dbl[])
        n833 = call-poly <vilib>:"DAQmx Write.vi"("task/channels in"=w1258, "data"=w1259) -> ("task out"=w1264:refnum<k21>, "error out"=w1263:errorcluster)  [unwired: 11 in, 1 out]
        n834 = call <vilib>:"DAQmx Stop Task.vi"("task/channels in"=w1264, "error in"=w1263) -> ("error out"=w1262:errorcluster)  [unwired: 12 in, 1 out]
        n835 = call <vilib>:"Simple Error Handler.vi"("error in (no error)"=w1262) -> ()  [unwired: 4 in, 5 out]
      }
      event "Trap delta (nm)": Value Change {
        n836 = event-data() -> ()  [unwired: 1 in, 6 out]
        n837 = local read "Pulling direction"() -> (w1266:bool)
        n838 = local read "Conv Y (nm/V)"() -> (w1267:dbl)
        n839 = local read "Conv X (nm/V)"() -> (w1268:dbl)
        n840 = Select(t=w1267, s=w1266, f=w1268) -> (s? t:f=w1269:dbl)
        n841 = local read "Fixed Y"() -> (w1275:dbl)
        n842 = Divide(x="Trap delta (nm)", y=w1269) -> (x/y=w1270:dbl)
        n843 = local read "Fixed X"() -> (w1274:dbl)
        n844 = Select(t=w1275, s=w1266, f=w1274) -> (s? t:f=w1273:dbl)
        n845 = Add(x=w1270, y=w1273) -> (x+y=w1271:dbl)
        n846 = case shown="False" w1266 {
          tunnel: w1271 -> [w1276 w1277]
          frame False {
            n847 = property on="X" class="DigNum (strict)"("Val(Sgnl)"=w1276) -> ()  [unwired: 2 in, 2 out]
          }
          frame True {
            n848 = property on="Y" class="DigNum (strict)"("Val(Sgnl)"=w1277) -> ()  [unwired: 2 in, 2 out]
          }
        }
      }
      event "Fish": Value Change {
        n849 = event-data() -> ()  [unwired: 1 in, 6 out]
        n850 = local read "Fish"() -> (w1278:bool)
        n851 = case shown="True" w1278 {
          frame False {
          }
          frame True {
            w1287 = 0.0 ("minimum value")
            w1288 = 10.0 ("maximum value")
            # "Grab offset in pulling\ndirection and add to \ndelta values"
            n852 = call-poly <vilib>:"DAQmx Create Virtual Channel.vi"("maximum value"=w1288, "minimum value"=w1287, "physical channels"=tag "Dev1/ao0") -> ("task out"=w1292:refnum<k21>, "error out"=w1291:errorcluster)  [unwired: 11 in]
            n853 = call-poly <vilib>:"DAQmx Create Virtual Channel.vi"("task in"=w1292, "maximum value"=w1288, "minimum value"=w1287, "physical channels"=tag "Dev1/ao1", "error in"=w1291) -> ("task out"=w1286:refnum<k21>, "error out"=w1285:errorcluster)  [unwired: 9 in]
            n854 = node-c288(i64 1 ("Period")) -> (w1294:T11)  [unwired: 3 in]
            n855 = timed-loop {
              timing: w1294 -> [_]
              timing-out: [_] -> w1293
              tunnel: w1286 -> [w1350]
              tunnel: w1285 -> [w1349]
              tunnel: [w1348] -> w1281
              tunnel: [w1347] -> w1280
              tunnel: [w1316] -> w1283
              tunnel: [w1329] -> w1279
              i -> [w1333]
              stop <- w1329 stop-if-true
              # "Send offset in direction\nof not-pulling to DAQ"
              n856 = node-c288() -> ()  [unwired: 1 in, 1 out]
              n857 = local read "Pulling direction"() -> (w1311:bool)
              n858 = local read "Conv Y (nm/V)"() -> (w1313:dbl)
              n859 = local read "Conv X (nm/V)"() -> (w1312:dbl)
              n860 = local read "Fixed X"() -> (w1320:dbl)
              n861 = local read "Fixed Y"() -> (w1319:dbl)
              n862 = Select(t=w1319, s=w1311, f=w1320) -> (s? t:f=w1321:dbl)
              n863 = Select(t=w1320, s=w1311, f=w1319) -> (s? t:f=w1318:dbl)
              n864 = Select(t=w1313, s=w1311, f=w1312) -> (s? t:f=w1308:dbl)
              n865 = Divide(x="Max fish\ndelta (nm)", y=w1308) -> (x/y=w1310:dbl)
              n866 = Divide(x="Min fish\ndelta (nm)", y=w1308) -> (x/y=w1309:dbl)
              n867 = Add(x=w1321, y=w1310) -> (x+y=w1323:dbl)
              n868 = Subtract(x=w1310, y=w1309) -> (x-y=w1325:dbl)
              n869 = Divide(x=w1325, y="Fish Speed (ms)") -> (x/y=w1326:dbl)
              n870 = flat-sequence {
                tunnel: w1311 -> [w1369]
                tunnel: w1318 -> [w1368]
                tunnel: w1350 -> [w1367]
                tunnel: w1349 -> [w1366]
                tunnel: w1326 -> [w1365]
                tunnel: w1323 -> [w1364]
                tunnel: "Fish Speed (ms)" -> [w1359]
                tunnel: [w1363] -> w1346
                tunnel: [w1362] -> w1345
                tunnel: [w1361] -> w1344
                tunnel: [w1360] -> w1343
                tunnel: [w1353] -> w1332
                tunnel: [w1352] -> w1317
                tunnel: [w1351] -> w1314
                tunnel: [w1416] -> w1342
                tunnel: w1346 -> [w1416]
                tunnel: [w1415] -> w1341
                tunnel: w1345 -> [w1415]
                tunnel: [w1414] -> w1340
                tunnel: w1344 -> [w1414]
                tunnel: [w1413] -> w1339
                tunnel: w1343 -> [w1413]
                tunnel: w1332 -> [w1412]
                tunnel: [w1412] -> w1331
                tunnel: w1317 -> [w1411]
                tunnel: [w1410] -> w1315
                tunnel: w1314 -> [w1410]
                tunnel: w1342 -> [w1427]
                tunnel: w1341 -> [w1426]
                tunnel: w1340 -> [w1425]
                tunnel: w1339 -> [w1424]
                tunnel: w1328 -> [w1423]
                tunnel: [w1422] -> w1348
                tunnel: [w1421] -> w1347
                tunnel: w1331 -> [w1420]
                tunnel: [w1419] -> w1316
                tunnel: w1315 -> [w1418]
                frame #0 {
                  n871 = local read "Mean force (pN)"() -> (w1358:dbl)
                  n872 = local read "Cutoff force (pN)"() -> (w1357:dbl)
                  n873 = Less Or Equal?(x=w1358, y=w1357) -> (x <= y?=w1355:bool)
                  n874 = And(x="Fish", y=w1355) -> (x .and. y?=w1356:bool)
                  n875 = case shown="True" w1356 {
                    selector: w1356 -> [w1371 _]
                    tunnel: w1369 -> [w1374 w1390]
                    tunnel: w1368 -> [_ w1389]
                    tunnel: w1367 -> [w1376 w1388]
                    tunnel: w1366 -> [w1375 w1387]
                    tunnel: w1365 -> [w1373 w1386]
                    tunnel: w1364 -> [w1372 w1385]
                    tunnel: [w1376 w1384] -> w1363
                    tunnel: [w1375 w1383] -> w1362
                    tunnel: [w1374 w1382] -> w1361
                    tunnel: [w1372 w1381] -> w1351
                    tunnel: [w1373 w1380] -> w1360
                    tunnel: w1359 -> [_ w1379]
                    tunnel: [w1371 w1378] -> w1353
                    tunnel: [FALSE w1377] -> w1352
                    frame False {
                    }
                    frame True {
                      n876 = while {
                        tunnel: w1390 -> [w1399]
                        tunnel: w1389 -> [w1398]
                        tunnel: w1388 -> [w1406]
                        tunnel: w1387 -> [w1405]
                        tunnel: w1386 -> [w1397]
                        tunnel: w1385 -> [w1403]
                        tunnel: [w1401] -> w1384
                        tunnel: [w1400] -> w1383
                        tunnel: [w1399] -> w1382
                        tunnel: [w1398] -> w1381
                        tunnel: [w1397] -> w1380
                        tunnel: w1379 -> [w1396]
                        tunnel: [w1391] -> w1378
                        tunnel: [w1391] -> w1377
                        i -> [w1395]
                        stop <- w1392 stop-if-true
                        n877 = Multiply(x=w1397, y=w1395) -> (x*y=w1404:dbl)
                        n878 = Subtract(x=w1403, y=w1404) -> (x-y=w1402:dbl)
                        n879 = Build Array(w1398, w1402) -> (w1409:dbl[])
                        n880 = Build Array(w1402, w1398) -> (w1408:dbl[])
                        n881 = Greater Or Equal?(x=w1395, y=w1396) -> (x >= y?=w1391:bool)
                        n882 = Select(t=w1409, s=w1399, f=w1408) -> (s? t:f=w1407:dbl[])
                        n883 = local read "Fish"() -> (w1393:bool)
                        n884 = Not(x=w1393) -> (.not. x?=w1394:bool)
                        n885 = call-poly <vilib>:"DAQmx Write.vi"("task/channels in"=w1406, "data"=w1407, "error in"=w1405) -> ("task out"=w1401:refnum<k21>, "error out"=w1400:errorcluster)  [unwired: 10 in, 1 out]
                        n886 = Compound Arithmetic op=OR(w1391, w1394) -> (w1392:bool)
                      }
                    }
                  }
                }
                frame #1 {
                  n887 = case shown="True" w1411 {
                    frame False {
                    }
                    frame True {
                      n888 = Wait (ms)(milliseconds to wait="Wait (ms)") -> ()  [unwired: 1 out]
                    }
                  }
                }
                frame #2 {
                  n889 = case shown="True" w1420 {
                    tunnel: w1427 -> [w1430 w1439]
                    tunnel: w1426 -> [w1429 w1438]
                    tunnel: w1425 -> [_ w1437]
                    tunnel: w1424 -> [_ w1436]
                    tunnel: w1423 -> [_ w1435]
                    tunnel: [w1430 w1434] -> w1422
                    tunnel: [w1429 w1433] -> w1421
                    tunnel: [FALSE w1432] -> w1419
                    tunnel: w1418 -> [_ w1431]
                    frame False {
                    }
                    frame True {
                      n890 = while {
                        tunnel: w1439 -> [w1471]
                        tunnel: w1438 -> [w1470]
                        tunnel: w1437 -> [w1442]
                        tunnel: w1436 -> [w1468]
                        tunnel: w1435 -> [w1467]
                        tunnel: [w1465] -> w1434
                        tunnel: [w1464] -> w1433
                        tunnel: [w1449] -> w1432
                        tunnel: w1431 -> [w1440]
                        i -> [w1456]
                        stop <- w1461 stop-if-true
                        # "If tether formed,\nimmediately change\nto new delta."
                        n891 = local read "Conv Y (nm/V)"() -> (w1443:dbl)
                        n892 = local read "Conv X (nm/V)"() -> (w1441:dbl)
                        n893 = local read "Fixed Y"() -> (w1450:dbl)
                        n894 = local read "Fixed X"() -> (w1455:dbl)
                        n895 = Select(t=w1443, s=w1442, f=w1441) -> (s? t:f=w1444:dbl)
                        n896 = local read "Cutoff force (pN)"() -> (w1457:dbl)
                        n897 = Divide(x="Delta after tether", y=w1444) -> (x/y=w1445:dbl)
                        n898 = Multiply(x=w1468, y=w1456) -> (x*y=w1469:dbl)
                        n899 = local read "Mean force (pN)"() -> (w1458:dbl)
                        n900 = Add(x=w1467, y=w1469) -> (x+y=w1452:dbl)
                        n901 = Select(t=w1450, s=w1442, f=w1455) -> (s? t:f=w1454:dbl)
                        n902 = Greater?(x=w1458, y=w1457) -> (0:w1449:bool)
                        n903 = Add(x=w1454, y=w1445) -> (x+y=w1453:dbl)
                        n904 = Select(t=w1453, s=w1449, f=w1452) -> (s? t:f=w1451:dbl)
                        n905 = local read "Fish Speed (ms)"() -> (w1463:i32)
                        n906 = Build Array(w1440, w1451) -> (w1466:dbl[])
                        n907 = Build Array(w1451, w1440) -> (w1447:dbl[])
                        n908 = Select(t=w1466, s=w1442, f=w1447) -> (s? t:f=w1446:dbl[])
                        n909 = case shown="True" w1449 {
                          tunnel: w1445 -> [_ _]
                          tunnel: w1446 -> [_ w1473]
                          frame False {
                          }
                          frame True {
                            n910 = Array To Cluster(array=w1473) -> (cluster=w1472:cluster{"[0]":dbl, "[1]":dbl})
                            n911 = local write "Trap position (V)"(w1472) -> ()
                          }
                        }
                        n912 = local read "Fish"() -> (w1460:bool)
                        n913 = Greater Or Equal?(x=w1456, y=w1463) -> (x >= y?=w1462:bool)
                        n914 = Not(x=w1460) -> (.not. x?=w1459:bool)
                        n915 = call-poly <vilib>:"DAQmx Write.vi"("task/channels in"=w1471, "data"=w1446, "error in"=w1470) -> ("task out"=w1465:refnum<k21>, "error out"=w1464:errorcluster)  [unwired: 10 in, 1 out]
                        n916 = Compound Arithmetic op=OR(w1462, w1459, w1449) -> (w1461:bool)
                      }
                    }
                  }
                }
              }
              n917 = Add(x=w1321, y=w1309) -> (x+y=w1328:dbl)
              n918 = Decrement(x="# attempts") -> (x-1=w1337:dbl)
              n919 = Greater Or Equal?(x=w1333, y=w1337) -> (x >= y?=w1336:bool)
              n920 = local read "Mean force (pN)"() -> (w1335:dbl)
              n921 = Greater?(x=w1335, y="Cutoff force (pN)") -> (0:w1330:bool)
              n922 = Compound Arithmetic op=OR(w1316, w1330, w1336) -> (w1329:bool)
              n923 = case shown="True" w1316 {
                frame False {
                }
                frame True {
                  n924 = call <vilib>:"Beep.vi"() -> ()  [unwired: 12 in]
                }
              }
              n925 = node-c288() -> ()  [unwired: 1 in, 1 out]
              "Tether" <- w1316
              "Attempt #" <- w1333
            }
            n926 = node-c288(w1293) -> ()  [unwired: 1 out]
            n927 = flat-sequence {
              tunnel: w1283 -> [w1302]
              tunnel: [w1302] -> w1282
              tunnel: w1281 -> [w1299]
              tunnel: w1280 -> [w1298]
              tunnel: w1279 -> [w1297]
              tunnel: w1282 -> [w1304]
              frame #0 {
                w1301 = T14 1 items=["no dialog", "OK message", "continue or stop message", "OK message + warnings", "continue/stop + warnings"] ("type of dialog (OK msg:1)")
                n928 = call <vilib>:"DAQmx Clear Task.vi"("task in"=w1299, "error in"=w1298) -> ("error out"=w1300:errorcluster)  [unwired: 13 in]
                n929 = Not(x=w1297) -> (.not. x?=w1296:bool)
                n930 = local write "Fish"(w1296) -> ()
                n931 = Wait (ms)(milliseconds to wait=u32 300) -> ()  [unwired: 1 out]
                n932 = call <vilib>:"Simple Error Handler.vi"("type of dialog (OK msg:1)"=w1301, "error in (no error)"=w1300) -> ()  [unwired: 3 in, 5 out]
              }
              frame #1 {
                n933 = And(x=w1304, y="Raster after\n tether?") -> (x .and. y?=w1305:bool)
                n934 = case shown="True" w1305 {
                  selector: w1305 -> [_ w1307]
                  frame False {
                  }
                  frame True {
                    n935 = property on="Raster scan" class="Bool (strict)"("Val(Sgnl)"=w1307) -> ()  [unwired: 2 in, 2 out]
                    n936 = property on="Inject Sample" class="Bool (strict)"("Val(Sgnl)"=FALSE ("Value (Signaling)")) -> ()  [unwired: 2 in, 2 out]
                  }
                }
              }
            }
          }
        }
      }
      event "Load param": Value Change {
        n937 = event-data() -> ()  [unwired: 1 in, 6 out]
        n938 = property on="Scan Parameters" class="Arr (strict)"() -> ("Index Values"=w1486:u32[])  [unwired: 2 in, 2 out]
        n939 = Index Array(array=w1486, index=0) -> (element=w1483:u32)
        n940 = Index Array(array="Scan Parameters", index=w1483) -> (element=w1482:T17)
        n941 = Unbundle "Unbundle"(w1482) -> ("# scans 2"=w1481:i32)  [unwired: 4 out]
        n942 = local write "Load param"(FALSE ("Load param")) -> ()
        n943 = property on="# scans" class="DigNum (strict)"("Val(Sgnl)"=w1481) -> ()  [unwired: 2 in, 2 out]
      }
      event "Step size (nm)", "Scan speed (nm/s)", "# scans", "Pulling direction", "Scan range (nm)": Value Change {
        n944 = event-data() -> ()  [unwired: 1 in, 6 out]
        n945 = local read "Pulling direction"() -> (w1517:bool)
        n946 = Reciprocal(x="Scan speed (nm/s)") -> (1/x=w1509:dbl)
        n947 = local read "Conv Y (nm/V)"() -> (w1515:dbl)
        n948 = local read "Conv X (nm/V)"() -> (w1516:dbl)
        n949 = Multiply(x="Step size (nm)", y=w1509) -> (x*y=w1507:dbl)
        n950 = Divide(x="Scan range (nm)", y="Step size (nm)") -> (x/y=w1514:dbl)
        n951 = Absolute Value(x=w1514) -> (abs(x)=w1513:dbl)
        n952 = Multiply(x=w1507, y=1000.0) -> (x*y=w1494:dbl)
        n953 = Select(t=w1515, s=w1517, f=w1516) -> (s? t:f=w1505:dbl)
        n954 = Multiply(x="# scans", y=2) -> (x*y=w1493:i32)
        n955 = To Unsigned Quad Integer(1:w1513) -> (0:w1503:u64)
        "Scan steps (mirror)" <- w1503
        n956 = Divide(x="Scan range (nm)", y=w1505) -> (x/y=→"Scan range (V)":dbl)
        n957 = Multiply(x=w1503, y=w1494) -> (x*y=w1502:dbl)
        n958 = Divide(x="Step size (nm)", y=w1505) -> (x/y=→"Scan increment (V)":dbl)
        n959 = Round Toward +Infinity(x=w1494) -> (ceil(x): smallest int >= x=w1491:dbl)
        "Time per step (ms)" <- w1491
        n960 = local read "Data update period (s/set)"() -> (w1497:dbl)
        n961 = Multiply(x=w1493, y=w1502) -> (x*y=w1500:dbl)
        n962 = Divide(x=w1500, y=1000.0) -> (x/y=w1498:dbl)
        "Total raster time (s)" <- w1498
        n963 = local read "Data update period (s/set)"() -> (w1489:dbl)
        n964 = Divide(x=w1498, y=w1497) -> (x/y=w1496:dbl)
        n965 = Round Toward -Infinity(1:w1496) -> (0:→"N sets to be saved":dbl)
        n966 = Multiply(x=w1489, y=1000.0) -> (x*y=w1487:dbl)
        n967 = Less?(x=w1491, y=w1487) -> (x < y?=w1490:bool)
        n968 = case shown="True" w1490 {
          selector: w1490 -> [_ w1518]
          frame False {
          }
          frame True {
            n969 = call "Display Message to User"("Enable"=w1518) -> ()  [unwired: 9 in, 2 out]
          }
        }
      }
      event "Averaging Number": Value Change {
        n970 = event-data() -> ()  [unwired: 1 in, 6 out]
        n971 = local read "# Samples/channel (in)"() -> (w1522:i32)
        n972 = local read "Averaging Number"() -> (w1520:i32)
        n973 = Quotient & Remainder(x=w1522, y=w1520) -> (floor(x/y)=w1521:i32)  [unwired: 1 out]
        n974 = Multiply(x=w1521, y=w1520) -> (x*y=w1519:i32)
        n975 = local write "# Samples/channel (in)"(w1519) -> ()
      }
    }
    n976 = node-c288() -> ()  [unwired: 1 in, 1 out]
  }
  n977 = call <vilib>:"Simple Error Handler.vi"("error in (no error)"=w104) -> ()  [unwired: 4 in, 5 out]
  n978 = disable-structure shown="Enabled" {
    frame Disabled {
      n979 = node-c288(2 ("Processor")) -> (w1528:T11)  [unwired: 3 in]
      n980 = timed-loop "Pump Control" {
        timing: w1528 -> [_]
        timing-out: [_] -> w1527
        tunnel: refnum<visa-resource-name> "COM6" ("VISA resource name") -> [w1530]
        stop <- w1529 stop-if-true
        n981 = node-c288() -> ()  [unwired: 1 in, 1 out]
        n982 = event shown="[4] \"Inject Pump 1\": Value Change" {
          selector: _ -> [_ _ _ _ _ _ _ _ _]
          dyn-events: _ -> [_ _ _ _ _ _ _ _ _]
          timeout: _ -> [_ _ _ _ _ _ _ _ _]
          tunnel: w1530 -> [w1538 w1634 _ w1710 w1838 w1981 w2026 w2084 w2143]
          tunnel: [_ _ w1709 _ _ _ _ _ _] -> w1529
          event "Flush Pump 1": Value Change {
            w1539 = "\r"
            n983 = event-data() -> ()  [unwired: 1 in, 5 out]
            n984 = call-poly "VISA Configure Serial Port"("VISA resource name"=w1538) -> ("VISA resource name out"=w1552:refnum<visa-resource-name>, "error out"=w1553:errorcluster)  [unwired: 13 in]
            n985 = local read "Write Wait"() -> (w1531:i32)
            n986 = Concatenate Strings("enter pump1", w1539) -> (w1540:string)
            n987 = flat-sequence {
              tunnel: w1553 -> [w1572]
              tunnel: w1552 -> [w1574]
              tunnel: [w1573] -> w1569
              tunnel: [w1571] -> w1568
              tunnel: w1540 -> [w1570]
              tunnel: w1569 -> [w1577]
              tunnel: [w1577] -> w1567
              tunnel: w1568 -> [w1576]
              tunnel: [w1576] -> w1566
              tunnel: w1531 -> [w1575]
              tunnel: [w1582] -> w1565
              tunnel: w1545 -> [w1581]
              tunnel: [w1578] -> w1564
              tunnel: w1567 -> [w1580]
              tunnel: w1566 -> [w1579]
              tunnel: w1565 -> [w1585]
              tunnel: [w1585] -> w1563
              tunnel: [w1584] -> w1562
              tunnel: w1564 -> [w1584]
              tunnel: w1531 -> [w1583]
              tunnel: w1563 -> [w1590]
              tunnel: [w1589] -> w1561
              tunnel: w1548 -> [w1588]
              tunnel: w1562 -> [w1587]
              tunnel: [w1586] -> w1560
              tunnel: w1561 -> [w1593]
              tunnel: [w1593] -> w1559
              tunnel: [w1592] -> w1558
              tunnel: w1560 -> [w1592]
              tunnel: w1531 -> [w1591]
              tunnel: w1559 -> [w1598]
              tunnel: [w1597] -> w1557
              tunnel: w1551 -> [w1596]
              tunnel: w1558 -> [w1595]
              tunnel: [w1594] -> w1556
              tunnel: [w1601] -> w1555
              tunnel: w1557 -> [w1601]
              tunnel: [w1600] -> w1554
              tunnel: w1556 -> [w1600]
              tunnel: w1531 -> [w1599]
              tunnel: w1555 -> [w1606]
              tunnel: w1554 -> [w1603]
              tunnel: [w1605] -> w1534
              tunnel: [w1604] -> w1532
              tunnel: [w1611] -> w1535
              tunnel: w1534 -> [w1611]
              tunnel: [w1610] -> w1533
              tunnel: w1532 -> [w1610]
              tunnel: w1531 -> [w1609]
              tunnel: w1535 -> [w1613]
              tunnel: w1533 -> [w1612]
              frame #0 {
                n988 = VISA Write(VISA resource name=w1574, write buffer=w1570, error in (no error)=w1572) -> (VISA resource name out=w1573:refnum<visa-resource-name>, error out=w1571:errorcluster)  [unwired: 1 out]
              }
              frame #1 {
                n989 = Wait (ms)(milliseconds to wait=w1575) -> ()  [unwired: 1 out]
              }
              frame #2 {
                n990 = VISA Write(VISA resource name=w1580, write buffer=w1581, error in (no error)=w1579) -> (VISA resource name out=w1582:refnum<visa-resource-name>, error out=w1578:errorcluster)  [unwired: 1 out]
              }
              frame #3 {
                n991 = Wait (ms)(milliseconds to wait=w1583) -> ()  [unwired: 1 out]
              }
              frame #4 {
                n992 = VISA Write(VISA resource name=w1590, write buffer=w1588, error in (no error)=w1587) -> (VISA resource name out=w1589:refnum<visa-resource-name>, error out=w1586:errorcluster)  [unwired: 1 out]
              }
              frame #5 {
                n993 = Wait (ms)(milliseconds to wait=w1591) -> ()  [unwired: 1 out]
              }
              frame #6 {
                n994 = VISA Write(VISA resource name=w1598, write buffer=w1596, error in (no error)=w1595) -> (VISA resource name out=w1597:refnum<visa-resource-name>, error out=w1594:errorcluster)  [unwired: 1 out]
              }
              frame #7 {
                n995 = Wait (ms)(milliseconds to wait=w1599) -> ()  [unwired: 1 out]
              }
              frame #8 {
                n996 = Concatenate Strings("start ", "\r") -> (w1602:string)
                n997 = VISA Write(VISA resource name=w1606, write buffer=w1602, error in (no error)=w1603) -> (VISA resource name out=w1605:refnum<visa-resource-name>, error out=w1604:errorcluster)  [unwired: 1 out]
              }
              frame #9 {
                n998 = Wait (ms)(milliseconds to wait=w1609) -> ()  [unwired: 1 out]
              }
              frame #10 {
                n999 = local write "Flush Pump 1"(FALSE ("Flush Pump 1")) -> ()
                n1000 = Concatenate Strings("enter main ", "\r") -> (w1617:string)
                n1001 = VISA Write(VISA resource name=w1613, write buffer=w1617, error in (no error)=w1612) -> (VISA resource name out=w1616:refnum<visa-resource-name>, error out=w1615:errorcluster)  [unwired: 1 out]
                n1002 = VISA Close(VISA resource name=w1616, error in (no error)=w1615) -> ()  [unwired: 1 out]
              }
            }
            n1003 = Concatenate Strings("set units 4 ", w1539) -> (w1545:string)
            n1004 = Multiply(x="Flush\nRate (ul/min)", y=60) -> (x*y=w1543:dbl)
            n1005 = Number To Decimal String(number=w1543) -> (decimal integer string=w1546:string)  [unwired: 1 in]
            n1006 = Concatenate Strings("set rate ", w1546, w1539) -> (w1548:string)
            n1007 = Number To Decimal String(number="Flush\nVolume (ul)") -> (decimal integer string=w1550:string)  [unwired: 1 in]
            n1008 = Concatenate Strings("set volume ", w1550, w1539) -> (w1551:string)
          }
          event "Flush Pump 2": Value Change {
            w1625 = "\r"
            n1009 = event-data() -> ()  [unwired: 1 in, 5 out]
            n1010 = call-poly "VISA Configure Serial Port"("VISA resource name"=w1634) -> ("VISA resource name out"=w1645:refnum<visa-resource-name>, "error out"=w1646:errorcluster)  [unwired: 13 in]
            n1011 = local read "Write Wait"() -> (w1620:i32)
            n1012 = Concatenate Strings("enter pump2", w1625) -> (w1626:string)
            n1013 = flat-sequence {
              tunnel: w1646 -> [w1661]
              tunnel: w1645 -> [w1663]
              tunnel: [w1662] -> w1631
              tunnel: [w1660] -> w1629
              tunnel: w1626 -> [w1659]
              tunnel: w1631 -> [w1666]
              tunnel: [w1666] -> w1630
              tunnel: w1629 -> [w1665]
              tunnel: [w1665] -> w1628
              tunnel: w1620 -> [w1664]
              tunnel: [w1671] -> w1658
              tunnel: w1638 -> [w1670]
              tunnel: [w1667] -> w1657
              tunnel: w1630 -> [w1669]
              tunnel: w1628 -> [w1668]
              tunnel: w1658 -> [w1674]
              tunnel: [w1674] -> w1656
              tunnel: [w1673] -> w1655
              tunnel: w1657 -> [w1673]
              tunnel: w1620 -> [w1672]
              tunnel: w1656 -> [w1679]
              tunnel: [w1678] -> w1654
              tunnel: w1641 -> [w1677]
              tunnel: w1655 -> [w1676]
              tunnel: [w1675] -> w1653
              tunnel: w1654 -> [w1682]
              tunnel: [w1682] -> w1652
              tunnel: [w1681] -> w1651
              tunnel: w1653 -> [w1681]
              tunnel: w1620 -> [w1680]
              tunnel: w1652 -> [w1687]
              tunnel: [w1686] -> w1650
              tunnel: w1644 -> [w1685]
              tunnel: w1651 -> [w1684]
              tunnel: [w1683] -> w1649
              tunnel: [w1690] -> w1648
              tunnel: w1650 -> [w1690]
              tunnel: [w1689] -> w1647
              tunnel: w1649 -> [w1689]
              tunnel: w1620 -> [w1688]
              tunnel: w1648 -> [w1697]
              tunnel: w1647 -> [w1696]
              tunnel: [w1692] -> w1624
              tunnel: [w1691] -> w1622
              tunnel: w1624 -> [w1700]
              tunnel: [w1700] -> w1623
              tunnel: w1622 -> [w1699]
              tunnel: [w1699] -> w1621
              tunnel: w1620 -> [w1698]
              tunnel: w1623 -> [w1704]
              tunnel: w1621 -> [w1703]
              frame #0 {
                n1014 = VISA Write(VISA resource name=w1663, write buffer=w1659, error in (no error)=w1661) -> (VISA resource name out=w1662:refnum<visa-resource-name>, error out=w1660:errorcluster)  [unwired: 1 out]
              }
              frame #1 {
                n1015 = Wait (ms)(milliseconds to wait=w1664) -> ()  [unwired: 1 out]
              }
              frame #2 {
                n1016 = VISA Write(VISA resource name=w1669, write buffer=w1670, error in (no error)=w1668) -> (VISA resource name out=w1671:refnum<visa-resource-name>, error out=w1667:errorcluster)  [unwired: 1 out]
              }
              frame #3 {
                n1017 = Wait (ms)(milliseconds to wait=w1672) -> ()  [unwired: 1 out]
              }
              frame #4 {
                n1018 = VISA Write(VISA resource name=w1679, write buffer=w1677, error in (no error)=w1676) -> (VISA resource name out=w1678:refnum<visa-resource-name>, error out=w1675:errorcluster)  [unwired: 1 out]
              }
              frame #5 {
                n1019 = Wait (ms)(milliseconds to wait=w1680) -> ()  [unwired: 1 out]
              }
              frame #6 {
                n1020 = VISA Write(VISA resource name=w1687, write buffer=w1685, error in (no error)=w1684) -> (VISA resource name out=w1686:refnum<visa-resource-name>, error out=w1683:errorcluster)  [unwired: 1 out]
              }
              frame #7 {
                n1021 = Wait (ms)(milliseconds to wait=w1688) -> ()  [unwired: 1 out]
              }
              frame #8 {
                n1022 = Concatenate Strings("start ", "\r") -> (w1695:string)
                n1023 = VISA Write(VISA resource name=w1697, write buffer=w1695, error in (no error)=w1696) -> (VISA resource name out=w1692:refnum<visa-resource-name>, error out=w1691:errorcluster)  [unwired: 1 out]
              }
              frame #9 {
                n1024 = Wait (ms)(milliseconds to wait=w1698) -> ()  [unwired: 1 out]
              }
              frame #10 {
                n1025 = local write "Flush Pump 2"(FALSE ("Flush Pump 1")) -> ()
                n1026 = Concatenate Strings("enter main ", "\r") -> (w1705:string)
                n1027 = VISA Write(VISA resource name=w1704, write buffer=w1705, error in (no error)=w1703) -> (VISA resource name out=w1702:refnum<visa-resource-name>, error out=w1701:errorcluster)  [unwired: 1 out]
                n1028 = VISA Close(VISA resource name=w1702, error in (no error)=w1701) -> ()  [unwired: 1 out]
              }
            }
            n1029 = Concatenate Strings("set units 4 ", w1625) -> (w1638:string)
            n1030 = Multiply(x="Flush \nRate (ul/min)  2", y=60) -> (x*y=w1636:dbl)
            n1031 = Number To Decimal String(number=w1636) -> (decimal integer string=w1639:string)  [unwired: 1 in]
            n1032 = Concatenate Strings("set rate ", w1639, w1625) -> (w1641:string)
            n1033 = Number To Decimal String(number="Flush\nVolume (ul)  2") -> (decimal integer string=w1643:string)  [unwired: 1 in]
            n1034 = Concatenate Strings("set volume ", w1643, w1625) -> (w1644:string)
          }
          event "Stop": Value Change {
            n1035 = event-data() -> ()  [unwired: 1 in, 5 out]
            n1036 = local read "Stop"() -> (w1709:bool)
          }
          event "Inject Pump 2": Value Change {
            n1037 = event-data() -> ()  [unwired: 1 in, 5 out]
            n1038 = case shown="True" "Inject Pump 2" {
              tunnel: w1710 -> [w1713 w1755]
              frame False {
                n1039 = local read "Write Wait"() -> (w1712:i32)
                n1040 = call-poly "VISA Configure Serial Port"("VISA resource name"=w1713) -> ("VISA resource name out"=w1717:refnum<visa-resource-name>, "error out"=w1718:errorcluster)  [unwired: 13 in]
                n1041 = Concatenate Strings("enter pump2", "\r") -> (w1715:string)
                n1042 = flat-sequence {
                  tunnel: w1718 -> [w1729]
                  tunnel: w1717 -> [w1731]
                  tunnel: [w1730] -> w1726
                  tunnel: [w1728] -> w1725
                  tunnel: w1715 -> [w1727]
                  tunnel: w1726 -> [w1734]
                  tunnel: w1725 -> [w1733]
                  tunnel: [w1734] -> w1724
                  tunnel: [w1733] -> w1723
                  tunnel: w1712 -> [w1732]
                  tunnel: [w1738] -> w1722
                  tunnel: [w1737] -> w1721
                  tunnel: w1724 -> [w1736]
                  tunnel: w1723 -> [w1735]
                  tunnel: w1722 -> [w1744]
                  tunnel: [w1744] -> w1720
                  tunnel: w1721 -> [w1743]
                  tunnel: [w1743] -> w1719
                  tunnel: w1712 -> [w1742]
                  tunnel: w1720 -> [w1748]
                  tunnel: w1719 -> [w1747]
                  frame #0 {
                    n1043 = VISA Write(VISA resource name=w1731, write buffer=w1727, error in (no error)=w1729) -> (VISA resource name out=w1730:refnum<visa-resource-name>, error out=w1728:errorcluster)  [unwired: 1 out]
                  }
                  frame #1 {
                    n1044 = Wait (ms)(milliseconds to wait=w1732) -> ()  [unwired: 1 out]
                  }
                  frame #2 {
                    n1045 = Concatenate Strings("stop ", "\r") -> (w1741:string)
                    n1046 = VISA Write(VISA resource name=w1736, write buffer=w1741, error in (no error)=w1735) -> (VISA resource name out=w1738:refnum<visa-resource-name>, error out=w1737:errorcluster)  [unwired: 1 out]
                  }
                  frame #3 {
                    n1047 = Wait (ms)(milliseconds to wait=w1742) -> ()  [unwired: 1 out]
                  }
                  frame #4 {
                    n1048 = Concatenate Strings("enter main ", "\r") -> (w1749:string)
                    n1049 = VISA Write(VISA resource name=w1748, write buffer=w1749, error in (no error)=w1747) -> (VISA resource name out=w1746:refnum<visa-resource-name>, error out=w1745:errorcluster)  [unwired: 1 out]
                    n1050 = VISA Close(VISA resource name=w1746, error in (no error)=w1745) -> ()  [unwired: 1 out]
                  }
                }
              }
              frame True {
                w1768 = "\r"
                n1051 = call-poly "VISA Configure Serial Port"("VISA resource name"=w1755) -> ("VISA resource name out"=w1757:refnum<visa-resource-name>, "error out"=w1756:errorcluster)  [unwired: 13 in]
                n1052 = local read "Write Wait"() -> (w1752:i32)
                n1053 = Concatenate Strings("enter pump2", w1768) -> (w1767:string)
                n1054 = flat-sequence {
                  tunnel: w1756 -> [w1791]
                  tunnel: w1757 -> [w1793]
                  tunnel: [w1792] -> w1788
                  tunnel: [w1790] -> w1787
                  tunnel: w1767 -> [w1789]
                  tunnel: w1788 -> [w1796]
                  tunnel: [w1796] -> w1786
                  tunnel: w1787 -> [w1795]
                  tunnel: [w1795] -> w1785
                  tunnel: w1752 -> [w1794]
                  tunnel: [w1801] -> w1784
                  tunnel: w1764 -> [w1800]
                  tunnel: [w1797] -> w1783
                  tunnel: w1786 -> [w1799]
                  tunnel: w1785 -> [w1798]
                  tunnel: w1784 -> [w1804]
                  tunnel: [w1804] -> w1782
                  tunnel: [w1803] -> w1781
                  tunnel: w1783 -> [w1803]
                  tunnel: w1752 -> [w1802]
                  tunnel: w1782 -> [w1809]
                  tunnel: [w1808] -> w1780
                  tunnel: w1761 -> [w1807]
                  tunnel: w1781 -> [w1806]
                  tunnel: [w1805] -> w1779
                  tunnel: w1780 -> [w1812]
                  tunnel: [w1812] -> w1778
                  tunnel: [w1811] -> w1777
                  tunnel: w1779 -> [w1811]
                  tunnel: w1752 -> [w1810]
                  tunnel: w1778 -> [w1817]
                  tunnel: [w1816] -> w1776
                  tunnel: w1758 -> [w1815]
                  tunnel: w1777 -> [w1814]
                  tunnel: [w1813] -> w1775
                  tunnel: [w1820] -> w1774
                  tunnel: w1776 -> [w1820]
                  tunnel: [w1819] -> w1773
                  tunnel: w1775 -> [w1819]
                  tunnel: w1752 -> [w1818]
                  tunnel: w1774 -> [w1827]
                  tunnel: w1773 -> [w1826]
                  tunnel: [w1822] -> w1772
                  tunnel: [w1821] -> w1771
                  tunnel: w1772 -> [w1830]
                  tunnel: [w1830] -> w1770
                  tunnel: w1771 -> [w1829]
                  tunnel: [w1829] -> w1769
                  tunnel: w1752 -> [w1828]
                  tunnel: w1770 -> [w1834]
                  tunnel: w1769 -> [w1833]
                  frame #0 {
                    n1055 = VISA Write(VISA resource name=w1793, write buffer=w1789, error in (no error)=w1791) -> (VISA resource name out=w1792:refnum<visa-resource-name>, error out=w1790:errorcluster)  [unwired: 1 out]
                  }
                  frame #1 {
                    n1056 = Wait (ms)(milliseconds to wait=w1794) -> ()  [unwired: 1 out]
                  }
                  frame #2 {
                    n1057 = VISA Write(VISA resource name=w1799, write buffer=w1800, error in (no error)=w1798) -> (VISA resource name out=w1801:refnum<visa-resource-name>, error out=w1797:errorcluster)  [unwired: 1 out]
                  }
                  frame #3 {
                    n1058 = Wait (ms)(milliseconds to wait=w1802) -> ()  [unwired: 1 out]
                  }
                  frame #4 {
                    n1059 = VISA Write(VISA resource name=w1809, write buffer=w1807, error in (no error)=w1806) -> (VISA resource name out=w1808:refnum<visa-resource-name>, error out=w1805:errorcluster)  [unwired: 1 out]
                  }
                  frame #5 {
                    n1060 = Wait (ms)(milliseconds to wait=w1810) -> ()  [unwired: 1 out]
                  }
                  frame #6 {
                    n1061 = VISA Write(VISA resource name=w1817, write buffer=w1815, error in (no error)=w1814) -> (VISA resource name out=w1816:refnum<visa-resource-name>, error out=w1813:errorcluster)  [unwired: 1 out]
                  }
                  frame #7 {
                    n1062 = Wait (ms)(milliseconds to wait=w1818) -> ()  [unwired: 1 out]
                  }
                  frame #8 {
                    n1063 = Concatenate Strings("start ", "\r") -> (w1825:string)
                    n1064 = VISA Write(VISA resource name=w1827, write buffer=w1825, error in (no error)=w1826) -> (VISA resource name out=w1822:refnum<visa-resource-name>, error out=w1821:errorcluster)  [unwired: 1 out]
                  }
                  frame #9 {
                    n1065 = Wait (ms)(milliseconds to wait=w1828) -> ()  [unwired: 1 out]
                  }
                  frame #10 {
                    n1066 = Concatenate Strings("enter main ", "\r") -> (w1835:string)
                    n1067 = VISA Write(VISA resource name=w1834, write buffer=w1835, error in (no error)=w1833) -> (VISA resource name out=w1832:refnum<visa-resource-name>, error out=w1831:errorcluster)  [unwired: 1 out]
                    n1068 = VISA Close(VISA resource name=w1832, error in (no error)=w1831) -> ()  [unwired: 1 out]
                  }
                }
                n1069 = local read "Normal \nRate (ul/hr)  2"() -> (w1753:dbl)
                n1070 = Concatenate Strings("set units 4 ", w1768) -> (w1764:string)
                n1071 = local read "Normal \nVolume (ul) 2"() -> (w1754:dbl)
                n1072 = Number To Decimal String(number=w1753) -> (decimal integer string=w1763:string)  [unwired: 1 in]
                n1073 = Concatenate Strings("set rate ", w1763, w1768) -> (w1761:string)
                n1074 = Number To Decimal String(number=w1754) -> (decimal integer string=w1759:string)  [unwired: 1 in]
                n1075 = Concatenate Strings("set volume ", w1759, w1768) -> (w1758:string)
              }
            }
          }
          event "Inject Pump 1": Value Change {
            n1076 = event-data() -> ()  [unwired: 1 in, 5 out]
            n1077 = case shown="True" "Inject Pump 1" {
              tunnel: w1838 -> [w1841 w1883]
              frame False {
                n1078 = local read "Write Wait"() -> (w1840:i32)
                n1079 = call-poly "VISA Configure Serial Port"("VISA resource name"=w1841) -> ("VISA resource name out"=w1845:refnum<visa-resource-name>, "error out"=w1846:errorcluster)  [unwired: 13 in]
                n1080 = Concatenate Strings("enter pump1", "\r") -> (w1843:string)
                n1081 = flat-sequence {
                  tunnel: w1846 -> [w1857]
                  tunnel: w1845 -> [w1859]
                  tunnel: [w1858] -> w1854
                  tunnel: [w1856] -> w1853
                  tunnel: w1843 -> [w1855]
                  tunnel: w1854 -> [w1862]
                  tunnel: w1853 -> [w1861]
                  tunnel: [w1862] -> w1852
                  tunnel: [w1861] -> w1851
                  tunnel: w1840 -> [w1860]
                  tunnel: [w1866] -> w1850
                  tunnel: [w1865] -> w1849
                  tunnel: w1852 -> [w1864]
                  tunnel: w1851 -> [w1863]
                  tunnel: w1850 -> [w1872]
                  tunnel: [w1872] -> w1848
                  tunnel: w1849 -> [w1871]
                  tunnel: [w1871] -> w1847
                  tunnel: w1840 -> [w1870]
                  tunnel: w1848 -> [w1876]
                  tunnel: w1847 -> [w1875]
                  frame #0 {
                    n1082 = VISA Write(VISA resource name=w1859, write buffer=w1855, error in (no error)=w1857) -> (VISA resource name out=w1858:refnum<visa-resource-name>, error out=w1856:errorcluster)  [unwired: 1 out]
                  }
                  frame #1 {
                    n1083 = Wait (ms)(milliseconds to wait=w1860) -> ()  [unwired: 1 out]
                  }
                  frame #2 {
                    n1084 = Concatenate Strings("stop ", "\r") -> (w1869:string)
                    n1085 = VISA Write(VISA resource name=w1864, write buffer=w1869, error in (no error)=w1863) -> (VISA resource name out=w1866:refnum<visa-resource-name>, error out=w1865:errorcluster)  [unwired: 1 out]
                  }
                  frame #3 {
                    n1086 = Wait (ms)(milliseconds to wait=w1870) -> ()  [unwired: 1 out]
                  }
                  frame #4 {
                    n1087 = Concatenate Strings("enter main ", "\r") -> (w1877:string)
                    n1088 = VISA Write(VISA resource name=w1876, write buffer=w1877, error in (no error)=w1875) -> (VISA resource name out=w1874:refnum<visa-resource-name>, error out=w1873:errorcluster)  [unwired: 1 out]
                    n1089 = VISA Close(VISA resource name=w1874, error in (no error)=w1873) -> ()  [unwired: 1 out]
                  }
                }
              }
              frame True {
                w1896 = "\r"
                n1090 = call-poly "VISA Configure Serial Port"("VISA resource name"=w1883) -> ("VISA resource name out"=w1885:refnum<visa-resource-name>, "error out"=w1884:errorcluster)  [unwired: 13 in]
                n1091 = local read "Write Wait"() -> (w1880:i32)
                n1092 = flat-sequence {
                  tunnel: w1884 -> [w1919]
                  tunnel: w1885 -> [w1921]
                  tunnel: [w1920] -> w1916
                  tunnel: [w1918] -> w1915
                  tunnel: w1895 -> [w1917]
                  tunnel: w1916 -> [w1924]
                  tunnel: [w1924] -> w1914
                  tunnel: w1915 -> [w1923]
                  tunnel: [w1923] -> w1913
                  tunnel: w1880 -> [w1922]
                  tunnel: [w1929] -> w1912
                  tunnel: w1892 -> [w1928]
                  tunnel: [w1925] -> w1911
                  tunnel: w1914 -> [w1927]
                  tunnel: w1913 -> [w1926]
                  tunnel: w1912 -> [w1932]
                  tunnel: [w1932] -> w1910
                  tunnel: [w1931] -> w1909
                  tunnel: w1911 -> [w1931]
                  tunnel: w1880 -> [w1930]
                  tunnel: w1910 -> [w1937]
                  tunnel: [w1936] -> w1908
                  tunnel: w1889 -> [w1935]
                  tunnel: w1909 -> [w1934]
                  tunnel: [w1933] -> w1907
                  tunnel: w1908 -> [w1940]
                  tunnel: [w1940] -> w1906
                  tunnel: [w1939] -> w1905
                  tunnel: w1907 -> [w1939]
                  tunnel: w1880 -> [w1938]
                  tunnel: w1906 -> [w1945]
                  tunnel: [w1944] -> w1904
                  tunnel: w1886 -> [w1943]
                  tunnel: w1905 -> [w1942]
                  tunnel: [w1941] -> w1903
                  tunnel: [w1948] -> w1902
                  tunnel: w1904 -> [w1948]
                  tunnel: [w1947] -> w1901
                  tunnel: w1903 -> [w1947]
                  tunnel: w1880 -> [w1946]
                  tunnel: w1902 -> [w1955]
                  tunnel: w1901 -> [w1954]
                  tunnel: [w1950] -> w1900
                  tunnel: [w1949] -> w1899
                  tunnel: w1900 -> [w1958]
                  tunnel: [w1958] -> w1898
                  tunnel: w1899 -> [w1957]
                  tunnel: [w1957] -> w1897
                  tunnel: w1880 -> [w1956]
                  tunnel: w1898 -> [w1962]
                  tunnel: w1897 -> [w1961]
                  frame #0 {
                    n1093 = VISA Write(VISA resource name=w1921, write buffer=w1917, error in (no error)=w1919) -> (VISA resource name out=w1920:refnum<visa-resource-name>, error out=w1918:errorcluster)  [unwired: 1 out]
                  }
                  frame #1 {
                    n1094 = Wait (ms)(milliseconds to wait=w1922) -> ()  [unwired: 1 out]
                  }
                  frame #2 {
                    n1095 = VISA Write(VISA resource name=w1927, write buffer=w1928, error in (no error)=w1926) -> (VISA resource name out=w1929:refnum<visa-resource-name>, error out=w1925:errorcluster)  [unwired: 1 out]
                  }
                  frame #3 {
                    n1096 = Wait (ms)(milliseconds to wait=w1930) -> ()  [unwired: 1 out]
                  }
                  frame #4 {
                    n1097 = VISA Write(VISA resource name=w1937, write buffer=w1935, error in (no error)=w1934) -> (VISA resource name out=w1936:refnum<visa-resource-name>, error out=w1933:errorcluster)  [unwired: 1 out]
                  }
                  frame #5 {
                    n1098 = Wait (ms)(milliseconds to wait=w1938) -> ()  [unwired: 1 out]
                  }
                  frame #6 {
                    n1099 = VISA Write(VISA resource name=w1945, write buffer=w1943, error in (no error)=w1942) -> (VISA resource name out=w1944:refnum<visa-resource-name>, error out=w1941:errorcluster)  [unwired: 1 out]
                  }
                  frame #7 {
                    n1100 = Wait (ms)(milliseconds to wait=w1946) -> ()  [unwired: 1 out]
                  }
                  frame #8 {
                    n1101 = Concatenate Strings("start ", "\r") -> (w1953:string)
                    n1102 = VISA Write(VISA resource name=w1955, write buffer=w1953, error in (no error)=w1954) -> (VISA resource name out=w1950:refnum<visa-resource-name>, error out=w1949:errorcluster)  [unwired: 1 out]
                  }
                  frame #9 {
                    n1103 = Wait (ms)(milliseconds to wait=w1956) -> ()  [unwired: 1 out]
                  }
                  frame #10 {
                    n1104 = Concatenate Strings("enter main ", "\r") -> (w1963:string)
                    n1105 = VISA Write(VISA resource name=w1962, write buffer=w1963, error in (no error)=w1961) -> (VISA resource name out=w1960:refnum<visa-resource-name>, error out=w1959:errorcluster)  [unwired: 1 out]
                    n1106 = VISA Close(VISA resource name=w1960, error in (no error)=w1959) -> ()  [unwired: 1 out]
                  }
                }
                n1107 = Concatenate Strings("enter pump1", w1896) -> (w1895:string)
                n1108 = local read "Normal \nRate (ul/hr)"() -> (w1881:dbl)
                n1109 = Concatenate Strings("set units 4 ", w1896) -> (w1892:string)
                n1110 = local read "Normal \nVolume (ul)"() -> (w1882:dbl)
                n1111 = Number To Decimal String(number=w1881) -> (decimal integer string=w1891:string)  [unwired: 1 in]
                n1112 = Concatenate Strings("set rate ", w1891, w1896) -> (w1889:string)
                n1113 = Number To Decimal String(number=w1882) -> (decimal integer string=w1887:string)  [unwired: 1 in]
                n1114 = Concatenate Strings("set volume ", w1887, w1896) -> (w1886:string)
              }
            }
          }
          event "Normal \nVolume (ul)": Value Change {
            n1115 = event-data() -> ()  [unwired: 1 in, 5 out]
            n1116 = call-poly "VISA Configure Serial Port"("VISA resource name"=w1981) -> ("VISA resource name out"=w1983:refnum<visa-resource-name>, "error out"=w1982:errorcluster)  [unwired: 13 in]
            n1117 = local read "Write Wait"() -> (w1966:i32)
            n1118 = Concatenate Strings("enter pump1", "\r") -> (w1985:string)
            n1119 = flat-sequence {
              tunnel: w1982 -> [w1995]
              tunnel: w1983 -> [w1997]
              tunnel: [w1996] -> w1975
              tunnel: [w1994] -> w1974
              tunnel: w1985 -> [w1993]
              tunnel: w1975 -> [w2000]
              tunnel: [w2000] -> w1973
              tunnel: w1974 -> [w1999]
              tunnel: [w1999] -> w1971
              tunnel: w1966 -> [w1998]
              tunnel: w1973 -> [w2004]
              tunnel: [w2005] -> w1972
              tunnel: w1971 -> [w2003]
              tunnel: [w2002] -> w1970
              tunnel: w1967 -> [w2001]
              tunnel: w1972 -> [w2008]
              tunnel: w1970 -> [w2007]
              tunnel: [w2008] -> w1992
              tunnel: [w2007] -> w1991
              tunnel: w1966 -> [w2006]
              tunnel: [w2013] -> w1990
              tunnel: [w2012] -> w1989
              tunnel: w1992 -> [w2011]
              tunnel: w1991 -> [w2010]
              tunnel: w1976 -> [w2009]
              tunnel: w1990 -> [w2016]
              tunnel: [w2016] -> w1988
              tunnel: w1989 -> [w2015]
              tunnel: [w2015] -> w1987
              tunnel: w1966 -> [w2014]
              tunnel: w1988 -> [w2020]
              tunnel: w1987 -> [w2019]
              frame #0 {
                n1120 = VISA Write(VISA resource name=w1997, write buffer=w1993, error in (no error)=w1995) -> (VISA resource name out=w1996:refnum<visa-resource-name>, error out=w1994:errorcluster)  [unwired: 1 out]
              }
              frame #1 {
                n1121 = Wait (ms)(milliseconds to wait=w1998) -> ()  [unwired: 1 out]
              }
              frame #2 {
                n1122 = VISA Write(VISA resource name=w2004, write buffer=w2001, error in (no error)=w2003) -> (VISA resource name out=w2005:refnum<visa-resource-name>, error out=w2002:errorcluster)  [unwired: 1 out]
              }
              frame #3 {
                n1123 = Wait (ms)(milliseconds to wait=w2006) -> ()  [unwired: 1 out]
              }
              frame #4 {
                n1124 = VISA Write(VISA resource name=w2011, write buffer=w2009, error in (no error)=w2010) -> (VISA resource name out=w2013:refnum<visa-resource-name>, error out=w2012:errorcluster)  [unwired: 1 out]
              }
              frame #5 {
                n1125 = Wait (ms)(milliseconds to wait=w2014) -> ()  [unwired: 1 out]
              }
              frame #6 {
                n1126 = Concatenate Strings("enter main ", "\r") -> (w2021:string)
                n1127 = VISA Write(VISA resource name=w2020, write buffer=w2021, error in (no error)=w2019) -> (VISA resource name out=w2018:refnum<visa-resource-name>, error out=w2017:errorcluster)  [unwired: 1 out]
                n1128 = VISA Close(VISA resource name=w2018, error in (no error)=w2017) -> ()  [unwired: 1 out]
              }
            }
            n1129 = Concatenate Strings("set units 4", "\r") -> (w1967:string)
            n1130 = Number To Decimal String(number="Normal \nVolume (ul)") -> (decimal integer string=w1978:string)  [unwired: 1 in]
            n1131 = Concatenate Strings("set volume", w1978, "\r") -> (w1976:string)
          }
          event "Normal \nRate (ul/hr)": Value Change {
            n1132 = event-data() -> ()  [unwired: 1 in, 5 out]
            n1133 = call-poly "VISA Configure Serial Port"("VISA resource name"=w2026) -> ("VISA resource name out"=w2034:refnum<visa-resource-name>, "error out"=w2033:errorcluster)  [unwired: 13 in]
            n1134 = local read "Write Wait"() -> (w2024:i32)
            n1135 = Concatenate Strings("enter pump1", "\r") -> (w2036:string)
            n1136 = flat-sequence {
              tunnel: w2033 -> [w2053]
              tunnel: w2034 -> [w2055]
              tunnel: [w2054] -> w2049
              tunnel: [w2052] -> w2048
              tunnel: w2036 -> [w2051]
              tunnel: w2049 -> [w2058]
              tunnel: [w2058] -> w2047
              tunnel: w2048 -> [w2057]
              tunnel: [w2057] -> w2046
              tunnel: w2024 -> [w2056]
              tunnel: w2047 -> [w2062]
              tunnel: [w2063] -> w2045
              tunnel: w2046 -> [w2061]
              tunnel: [w2060] -> w2044
              tunnel: w2027 -> [w2059]
              tunnel: w2045 -> [w2066]
              tunnel: w2044 -> [w2065]
              tunnel: [w2066] -> w2043
              tunnel: [w2065] -> w2042
              tunnel: w2024 -> [w2064]
              tunnel: [w2071] -> w2041
              tunnel: [w2070] -> w2040
              tunnel: w2043 -> [w2069]
              tunnel: w2042 -> [w2068]
              tunnel: w2030 -> [w2067]
              tunnel: w2041 -> [w2074]
              tunnel: [w2074] -> w2039
              tunnel: w2040 -> [w2073]
              tunnel: [w2073] -> w2038
              tunnel: w2024 -> [w2072]
              tunnel: w2039 -> [w2078]
              tunnel: w2038 -> [w2077]
              frame #0 {
                n1137 = VISA Write(VISA resource name=w2055, write buffer=w2051, error in (no error)=w2053) -> (VISA resource name out=w2054:refnum<visa-resource-name>, error out=w2052:errorcluster)  [unwired: 1 out]
              }
              frame #1 {
                n1138 = Wait (ms)(milliseconds to wait=w2056) -> ()  [unwired: 1 out]
              }
              frame #2 {
                n1139 = VISA Write(VISA resource name=w2062, write buffer=w2059, error in (no error)=w2061) -> (VISA resource name out=w2063:refnum<visa-resource-name>, error out=w2060:errorcluster)  [unwired: 1 out]
              }
              frame #3 {
                n1140 = Wait (ms)(milliseconds to wait=w2064) -> ()  [unwired: 1 out]
              }
              frame #4 {
                n1141 = VISA Write(VISA resource name=w2069, write buffer=w2067, error in (no error)=w2068) -> (VISA resource name out=w2071:refnum<visa-resource-name>, error out=w2070:errorcluster)  [unwired: 1 out]
              }
              frame #5 {
                n1142 = Wait (ms)(milliseconds to wait=w2072) -> ()  [unwired: 1 out]
              }
              frame #6 {
                n1143 = Concatenate Strings("enter main ", "\r") -> (w2079:string)
                n1144 = VISA Write(VISA resource name=w2078, write buffer=w2079, error in (no error)=w2077) -> (VISA resource name out=w2076:refnum<visa-resource-name>, error out=w2075:errorcluster)  [unwired: 1 out]
                n1145 = VISA Close(VISA resource name=w2076, error in (no error)=w2075) -> ()  [unwired: 1 out]
              }
            }
            n1146 = Concatenate Strings("set units 4", "\r") -> (w2027:string)
            n1147 = Number To Decimal String(number="Normal \nRate (ul/hr)") -> (decimal integer string=w2025:string)  [unwired: 1 in]
            n1148 = Concatenate Strings("set rate", w2025, "\r") -> (w2030:string)
          }
          event "Normal \nRate (ul/hr)  2": Value Change {
            n1149 = event-data() -> ()  [unwired: 1 in, 5 out]
            n1150 = call-poly "VISA Configure Serial Port"("VISA resource name"=w2084) -> ("VISA resource name out"=w2092:refnum<visa-resource-name>, "error out"=w2091:errorcluster)  [unwired: 13 in]
            n1151 = local read "Write Wait"() -> (w2082:i32)
            n1152 = Concatenate Strings("enter pump2", "\r") -> (w2094:string)
            n1153 = flat-sequence {
              tunnel: w2091 -> [w2111]
              tunnel: w2092 -> [w2113]
              tunnel: [w2112] -> w2107
              tunnel: [w2110] -> w2106
              tunnel: w2094 -> [w2109]
              tunnel: w2107 -> [w2116]
              tunnel: [w2116] -> w2105
              tunnel: w2106 -> [w2115]
              tunnel: [w2115] -> w2104
              tunnel: w2082 -> [w2114]
              tunnel: w2105 -> [w2120]
              tunnel: [w2121] -> w2103
              tunnel: w2104 -> [w2119]
              tunnel: [w2118] -> w2102
              tunnel: w2085 -> [w2117]
              tunnel: w2103 -> [w2124]
              tunnel: w2102 -> [w2123]
              tunnel: [w2124] -> w2101
              tunnel: [w2123] -> w2100
              tunnel: w2082 -> [w2122]
              tunnel: [w2129] -> w2099
              tunnel: [w2128] -> w2098
              tunnel: w2101 -> [w2127]
              tunnel: w2100 -> [w2126]
              tunnel: w2088 -> [w2125]
              tunnel: w2099 -> [w2132]
              tunnel: [w2132] -> w2097
              tunnel: w2098 -> [w2131]
              tunnel: [w2131] -> w2096
              tunnel: w2082 -> [w2130]
              tunnel: w2097 -> [w2136]
              tunnel: w2096 -> [w2135]
              frame #0 {
                n1154 = VISA Write(VISA resource name=w2113, write buffer=w2109, error in (no error)=w2111) -> (VISA resource name out=w2112:refnum<visa-resource-name>, error out=w2110:errorcluster)  [unwired: 1 out]
              }
              frame #1 {
                n1155 = Wait (ms)(milliseconds to wait=w2114) -> ()  [unwired: 1 out]
              }
              frame #2 {
                n1156 = VISA Write(VISA resource name=w2120, write buffer=w2117, error in (no error)=w2119) -> (VISA resource name out=w2121:refnum<visa-resource-name>, error out=w2118:errorcluster)  [unwired: 1 out]
              }
              frame #3 {
                n1157 = Wait (ms)(milliseconds to wait=w2122) -> ()  [unwired: 1 out]
              }
              frame #4 {
                n1158 = VISA Write(VISA resource name=w2127, write buffer=w2125, error in (no error)=w2126) -> (VISA resource name out=w2129:refnum<visa-resource-name>, error out=w2128:errorcluster)  [unwired: 1 out]
              }
              frame #5 {
                n1159 = Wait (ms)(milliseconds to wait=w2130) -> ()  [unwired: 1 out]
              }
              frame #6 {
                n1160 = Concatenate Strings("enter main ", "\r") -> (w2137:string)
                n1161 = VISA Write(VISA resource name=w2136, write buffer=w2137, error in (no error)=w2135) -> (VISA resource name out=w2134:refnum<visa-resource-name>, error out=w2133:errorcluster)  [unwired: 1 out]
                n1162 = VISA Close(VISA resource name=w2134, error in (no error)=w2133) -> ()  [unwired: 1 out]
              }
            }
            n1163 = Concatenate Strings("set units 4", "\r") -> (w2085:string)
            n1164 = Number To Decimal String(number="Normal \nRate (ul/hr)  2") -> (decimal integer string=w2083:string)  [unwired: 1 in]
            n1165 = Concatenate Strings("set rate", w2083, "\r") -> (w2088:string)
          }
          event "Normal \nVolume (ul) 2": Value Change {
            n1166 = event-data() -> ()  [unwired: 1 in, 5 out]
            n1167 = call-poly "VISA Configure Serial Port"("VISA resource name"=w2143) -> ("VISA resource name out"=w2147:refnum<visa-resource-name>, "error out"=w2148:errorcluster)  [unwired: 13 in]
            n1168 = local read "Write Wait"() -> (w2140:i32)
            n1169 = Concatenate Strings("enter pump2", "\r") -> (w2145:string)
            n1170 = flat-sequence {
              tunnel: w2148 -> [w2169]
              tunnel: w2147 -> [w2171]
              tunnel: [w2170] -> w2166
              tunnel: [w2168] -> w2165
              tunnel: w2145 -> [w2167]
              tunnel: w2166 -> [w2174]
              tunnel: [w2174] -> w2164
              tunnel: w2165 -> [w2173]
              tunnel: [w2173] -> w2163
              tunnel: w2140 -> [w2172]
              tunnel: w2164 -> [w2178]
              tunnel: [w2179] -> w2162
              tunnel: w2163 -> [w2177]
              tunnel: [w2176] -> w2161
              tunnel: w2154 -> [w2175]
              tunnel: w2162 -> [w2182]
              tunnel: w2161 -> [w2181]
              tunnel: [w2182] -> w2160
              tunnel: [w2181] -> w2159
              tunnel: w2140 -> [w2180]
              tunnel: [w2187] -> w2158
              tunnel: [w2186] -> w2157
              tunnel: w2160 -> [w2185]
              tunnel: w2159 -> [w2184]
              tunnel: w2151 -> [w2183]
              tunnel: w2158 -> [w2190]
              tunnel: [w2190] -> w2156
              tunnel: w2157 -> [w2189]
              tunnel: [w2189] -> w2155
              tunnel: w2140 -> [w2188]
              tunnel: w2156 -> [w2194]
              tunnel: w2155 -> [w2193]
              frame #0 {
                n1171 = VISA Write(VISA resource name=w2171, write buffer=w2167, error in (no error)=w2169) -> (VISA resource name out=w2170:refnum<visa-resource-name>, error out=w2168:errorcluster)  [unwired: 1 out]
              }
              frame #1 {
                n1172 = Wait (ms)(milliseconds to wait=w2172) -> ()  [unwired: 1 out]
              }
              frame #2 {
                n1173 = VISA Write(VISA resource name=w2178, write buffer=w2175, error in (no error)=w2177) -> (VISA resource name out=w2179:refnum<visa-resource-name>, error out=w2176:errorcluster)  [unwired: 1 out]
              }
              frame #3 {
                n1174 = Wait (ms)(milliseconds to wait=w2180) -> ()  [unwired: 1 out]
              }
              frame #4 {
                n1175 = VISA Write(VISA resource name=w2185, write buffer=w2183, error in (no error)=w2184) -> (VISA resource name out=w2187:refnum<visa-resource-name>, error out=w2186:errorcluster)  [unwired: 1 out]
              }
              frame #5 {
                n1176 = Wait (ms)(milliseconds to wait=w2188) -> ()  [unwired: 1 out]
              }
              frame #6 {
                n1177 = Concatenate Strings("enter main ", "\r") -> (w2195:string)
                n1178 = VISA Write(VISA resource name=w2194, write buffer=w2195, error in (no error)=w2193) -> (VISA resource name out=w2192:refnum<visa-resource-name>, error out=w2191:errorcluster)  [unwired: 1 out]
                n1179 = VISA Close(VISA resource name=w2192, error in (no error)=w2191) -> ()  [unwired: 1 out]
              }
            }
            n1180 = Concatenate Strings("set units 4", "\r") -> (w2154:string)
            n1181 = Number To Decimal String(number="Normal \nVolume (ul) 2") -> (decimal integer string=w2141:string)  [unwired: 1 in]
            n1182 = Concatenate Strings("set volume", w2141, "\r") -> (w2151:string)
          }
        }
        n1183 = node-c288() -> ()  [unwired: 1 in, 1 out]
      }
      n1184 = node-c288(w1527) -> ()  [unwired: 1 out]
    }
    frame Enabled {
      n1185 = node-c288(2 ("Processor")) -> (w2207:T11)  [unwired: 3 in]
      n1186 = timed-loop "Pump Control" {
        timing: w2207 -> [_]
        timing-out: [_] -> w2206
        tunnel: refnum<visa-resource-name> "COM5" ("VISA resource name") -> [w2209]
        stop <- w2208 stop-if-true
        n1187 = node-c288() -> ()  [unwired: 1 in, 1 out]
        n1188 = event shown="[2] \"Inject Sample\": Value Change" {
          selector: _ -> [_ _ _ _ _]
          dyn-events: _ -> [_ _ _ _ _]
          timeout: _ -> [_ _ _ _ _]
          tunnel: w2209 -> [w2215 _ w2289 w2316 w2321]
          tunnel: [_ w2287 _ _ _] -> w2208
          event "Flush Sample": Value Change {
            n1189 = event-data() -> ()  [unwired: 1 in, 5 out]
            n1190 = local read "Write Wait"() -> (w2229:i32)
            n1191 = flat-sequence {
              tunnel: [w2253] -> w2249
              tunnel: [w2252] -> w2248
              tunnel: "CLD" -> [w2251]
              tunnel: w2215 -> [w2250]
              tunnel: w2249 -> [w2256]
              tunnel: [w2256] -> w2247
              tunnel: w2248 -> [w2255]
              tunnel: [w2255] -> w2246
              tunnel: w2229 -> [w2254]
              tunnel: [w2261] -> w2245
              tunnel: [w2258] -> w2244
              tunnel: w2247 -> [w2260]
              tunnel: w2246 -> [w2259]
              tunnel: "MODVOL" -> [w2257]
              tunnel: w2245 -> [w2264]
              tunnel: [w2264] -> w2243
              tunnel: [w2263] -> w2242
              tunnel: w2244 -> [w2263]
              tunnel: w2229 -> [w2262]
              tunnel: w2243 -> [w2269]
              tunnel: [w2268] -> w2241
              tunnel: w2231 -> [w2267]
              tunnel: w2242 -> [w2266]
              tunnel: [w2265] -> w2240
              tunnel: w2241 -> [w2272]
              tunnel: [w2272] -> w2239
              tunnel: [w2271] -> w2238
              tunnel: w2240 -> [w2271]
              tunnel: w2229 -> [w2270]
              tunnel: w2239 -> [w2277]
              tunnel: [w2276] -> w2237
              tunnel: w2233 -> [w2275]
              tunnel: w2238 -> [w2274]
              tunnel: [w2273] -> w2236
              tunnel: [w2280] -> w2234
              tunnel: w2237 -> [w2280]
              tunnel: [w2279] -> w2235
              tunnel: w2236 -> [w2279]
              tunnel: w2229 -> [w2278]
              tunnel: w2235 -> [w2285]
              tunnel: w2234 -> [w2286]
              tunnel: [w2284] -> w2224
              tunnel: "RUN " -> [w2283]
              frame #0 {
                n1192 = call "Write to pump 2.vi"("String to write"=w2251, "VISA resource name"=w2250) -> ("error out"=w2252:errorcluster, "VISA resource name out"=w2253:refnum<visa-resource-name>)  [unwired: 8 in]
              }
              frame #1 {
                n1193 = Wait (ms)(milliseconds to wait=w2254) -> ()  [unwired: 1 out]
              }
              frame #2 {
                n1194 = call "Write to pump 2.vi"("error in (no error)"=w2259, "String to write"=w2257, "VISA resource name"=w2260) -> ("error out"=w2258:errorcluster, "VISA resource name out"=w2261:refnum<visa-resource-name>)  [unwired: 7 in]
              }
              frame #3 {
                n1195 = Wait (ms)(milliseconds to wait=w2262) -> ()  [unwired: 1 out]
              }
              frame #4 {
                n1196 = call "Write to pump 2.vi"("error in (no error)"=w2266, "String to write"=w2267, "VISA resource name"=w2269) -> ("error out"=w2265:errorcluster, "VISA resource name out"=w2268:refnum<visa-resource-name>)  [unwired: 7 in]
              }
              frame #5 {
                n1197 = Wait (ms)(milliseconds to wait=w2270) -> ()  [unwired: 1 out]
              }
              frame #6 {
                n1198 = call "Write to pump 2.vi"("error in (no error)"=w2274, "String to write"=w2275, "VISA resource name"=w2277) -> ("error out"=w2273:errorcluster, "VISA resource name out"=w2276:refnum<visa-resource-name>)  [unwired: 7 in]
              }
              frame #7 {
                n1199 = Wait (ms)(milliseconds to wait=w2278) -> ()  [unwired: 1 out]
              }
              frame #8 {
                w2282 = TRUE ("Inject Pump 3")
                n1200 = Tick Count (ms)() -> (millisecond timer value=→"Flush Sample Start Time":u32)
                n1201 = call "Write to pump 2.vi"("error in (no error)"=w2285, "String to write"=w2283, "VISA resource name"=w2286) -> ("error out"=w2284:errorcluster)  [unwired: 7 in, 1 out]
                n1202 = local write "Inject Sample"(w2282) -> ()
                "Flushing Sample" <- w2282
              }
            }
            n1203 = Number To Fractional String(number="Flush \nRate (ul/min)  3") -> (F-format string=w2217:string)  [unwired: 3 in]
            n1204 = String Subset(string=w2217, length (rest)=6 ("length (rest)")) -> (substring=w2216:string)  [unwired: 1 in]
            n1205 = Concatenate Strings("RAT", w2216, "UM") -> (w2231:string)
            n1206 = Divide(x="Flush\nVolume (ul)  3", y=1000.0) -> (x/y=w2222:dbl)
            n1207 = Number To Fractional String(number=w2222) -> (F-format string=w2221:string)  [unwired: 3 in]
            n1208 = Divide(x="Flush\nVolume (ul)  3", y="Flush \nRate (ul/min)  3") -> (x/y=w2212:dbl)
            n1209 = Multiply(x=w2212, y=60.0) -> (x*y=→"Sample flush time (s)":dbl)
            n1210 = String Subset(string=w2221, length (rest)=6 ("length (rest)")) -> (substring=w2220:string)  [unwired: 1 in]
            n1211 = Concatenate Strings("TGT", w2220) -> (w2233:string)
            "error out" <- w2224
          }
          event "Stop": Value Change {
            n1212 = event-data() -> ()  [unwired: 1 in, 5 out]
            n1213 = local read "Stop"() -> (w2287:bool)
          }
          event "Inject Sample": Value Change {
            n1214 = event-data() -> ()  [unwired: 1 in, 5 out]
            n1215 = case shown="True" "Inject Sample" {
              tunnel: w2289 -> [w2291 w2292]
              frame False {
                n1216 = call "Write to pump 2.vi"("String to write"="STP", "VISA resource name"=w2291) -> ()  [unwired: 8 in, 2 out]
              }
              frame True {
                n1217 = local read "Normal \nRate (ul/hr)  3"() -> (w2293:dbl)
                n1218 = Number To Fractional String(number=w2293) -> (F-format string=w2296:string)  [unwired: 3 in]
                n1219 = String Subset(string=w2296, length (rest)=6 ("length (rest)")) -> (substring=w2294:string)  [unwired: 1 in]
                n1220 = flat-sequence {
                  tunnel: "RUN " -> [w2308]
                  tunnel: [w2310] -> _
                  tunnel: [w2309] -> _
                  tunnel: w2292 -> [w2307]
                  frame #0 {
                    n1221 = call "Write to pump 2.vi"("String to write"=w2308, "VISA resource name"=w2307) -> ("error out"=w2309:errorcluster, "VISA resource name out"=w2310:refnum<visa-resource-name>)  [unwired: 8 in]
                  }
                }
                n1222 = Concatenate Strings("RAT", w2294, "UH" ("string")) -> ()  [unwired: 1 out]
                n1223 = local read "Normal \nVolume (ul) 3"() -> (w2302:dbl)
                n1224 = Divide(x=w2302, y=1000.0) -> (x/y=w2297:dbl)
                n1225 = Number To Fractional String(number=w2297) -> (F-format string=w2300:string)  [unwired: 3 in]
                n1226 = String Subset(string=w2300, length (rest)=6 ("length (rest)")) -> (substring=w2298:string)  [unwired: 1 in]
                n1227 = Concatenate Strings("TGT", w2298) -> ()  [unwired: 1 out]
              }
            }
          }
          event "Normal \nRate (ul/hr)  3": Value Change {
            n1228 = event-data() -> ()  [unwired: 1 in, 5 out]
            n1229 = Number To Fractional String(number="Normal \nRate (ul/hr)  3") -> (F-format string=w2314:string)  [unwired: 3 in]
            n1230 = String Subset(string=w2314, length (rest)=6 ("length (rest)")) -> (substring=w2312:string)  [unwired: 1 in]
            n1231 = Concatenate Strings("RAT", w2312, "UH") -> (w2315:string)
            n1232 = call "Write to pump 2.vi"("String to write"=w2315, "VISA resource name"=w2316) -> ()  [unwired: 8 in, 2 out]
          }
          event "Clear Volume": Value Change {
            n1233 = event-data() -> ()  [unwired: 1 in, 5 out]
            n1234 = Divide(x="Normal \nVolume (ul) 3", y=1000.0) -> (x/y=w2334:dbl)
            n1235 = Number To Fractional String(number=w2334) -> (F-format string=w2337:string)  [unwired: 3 in]
            n1236 = String Subset(string=w2337, length (rest)=6 ("length (rest)")) -> (substring=w2335:string)  [unwired: 1 in]
            n1237 = flat-sequence {
              tunnel: [w2344] -> w2332
              tunnel: [w2343] -> w2331
              tunnel: w2321 -> [w2342]
              tunnel: w2320 -> [w2341]
              tunnel: [w2346] -> w2329
              tunnel: [w2345] -> w2330
              tunnel: w2326 -> [w2347]
              tunnel: w2332 -> [w2346]
              tunnel: w2331 -> [w2345]
              tunnel: w2330 -> [w2351]
              tunnel: w2329 -> [w2352]
              tunnel: [w2350] -> _
              tunnel: [w2349] -> _
              tunnel: w2319 -> [w2348]
              frame #0 {
                n1238 = call "Write to pump 2.vi"("String to write"=w2341, "VISA resource name"=w2342) -> ("error out"=w2343:errorcluster, "VISA resource name out"=w2344:refnum<visa-resource-name>)  [unwired: 8 in]
              }
              frame #1 {
                n1239 = Wait (ms)(milliseconds to wait=w2347) -> ()  [unwired: 1 out]
              }
              frame #2 {
                n1240 = call "Write to pump 2.vi"("error in (no error)"=w2351, "String to write"=w2348, "VISA resource name"=w2352) -> ("error out"=w2349:errorcluster, "VISA resource name out"=w2350:refnum<visa-resource-name>)  [unwired: 7 in]
              }
            }
            n1241 = local read "Write Wait"() -> (w2326:i32)
            n1242 = Concatenate Strings("TGT", w2335) -> (w2320:string)
            n1243 = local read "Normal \nRate (ul/hr)  3"() -> (w2322:dbl)
            n1244 = local write "Clear Volume"(FALSE ("Clear Volume")) -> ()
            n1245 = Number To Fractional String(number=w2322) -> (F-format string=w2325:string)  [unwired: 3 in]
            n1246 = String Subset(string=w2325, length (rest)=6 ("length (rest)")) -> (substring=w2323:string)  [unwired: 1 in]
            n1247 = Concatenate Strings("RAT", w2323, "UH" ("string")) -> (w2319:string)
          }
        }
        n1248 = node-c288() -> ()  [unwired: 1 in, 1 out]
      }
      n1249 = node-c288(w2206) -> ()  [unwired: 1 out]
    }
  }
  n1250 = node-c288() -> (w84:T11)  [unwired: 4 in]
  n1251 = timed-loop {
    timing: w84 -> [_]
    timing-out: [_] -> w83
    stop <- w2359 stop-if-true
    n1252 = node-c288() -> ()  [unwired: 1 in, 1 out]
    n1253 = event shown="[1] \"Stop\": Value Change" {
      selector: _ -> [_ _]
      dyn-events: _ -> [_ _]
      timeout: _ -> [_ _]
      tunnel: [_ "Stop"] -> w2359
      event Timeout {
        n1254 = event-data() -> ()  [unwired: 1 in, 2 out]
      }
      event "Stop": Value Change {
        n1255 = event-data() -> ()  [unwired: 1 in, 4 out]
        n1256 = local write "Force Feedback"(FALSE ("Force Feedback")) -> ()
      }
    }
    n1257 = node-c288() -> ()  [unwired: 1 in, 1 out]
  }
  n1258 = case shown="True" w73 {
    tunnel: w78 -> [_ w2366]
    tunnel: w77 -> [_ w2365]
    tunnel: w76 -> [_ w2364]
    frame False {
    }
    frame True {
      w2368 = T14 3 items=["no dialog", "OK message", "continue or stop message", "OK message + warnings", "continue/stop + warnings"] ("type of dialog (OK msg:1)")
      w2367 = T14 3 items=["no dialog", "OK message", "continue or stop message", "OK message + warnings", "continue/stop + warnings"] ("type of dialog (OK msg:1)")
      n1259 = call <vilib>:"DAQmx Clear Task.vi"("task in"=w2366, "error in"=w2364) -> ("error out"=w2369:errorcluster)  [unwired: 13 in]
      n1260 = call <vilib>:"DAQmx Clear Task.vi"("task in"=w2365) -> ("error out"=w2370:errorcluster)  [unwired: 14 in]
      n1261 = call <vilib>:"Simple Error Handler.vi"("type of dialog (OK msg:1)"=w2368, "error in (no error)"=w2369) -> ()  [unwired: 3 in, 5 out]
      n1262 = call <vilib>:"Simple Error Handler.vi"("type of dialog (OK msg:1)"=w2367, "error in (no error)"=w2370) -> ()  [unwired: 3 in, 5 out]
    }
  }
  n1263 = case shown="\"Force Feedback\", Default" "?" {
    frame "Force Feedback", Default {
    }
    frame "Raster scan" {
    }
  }
  n1264 = node-c288(w83) -> ()  [unwired: 1 out]
  n1265 = node-c288(w86) -> ()  [unwired: 1 out]
  n1266 = local write "Pause Mouse/Mirror Connection"(FALSE ("Pause Mouse/Mirror Connection")) -> ()
  n1267 = local write "Stop"(FALSE ("Stop all")) -> ()
  "CoordinatesMousePressed" <- T4 {"Horizontal"=0, "Vertical"=0} ("Coords when pressed")
  "Deflection" <- T4 {"Horizontal"=0, "Vertical"=0} ("Coords when pressed")
